vi "TI sbRIO Main (RT).vi"() -> ()   [LabVIEW 2013]
uses:
  Type Defs/Restarts Cluster.ctl
  Type Defs/Restarts Limits.ctl
  Type Defs/Controller Names.ctl
  Controls/HMI Mom Buttons.ctl
  Controls/Alarm Config.ctl
  Controls/Alarm Definition.ctl
  Controls/Alarm Profile Config.ctl
  Type Defs/App Config.ctl
  Type Defs/Actual Starts.ctl
  Type Defs/Sequence States.ctl
  Type Defs/CAN Mode.ctl
  Type Defs/Controller List.ctl
  Controls/RPi HMI Mode.ctl
  Type Defs/Pump Data Mode.ctl
  Controls/HMI Tog Buttons.ctl
  Controls/Controller Config.ctl
  SubVIs/TenHzDataArray(Global).vi
  <vilib>/FPGAPlugInAG/sbRIO-9626/niLvFpga_Open_sbRIO-9626.vi
  <vilib>/Utility/file.llb/Write To Spreadsheet File (DBL).vi
  SubVIs/Record Period (global).vi
  SubVIs/Record Samples (global).vi
  <vilib>/FPGAPlugInAG/sbRIO-9626/niLvFpga_Reset_sbRIO-9626.vi
  <vilib>/Utility/error.llb/Error Cluster From Error Code.vi
  <vilib>/rvi/errors/niLvFpgaAdjustHostInterfaceError.vi
  <vilib>/FPGAPlugInAG/sbRIO-9626/niLvFpga_Run_sbRIO-9626.vi
  <vilib>/Utility/file.llb/Write To Spreadsheet File (string).vi
  <vilib>/rvi/interface/nirviOpenFPGA/nirviOpenFPGA.xnode
  Controls/FPGA_Reference.ctl
  FPGA/bitfiles/TI sbRIO PWM (FPGA) v1.0.lvbitx
  <vilib>/rvi/interface/nirviMethod/nirviMethod.xnode
  <vilib>/rvi/interface/nirviReadWriteControl/nirviReadWriteControl.xnode
  <vilib>/Utility/config.llb/NI_LVConfig.lvlib
  NiFpgaLv.dll
  <vilib>/NI_Real-Time Target Support.lvlib
  Real-Time/Controls/RT FIFO Mode.ctl
  <vilib>/rvi/interface/nirviCloseFPGA/nirviCloseFPGA.xnode
  Type Defs/JSON_Channel.ctl
  Type Defs/JSON_Pump.ctl
  Type Defs/JSON_Tank.ctl
  <vilib>/rvi/errors/niLvFpgaMergeErrorWithErrorCode.vi
  <vilib>/FPGAPlugInAG/sbRIO-9626/niLvFpga_Abort_sbRIO-9626.vi
  <vilib>/FPGAPlugInAG/sbRIO-9626/niLvFpga_Close_sbRIO-9626.vi
panel:
  out "HMI Mom Buttons":T1
  out "TenHzPts":i32
  in  "TenHz Path":path=path "u:/TenHz/Try.csv"
  in  "Stop":bool
  in  "Alarm Tab":enum32{"Page 1", "Page 2"}(tab)
  out "Alarm Message":string
  in  "pb.Alarm OK":bool
  in  "Monitoring Tab":enum32{"Page 1", "Page 2"}(tab)
  in  "pb.E Stop":bool
  in  "Ignition Relay":T2
  in  "Power Relay":T2
  out "Voltages":dbl[](array[numeric])=[0.015201568603515625, 0.00335693359375, 0.003021240234375, 0.12260055541992188, 0.06085968017578125, 0.052234649658203125] caption="Pump\nVoltage\n(V)" format="%#.0f"
  out "Ave. Speed":dbl=7.74131899555212 format="%.1f"
  out "Temp2":dbl caption="Tank 2 Temp (C):" format="%#_2g"
  out "Temp1":dbl caption="Tank 1 Temp (C):" format="%#_2g"
  out "Pressure":dbl[](array[numeric])=[0.015201568603515625, 0.00335693359375, 0.003021240234375, 0.12260055541992188, 0.06085968017578125, 0.052234649658203125] caption="Pressure\n(kPa)" format="%#.0f"
  out "Flow":dbl[](array[numeric])=[0.0, 0.0, 0.0, 0.125, 0.0625, 0.0625] caption="Flow\n(L/H)" format="%#.0f"
  out "PumpCurrent":dbl[](array[numeric])=[0.015201568603515625, 0.00335693359375, 0.003021240234375, 0.12260055541992188, 0.06085968017578125, 0.052234649658203125] caption="Pump\nCurrent\n(RMS)" format="%#.1g"
  out "PS Actual (V):":dbl format="%.2f"
  out "ControllerCurrent":dbl[](array[numeric])=[0.015201568603515625, 0.00335693359375, 0.003021240234375, 0.12260055541992188, 0.06085968017578125, 0.052234649658203125] caption="Controller\nCurrent\n(DC)" format="%#.1g"
  out "Speed":dbl[](array[numeric]) caption="Speed\n(RPM)" format="%#_4f"
  in  "Power Supply Cmd (V):":dbl min=0.0 max=20.0 format="%#.2f"
  in  "PressureCMD":dbl caption="Pressure Cmd (kPa):" min=0.0 max=825.0 format="%#.2f"
  in  "Manual\nCMD":dbl[](array[numeric])=[0.0, 0.0, 0.0, 0.0, 0.0, 0.0] min=0.0 max=100.0 step=0.1 format="%#.2f"
  in  "pb.Zero CMDs":bool
  out "CPU Usage:":dbl=7.74131899555212 format="%.1f"
  in  "Pumps Present":T2={"Pump 1"=TRUE, "Pump 2"=TRUE, "Pump 3"=TRUE, "Pump 4"=TRUE, "Pump 5"=TRUE, "Pump 6"=TRUE}
  out "CAN CMD":dbl
  in  "Restarts Tab":enum32{"Page 1", "Page 2"}(tab)
  in  "Restarts Limits":T3={"High Limits:"=[30, 30, 30, 30, 30, 30], "Low Limits:"=[30, 30, 30, 30, 30, 30]}
  in  "pb.Rst Tot Restarts":bool
  in  "pb.Reset Restarts":bool
  in  "Inform:":string="Input email address on Email Handler program on Lab 4 PC."
  out "Restarts Cluster":T4
  out "Client?":bool
  in  "Title Tab":enum32{"Page 1", "Page 2"}(tab)
  in  "Title":string="TI Automotive sbRIO, v2.6 (Standard Tank)"
  in  "Login":bool
  in  "Set Time Tab":enum32{"Page 1", "Page 2"}(tab)
  in  "pb.Set Time OK":bool
  in  "pb.Set Time Cancel":bool
  in  "New Time":dbl format="%<%H:%M:%S>t"
  in  "Reset Tab":enum32{"Page 1", "Page 2"}(tab)
  in  "pb.Reset OK":bool
  in  "pb.Reset Cancel":bool
  in  "pb.Stop Profile":bool
  in  "Save As Tab":enum32{"Page 1", "Page 2"}(tab)
  in  "New Profile Name:":string
  in  "pb.Save As OK":bool
  in  "pb.Save As Cancel":bool
  in  "Main Tab":enum32{"Main", "Data Stream", "Alarms"}(tab)
  in  "Profile:":string[][](table)=[["1", "2.0", "0.0", "0.0", "0.0", "67.6", "67.6", "67.6"], ["2", "1.0", "0.0", "0.0", "0.0", "10.0", "10.0", "10.0"]]
  in  "Controller Type:":T5
  in  "pb.FuelChange":bool
  in  "Tank 1 Fuel Type":string
  in  "Tank 2 Fuel Type":string
  in  "Stagger Time (ms):":i32
  in  "pb.Time Reset All":bool
  in  "CA Number:":string
  in  "Profile Name:":string(combo)="test"
  in  "pb.Save As":bool
  out "Current Step:":i32=2
  out "Step Time Left:":dbl=0.21101045608520508
  out "Cycles Completed:":u32=17
  in  "pb.Cycle Reset":bool
  out "Location:":string
  in  "pb.Run Profile":bool
  out "Elapsed Time:":dbl[](array[numeric])=[7.1, 7.1, 7.1, 458133.45, 458138.85000000003, 458126.75] format="%<%H:%M:%S>t"
  in  "pb.Resets":bool[](array[boolean])=[FALSE, FALSE, FALSE, FALSE, FALSE, FALSE]
  in  "pb.Sets":bool[](array[boolean])=[FALSE, FALSE, FALSE, FALSE, FALSE, FALSE]
  in  "Serial Numbers":T6
  in  "pb.TenHzSave":bool
  in  "Record Frequency:":i32=10 min=1 max=10 step=1
  in  "pb.Reset Cogs":bool
  in  "Cog Limits:":i32[](array[numeric])=[30, 30, 30, 30, 30, 30] min=0
  out "Cog Events:":i32[](array[numeric])
  out "Graph":dbl[](graph)
  in  "RPMhyst":fxp<+,25,6>=0.20000076293945312
  in  "Alarm Config":T7
  # "Manual Control"
  # "Monitoring"
  # "Restarts Monitor"
  # "Enter a new elapsed time."
  # "Are you sure you want to reset?"
  # "Under Development"
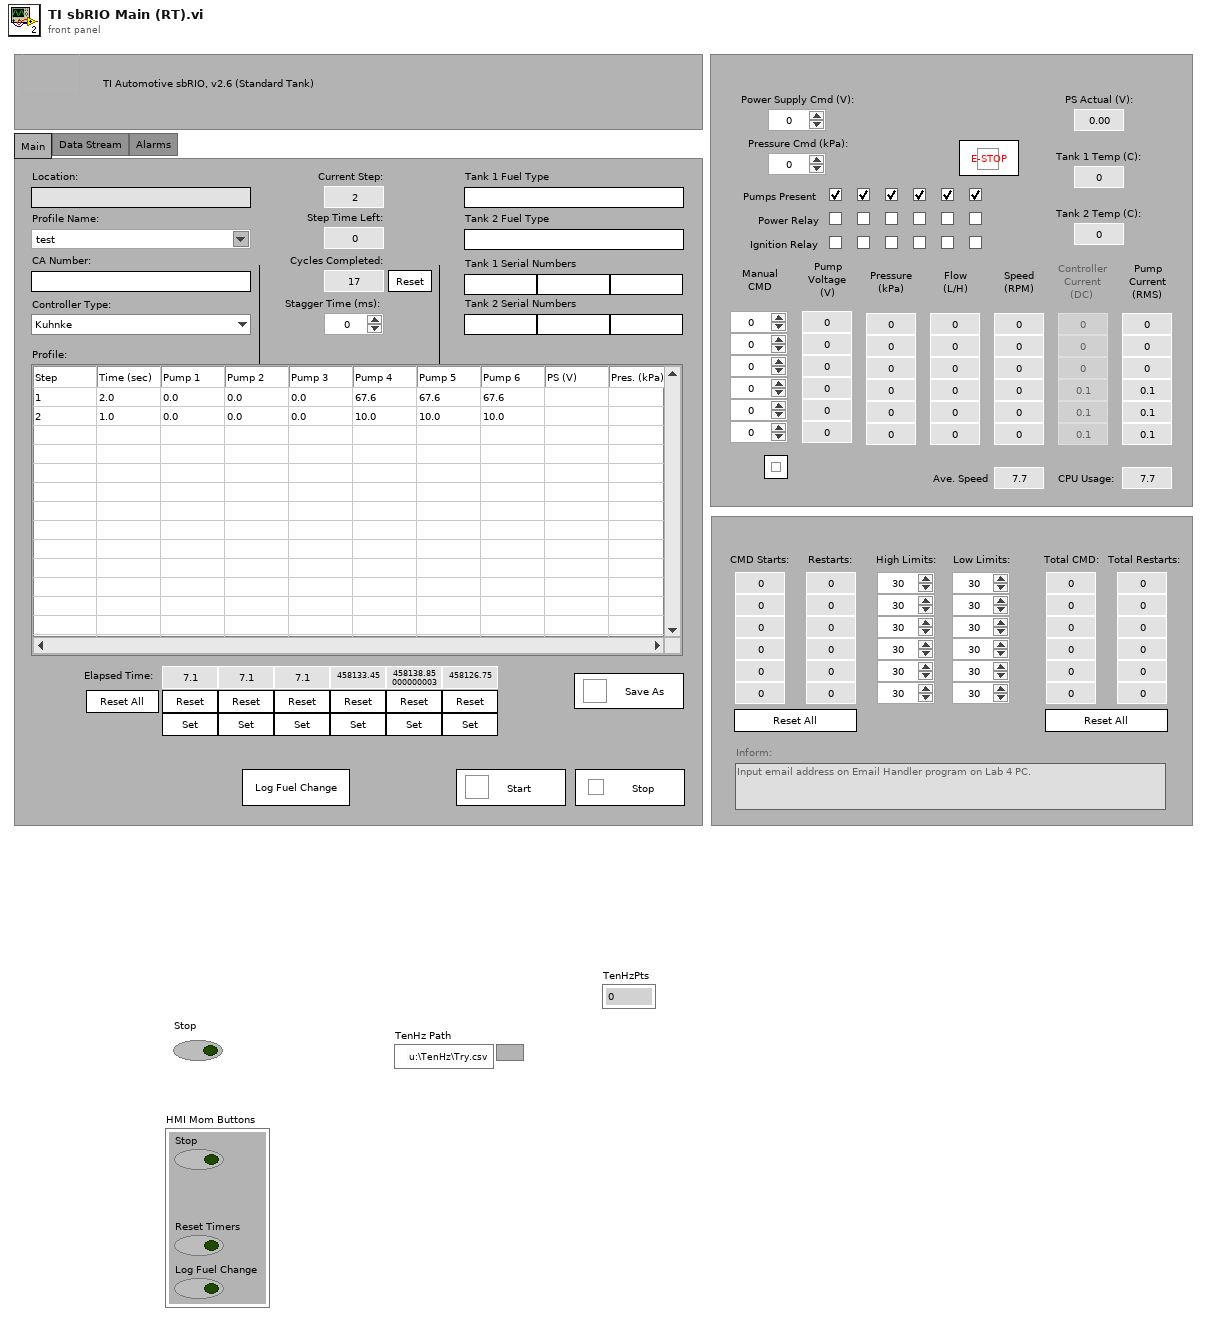
[diagram p1: front panel]
types:
  T1 = typedef "HMI Mom Buttons.ctl" = cluster{"Stop":bool, "Reset Timers":bool, "Log Fuel Change":bool}
  T2 = cluster{"Pump 1":bool, "Pump 2":bool, "Pump 3":bool, "Pump 4":bool, "Pump 5":bool, "Pump 6":bool}
  T3 = typedef "Restarts Limits.ctl" = cluster{"High Limits:":i32[], "Low Limits:":i32[]}
  T4 = typedef "Restarts Cluster.ctl" = cluster{"CMD Starts:":i32[], "Restarts:":i32[], "Total CMD:":i32[], "Total Restarts:":i32[]}
  T5 = typedef "Controller Names.ctl" = enum16{"Kuhnke", "Conti", "Hella CAN", "Helbako", "TI PWM", "PSA", "Hella DC Gas", "Hella DC Diesel", "8 Comm", "10 Comm", "8 Comm Hella", "10 Comm Hella", "8 Comm Omron", "10 Comm Omron", "8 Comm Nissan", "10 Comm Nissan"}
  T6 = cluster{"Position 1 SN":string, "Position 2 SN":string, "Position 3 SN":string, "Position 4 SN":string, "Position 5 SN":string, "Position 6 SN":string}
  T7 = typedef "Alarm Config.ctl" = cluster{"Alarms:":T8[], "Profile Sync:":T9}
  T8 = typedef "Alarm Definition.ctl" = cluster{"Description:":string, "Enabled:":bool, "Data Index:":i32, "Data Type:":string, "Low Limit:":dbl, "High Limit:":dbl, "Trip Time:":u32, "Profile Sync:":bool}
  T9 = typedef "Alarm Profile Config.ctl" = cluster{"Trip Time:":u32, "Consecutive Trips:":i32}
  T10 = typedef "RPi HMI Mode.ctl" = enum16{"Init", "Write Data", "Read from RPi", "Write to RPi"}
  T11 = typedef "Controller List.ctl" = cluster{"Controller Name":T5, "CommSeg":i32, "PWM?":bool, "Frequency":i32, "Low Command":dbl, "High Command":dbl, "Stop Command":dbl, "Command Step":dbl, "Solenoid Stop?":bool, "Controller?":bool, "Invert PWM":bool}[]
  T12 = cluster{"Controller Name":T5, "CommSeg":i32, "PWM?":bool, "Frequency":i32, "Low Command":dbl, "High Command":dbl, "Stop Command":dbl, "Command Step":dbl, "Solenoid Stop?":bool, "Controller?":bool, "Invert PWM":bool}
  T13 = typedef "CAN Mode.ctl" = enum16{"Init", "Read", "Write", "Close"}
  T14 = typedef "Sequence States.ctl" = enum16{"Main", "Init Files", "Init", "Save As", "Start Profile", "Check Step Time", "Alarm", "Run Step", "Stop Profile", "Cycle Reset", "Time Reset", "Time Reset All", "Time Set", "Tare CTs", "Save Profile", "Open Profile", "Get Profiles", "Update Screen", "Save Status", "Set Manual CMD", "Reset Restarts", "Reset Total Restarts", "Reset Cogs", "Disable Background", "Enable Background", "Get/Release Control", "Init AKLH", "Save AKLH", "Log Fuel Change", "Update Data Stream", "Init TenHz", "Read TenHz", "Remote Timer Reset", "Record Frequency Change", "Controller Change", "Get Alarms", "Init Alarms", "Save Alarms"}
  T15 = typedef "Actual Starts.ctl" = cluster{"Actual Pump Starts":i32[], "Initial Actual Starts":i32[], "Tot Act Starts":i32[], "Tot Init Act Starts":i32[]}
  T16 = typedef "App Config.ctl" = cluster{"Location":string, "Profiles Path":path, "Current Profile":string, "CA Number":string, "Cycles Completed":u32, "PWM Freq (Hz)":dbl, "Controller Type:":T5, "Inform":string, "Pumps Present":u32, "Stagger Time (ms)":i32, "Tank 1 Fuel":string, "Tank 2 Fuel":string, "Serial Numbers":cluster{"Position 1 SN":string, "Position 2 SN":string, "Poaition 3 SN":string, "Position 4 SN":string, "Position 5 SN":string, "Position 6 SN":string}, "Record TenHz":bool, "VoltCtrlRef":string, "TenHzFrequency":u32}
  T17 = cluster{"Error":errorcluster, "Profile":string[][], "App Config":T16, "Profiles":string[], "Current Step":i32, "Step Time Left":dbl, "Run Profile":bool, "Step Start Time":dbl, "Step Time":dbl, " # of Steps":i32, "Last Update":dbl, "Update Screen":bool, "Last Profile Time":dbl, "Manual CMDs":dbl[], "Client?":bool, "pb.Run Profile":bool, "pb.Resets":bool[], "pb.Sets":bool[], "Last CMDs":dbl[], "Update Profile":bool, "Elapsed Times":dbl[], "Intitial Times":dbl[], "Alarm":bool, "CT Offsets":fxp<+/-,26,7>[], "Pumps Present":cluster{"Pump 1":bool, "Pump 2":bool, "Pump 3":bool, "Pump 4":bool, "Pump 5":bool, "Pump 6":bool}, "Login":bool, "Stagger Counter":i32, "New Step":bool, "Restarts Limits":T3, "Restarts Cluster":T4, "Actual Starts":T15, "AKLH Path":path, "TenHz Path":path, "AKLH Timer":dbl, "TenHz Timer":dbl, "TenHz Active?":bool, "AKLH Last Hour":i32, "Main Tab":enum32{"Page 1", "Page 2"}, "Stop Cmd":dbl, "Tank Data":dbl[], "CogCounters":i32[], "Cog Events":i32[], "Voltage Enable":bool, "Cog Limits:":i32[], "TenHz Day":i32, "Controller":cluster{"Controller Name":T5, "CommSeg":i32, "PWM?":bool, "Frequency":i32, "Low Command":dbl, "High Command":dbl, "Stop Command":dbl, "Command Step":dbl, "Solenoid Stop?":bool, "Controller?":bool, "Invert PWM":bool}, "PS CMD":dbl, "Press CMD":dbl, "Temp CMD":dbl, "Power Relay":cluster{"Pump 1":bool, "Pump 2":bool, "Pump 3":bool, "Pump 4":bool, "Pump 5":bool, "Pump 6":bool}, "Ignition Relay":cluster{"Pump 1":bool, "Pump 2":bool, "Pump 3":bool, "Pump 4":bool, "Pump 5":bool, "Pump 6":bool}, "Controller List":T11, "Alarm Config":T7, "Alarm Config Path":path, "Trip Counters":i32[], "Previous Times":u32[], "Alarm Message":string, "Restart Alarm":bool, "Prev ON Times":u32[]}
  T18 = typedef "FPGA_Reference.ctl" = refnum<k20>
  T19 = typedef "HMI Cluster.ctl" = cluster{"Error":errorcluster, "COM Ref":refnum<visa-resource-name>, "Pump Data":T20, "Tank Data":cluster{"PS Actual (V):":dbl, "Temp1":dbl, "Temp2":dbl}, "Power Relays":cluster{"Pump 1":bool, "Pump 2":bool, "Pump 3":bool, "Pump 4":bool, "Pump 5":bool, "Pump 6":bool}, "Pump CMDs":dbl[], "HMI Header":T21, "Tank CMDs":T22, "HMI Tog Buttons":T23, "In Test":bool, "HMI Command":bool, "HMI Mom Buttons":T1, "Controller Config":T24}
  T20 = typedef "Pump Data.ctl" = cluster{"Voltages":dbl[], "PumpCurrent":dbl[], "Speed":dbl[], "ControllerCurrent":dbl[], "Pressure":dbl[], "Flow":dbl[], "Elapsed Time:":dbl[]}
  T21 = typedef "HMI Header.ctl" = cluster{"Line 1":string, "Line 2":string, "Line 3":string}
  T22 = typedef "Tank CMDs.ctl" = cluster{"PS CMD":dbl, "Press CMD":dbl, "Temp CMD":dbl}
  T23 = typedef "HMI Tog Buttons.ctl" = cluster{"Start Test":bool, "Toggle Spare 1":bool, "Toggle Spare 2":bool, "Toggle Spare 3":bool, "Toggle Spare 4":bool, "Toggle Spare 5":bool}
  T24 = typedef "Controller Config.ctl" = cluster{"Controller List":string, "Controller Type:":T5, "CMD Max":i32, "CMD Inc":i32}
  T25 = typedef "RT FIFO Mode.ctl" = enum16{"Create", "Write", "Read", "Delete"}
  T26 = typedef "Pump Data Mode.ctl" = enum16{"Read", "Write Data", "Write Cal"}
  T27 = enum8{"Enabled", "Disabled", "Disabled and Grayed Out"}
  T28 = typedef "JSON_Tank.ctl" = cluster{"number":u16, "building":string, "room":string, "ipAddress":string, "profileName":string, "caNumber":string, "ctrlType":string, "mode":string, "channels":T29[], "pumps":T30[]}
  T29 = typedef "JSON_Channel.ctl" = cluster{"name":string, "tag":string, "data":string, "type":string, "unit":string}
  T30 = typedef "JSON_Pump.ctl" = cluster{"position":u8, "enabled":bool, "command":string, "channels":T29[], "elapsedTime":string}
  T31 = cluster{"Position 1 SN":string, "Position 2 SN":string, "Poaition 3 SN":string, "Position 4 SN":string, "Position 5 SN":string, "Position 6 SN":string}
  T32 = typedef "Test Action.ctl" = enum16{"Idle", "Start", "Stop", "Pump Cmd", "Pump 1 Enable", "Pump 2 Enable", "Pump 3 Enable", "Pump 4 Enable", "Pump 5 Enable", "Pump 6 Enable", "Timer 1 Reset", "Timer 2 Reset", "Timer 3 Reset", "Timer 4 Reset", "Timer 5 Reset", "Timer 6 Reset"}
  T33 = cluster{"Boolean array[0]":bool, "Boolean array[1]":bool, "Boolean array[2]":bool, "Boolean array[3]":bool, "Boolean array[4]":bool, "Boolean array[5]":bool}
  T34 = typedef "LVDateTimeRec.ctl" = cluster{"fractional second":dbl, "second":i32, "minute":i32, "hour":i32, "day of month":i32, "month":i32, "year":i32, "day of week":i32, "day of year":i32, "DST":i32}
  T35 = typedef "NI_LVConfig.lvlib/Config Data RefNum.ctl" = refnum<k1>
  T36 = cluster{"PS Actual (V):":dbl, "Temp1":dbl, "Temp2":dbl}
  T37 = cluster{"Location":string, "Current Profile":string, "CA Number":string}
  T38 = cluster{"PS CMD":dbl, "Press CMD":dbl, "Temp CMD":dbl}
  T39 = typedef "LVRemotePanelConnectionsTypeDef.ctl" = cluster{"VI Name":string, "Remote":string, "UserName":string, "Port":i32, "Status":enum32{"Viewing", "Waiting For Control", "Controlling"}, "Create Time":timestamp, "Status Time":timestamp, "Control End Time":timestamp}[]
  T40 = typedef "NI_Real-Time Target Support.lvlib/RT CPU Load.ctl" = cluster{"Total (%)":dbl, "Time Critical (%)":dbl, "Timed Structures (%)":dbl, "High (%)":dbl, "Above Normal (%)":dbl, "Normal (%)":dbl, "Background (%)":dbl, "Idle (%)":dbl, "ISR (%)":dbl}
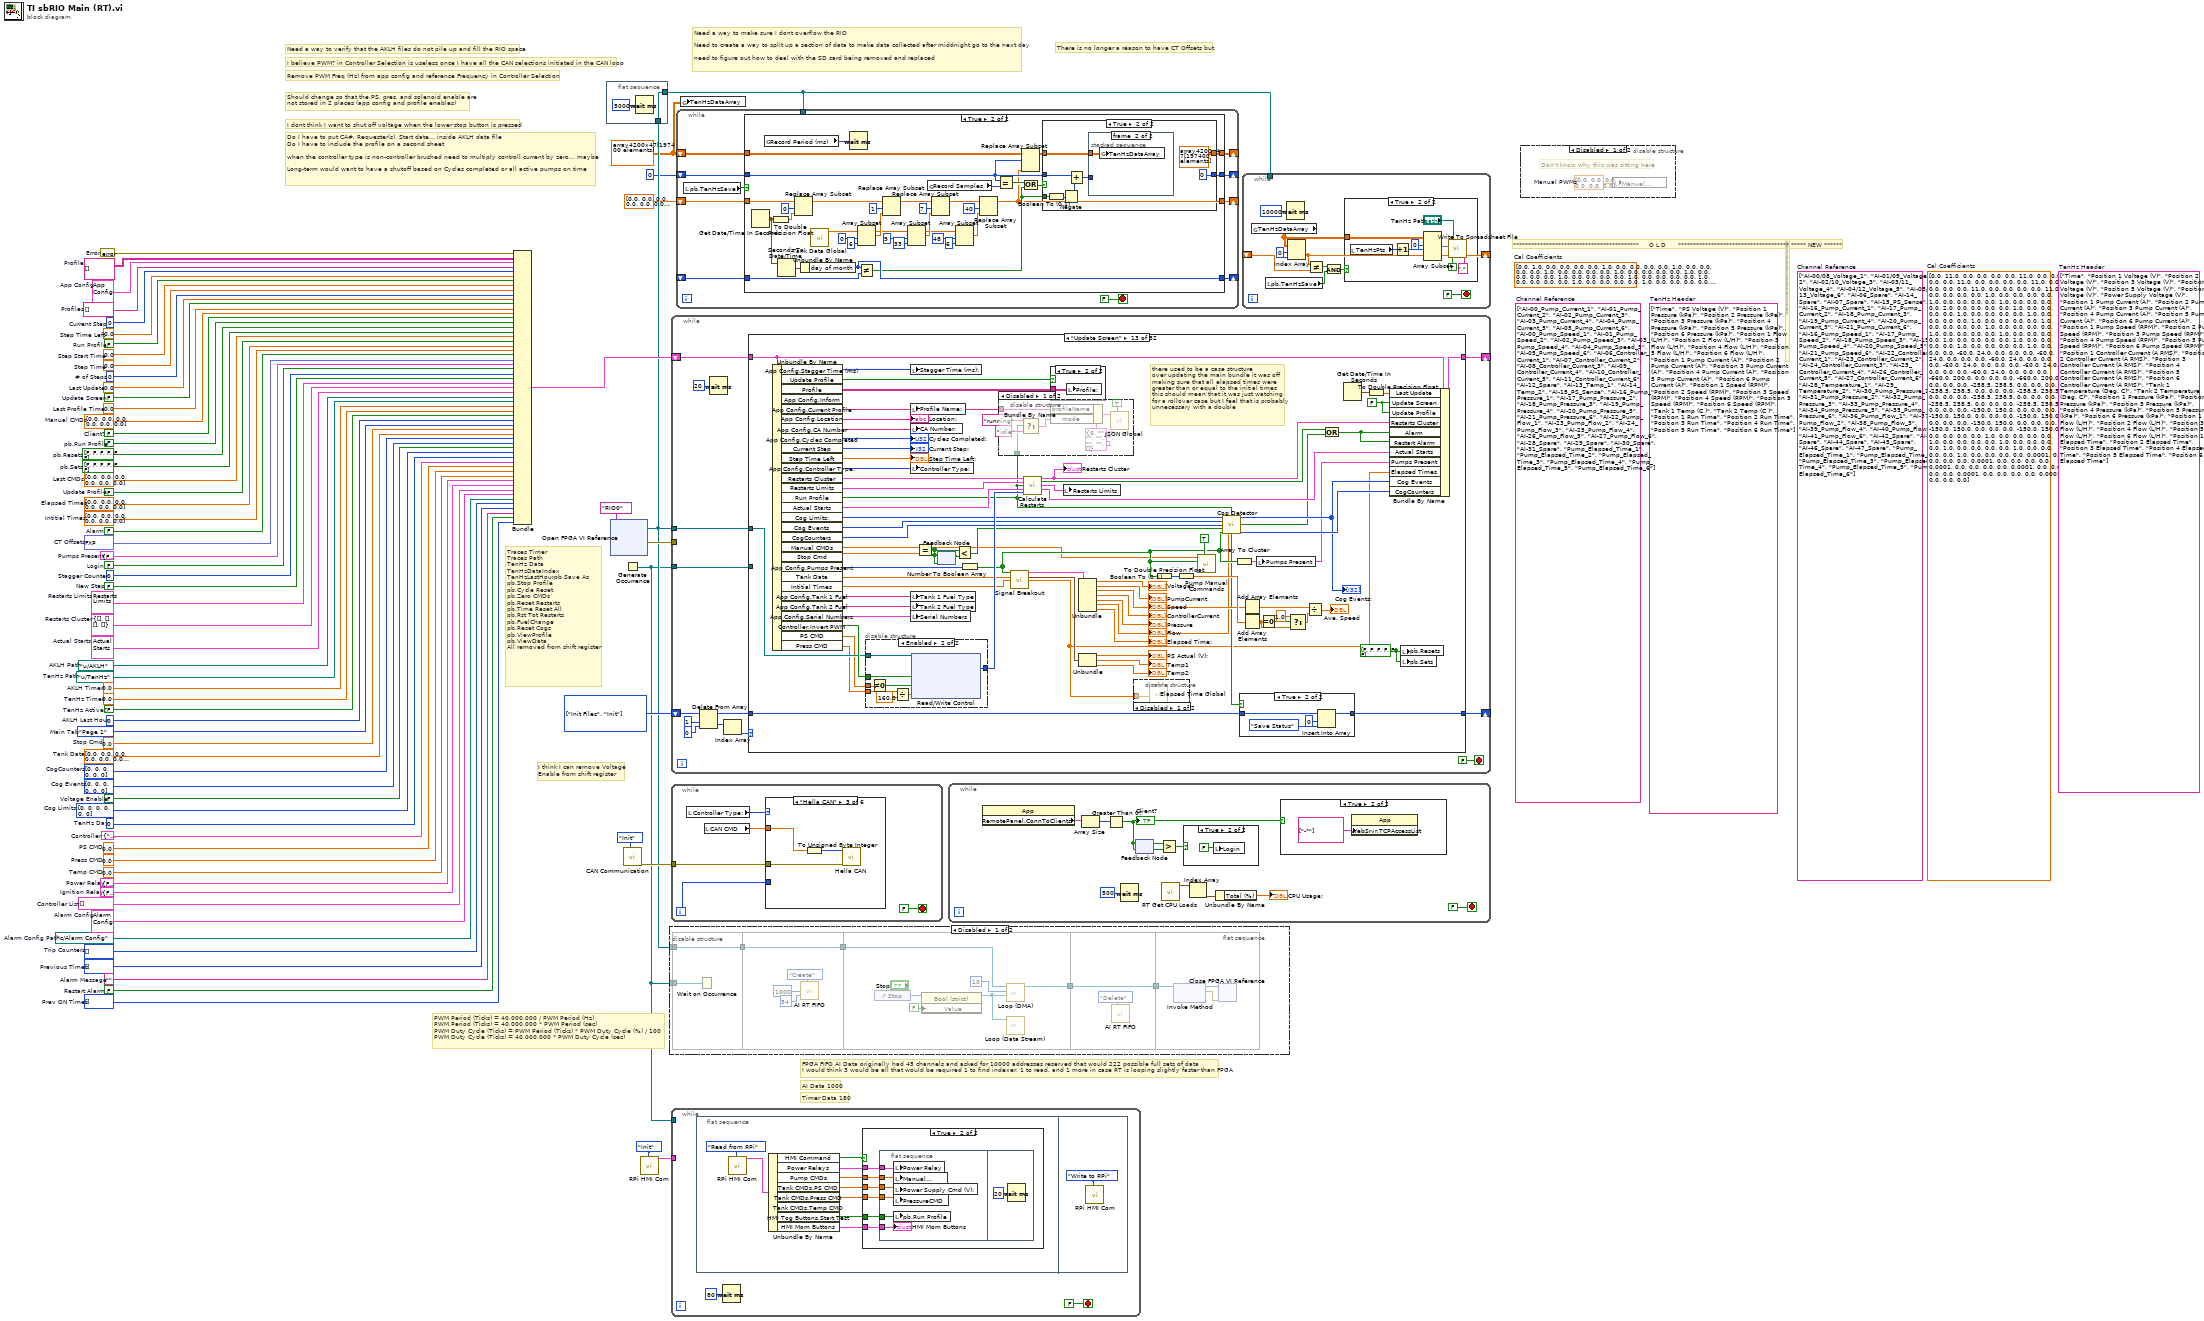
[diagram p0: block diagram]
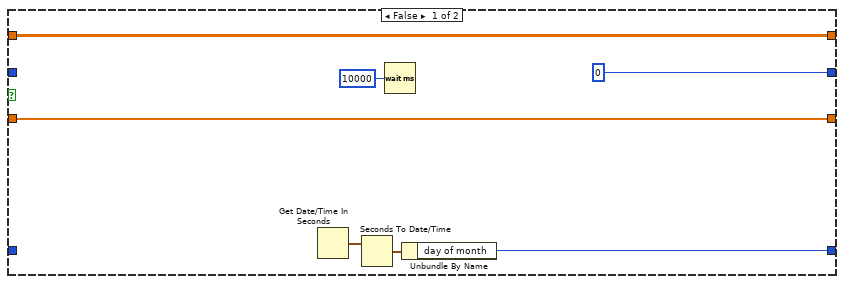
[diagram p3: hidden frame]
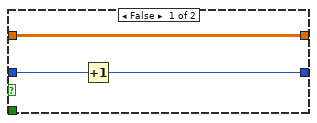
[diagram p4: hidden frame]
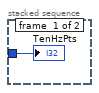
[diagram p5: hidden frame]
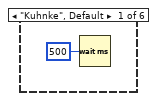
[diagram p8: hidden frame]
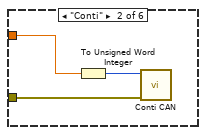
[diagram p9: hidden frame]
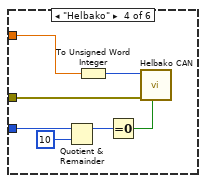
[diagram p10: hidden frame]
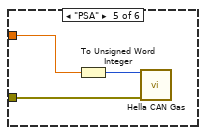
[diagram p11: hidden frame]
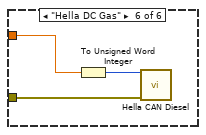
[diagram p12: hidden frame]
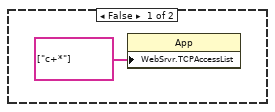
[diagram p13: hidden frame]
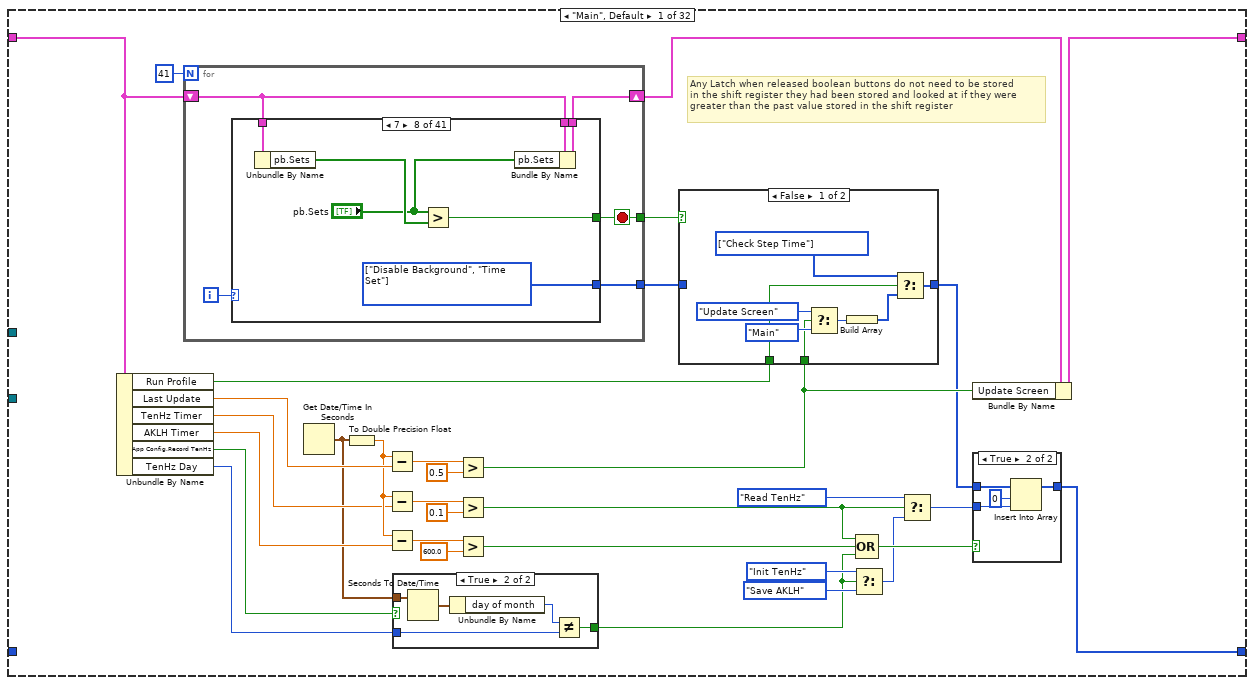
[diagram p16: hidden frame]
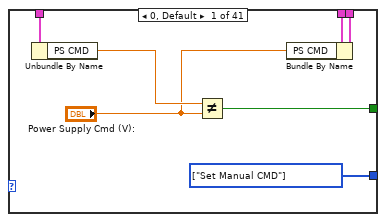
[diagram p19: hidden frame]
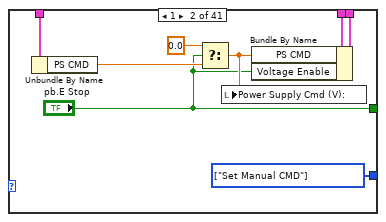
[diagram p20: hidden frame]
diagram:
  w1 = dbl[][] array4200x47[197400 elements]
  w7 = u32[] []  # Prev ON Times
  w8 = FALSE  # Restart Alarm
  w9 = ""  # Alarm Message
  w10 = u32[] []  # Previous Times
  w11 = i32[] []  # Trip Counters
  w12 = path "c:/Alarm Config"  # Alarm Config Path
  w13 = T7 {"Alarms:"=[{"Description:"="", "Enabled:"=FALSE, "Data Index:"=0, "Data Type:"="", "Low Limit:"=0.0, "High Limit:"=0.0, "Trip Time:"=0, "Profile Sync:"=FALSE}, {"Description:"="", "Enabled:"=FALSE, "Data Index:"=0, "Data Type:"="", "Low Limit:"=0.0, "High Limit:"=0.0, "Trip Time:"=0, "Profile Sync:"=FALSE}, {"Description:"="", "Enabled:"=FALSE, "Data Index:"=0, "Data Type:"="", "Low Limit:"=0.0, "High Limit:"=0.0, "Trip Time:"=0, "Profile Sync:"=FALSE}, {"Description:"="", "Enabled:"=FALSE, "Data Index:"=0, "Data Type:"="", "Low Limit:"=0.0, "High Limit:"=0.0, "Trip Time:"=0, "Profile Sync:"=FALSE}, {"Description:"="", "Enabled:"=FALSE, "Data Index:"=0, "Data Type:"="", "Low Limit:"=0.0, "High Limit:"=0.0, "Trip Time:"=0, "Profile Sync:"=FALSE}, {"Description:"="", "Enabled:"=FALSE, "Data Index:"=0, "Data Type:"="", "Low Limit:"=0.0, "High Limit:"=0.0, "Trip Time:"=0, "Profile Sync:"=FALSE}, {"Description:"="", "Enabled:"=FALSE, "Data Index:"=0, "Data Type:"="", "Low Limit:"=0.0, "High Limit:"=0.0, "Trip Time:"=0, "Profile Sync:"=FALSE}, {"Description:"="", "Enabled:"=FALSE, "Data Index:"=0, "Data Type:"="", "Low Limit:"=0.0, "High Limit:"=0.0, "Trip Time:"=0, "Profile Sync:"=FALSE}], "Profile Sync:"={"Trip Time:"=0, "Consecutive Trips:"=0}}  # Alarm Config
  w14 = T11 []  # Controller List
  w15 = T12 {"Controller Name"=enum."Kuhnke", "CommSeg"=2, "PWM?"=TRUE, "Frequency"=100, "Low Command"=10.0, "High Command"=100.0, "Stop Command"=10.0, "Command Step"=0.1, "Solenoid Stop?"=FALSE, "Controller?"=TRUE, "Invert PWM"=FALSE}  # Controller
  w17 = T2 {"Pump 1"=FALSE, "Pump 2"=FALSE, "Pump 3"=FALSE, "Pump 4"=FALSE, "Pump 5"=FALSE, "Pump 6"=FALSE}  # Ignition Relay
  w18 = T2 {"Pump 1"=FALSE, "Pump 2"=FALSE, "Pump 3"=FALSE, "Pump 4"=FALSE, "Pump 5"=FALSE, "Pump 6"=FALSE}  # Power Relay
  w19 = 0.0  # Temp CMD
  w20 = 0.0  # Press CMD
  w21 = 0.0  # PS CMD
  (unwired) string[] ["Time", "Position 1 Voltage (V)", "Position 2 Voltage (V)", "Position 3 Voltage (V)", "Position 4 Voltage (V)", "Position 5 Voltage (V)", "Position 6 Voltage (V)", "Power Supply Voltage (V)", "Position 1 Pump Current (A)", "Position 2 Pump Current (A)", "Position 3 Pump Current (A)", "Position 4 Pump Current (A)", "Position 5 Pump Current (A)", "Position 6 Pump Current (A)", "Position 1 Pump Speed (RPM)", "Position 2 Pump Speed (RPM)", "Position 3 Pump Speed (RPM)", "Position 4 Pump Speed (RPM)", "Position 5 Pump Speed (RPM)", "Position 6 Pump Speed (RPM)", "Position 1 Controller Current (A RMS)", "Position 2 Controller Current (A RMS)", "Position 3 Controller Current (A RMS)", "Position 4 Controller Current (A RMS)", "Position 5 Controller Current (A RMS)", "Position 6 Controller Current (A RMS)", "Tank 1 Temperature (Deg. C)", "Tank 2 Temperature (Deg. C)", "Position 1 Pressure (kPa)", "Position 2 Pressure (kPa)", "Position 3 Pressure (kPa)", "Position 4 Pressure (kPa)", "Position 5 Pressure (kPa)", "Position 6 Pressure (kPa)", "Position 1 Flow (L/H)", "Position 2 Flow (L/H)", "Position 3 Flow (L/H)", "Position 4 Flow (L/H)", "Position 5 Flow (L/H)", "Position 6 Flow (L/H)", "Position 1 Elapsed Time", "Position 2 Elapsed Time", "Position 3 Elapsed Time", "Position 4 Elapsed Time", "Position 5 Elapsed Time", "Position 6 Elapsed Time"]  # TenHz Header
  (unwired) dbl[][] [[0.0, 11.0, 0.0, 0.0, 0.0], [0.0, 11.0, 0.0, 0.0, 0.0], [0.0, 11.0, 0.0, 0.0, 0.0], [0.0, 11.0, 0.0, 0.0, 0.0], [0.0, 11.0, 0.0, 0.0, 0.0], [0.0, 11.0, 0.0, 0.0, 0.0], [0.0, 1.0, 0.0, 0.0, 0.0], [0.0, 1.0, 0.0, 0.0, 0.0], [0.0, 1.0, 0.0, 0.0, 0.0], [0.0, 2.0, 0.0, 0.0, 0.0], [0.0, 1.0, 0.0, 0.0, 0.0], [0.0, 1.0, 0.0, 0.0, 0.0], [0.0, 1.0, 0.0, 0.0, 0.0], [0.0, 1.0, 0.0, 0.0, 0.0], [0.0, 1.0, 0.0, 0.0, 0.0], [0.0, 1.0, 0.0, 0.0, 0.0], [0.0, 1.0, 0.0, 0.0, 0.0], [0.0, 1.0, 0.0, 0.0, 0.0], [0.0, 1.0, 0.0, 0.0, 0.0], [0.0, 1.0, 0.0, 0.0, 0.0], [0.0, 1.0, 0.0, 0.0, 0.0], [0.0, 1.0, 0.0, 0.0, 0.0], [-60.0, 24.0, 0.0, 0.0, 0.0], [-60.0, 24.0, 0.0, 0.0, 0.0], [-60.0, 24.0, 0.0, 0.0, 0.0], [-60.0, 24.0, 0.0, 0.0, 0.0], [-60.0, 24.0, 0.0, 0.0, 0.0], [-60.0, 24.0, 0.0, 0.0, 0.0], [-660.0, 200.0, 0.0, 0.0, 0.0], [-660.0, 200.0, 0.0, 0.0, 0.0], [-258.5, 258.5, 0.0, 0.0, 0.0], [-258.5, 258.5, 0.0, 0.0, 0.0], [-258.5, 258.5, 0.0, 0.0, 0.0], [-258.5, 258.5, 0.0, 0.0, 0.0], [-258.5, 258.5, 0.0, 0.0, 0.0], [-258.5, 258.5, 0.0, 0.0, 0.0], [-150.0, 150.0, 0.0, 0.0, 0.0], [-150.0, 150.0, 0.0, 0.0, 0.0], [-150.0, 150.0, 0.0, 0.0, 0.0], [-150.0, 150.0, 0.0, 0.0, 0.0], [-150.0, 150.0, 0.0, 0.0, 0.0], [-150.0, 150.0, 0.0, 0.0, 0.0], [0.0, 1.0, 0.0, 0.0, 0.0], [0.0, 1.0, 0.0, 0.0, 0.0], [0.0, 1.0, 0.0, 0.0, 0.0], [0.0, 1.0, 0.0, 0.0, 0.0], [0.0, 1.0, 0.0, 0.0, 0.0], [0.0, 1.0, 0.0, 0.0, 0.0], [0.0, 0.0001, 0.0, 0.0, 0.0], [0.0, 0.0001, 0.0, 0.0, 0.0], [0.0, 0.0001, 0.0, 0.0, 0.0], [0.0, 0.0001, 0.0, 0.0, 0.0], [0.0, 0.0001, 0.0, 0.0, 0.0], [0.0, 0.0001, 0.0, 0.0, 0.0]]  # Cal Coefficients
  (unwired) dbl[][] [[0.0, 1.0, 0.0, 0.0, 0.0], [0.0, 1.0, 0.0, 0.0, 0.0], [0.0, 1.0, 0.0, 0.0, 0.0], [0.0, 1.0, 0.0, 0.0, 0.0], [0.0, 1.0, 0.0, 0.0, 0.0], [0.0, 1.0, 0.0, 0.0, 0.0], [0.0, 1.0, 0.0, 0.0, 0.0], [0.0, 1.0, 0.0, 0.0, 0.0], [0.0, 1.0, 0.0, 0.0, 0.0], [0.0, 1.0, 0.0, 0.0, 0.0], [0.0, 1.0, 0.0, 0.0, 0.0], [0.0, 1.0, 0.0, 0.0, 0.0], [-60.0, 24.0, 0.0, 0.0, 0.0], [-60.0, 24.0, 0.0, 0.0, 0.0], [-60.0, 24.0, 0.0, 0.0, 0.0], [-60.0, 24.0, 0.0, 0.0, 0.0], [-60.0, 24.0, 0.0, 0.0, 0.0], [-60.0, 24.0, 0.0, 0.0, 0.0], [0.0, 1.0, 0.0, 0.0, 0.0], [-660.0, 200.0, 0.0, 0.0, 0.0], [-660.0, 200.0, 0.0, 0.0, 0.0], [0.0, 2.0, 0.0, 0.0, 0.0], [-258.5, 258.5, 0.0, 0.0, 0.0], [-258.5, 258.5, 0.0, 0.0, 0.0], [-258.5, 258.5, 0.0, 0.0, 0.0], [-258.5, 258.5, 0.0, 0.0, 0.0], [-258.5, 258.5, 0.0, 0.0, 0.0], [-258.5, 258.5, 0.0, 0.0, 0.0], [-150.0, 150.0, 0.0, 0.0, 0.0], [-150.0, 150.0, 0.0, 0.0, 0.0], [-150.0, 150.0, 0.0, 0.0, 0.0], [-150.0, 150.0, 0.0, 0.0, 0.0], [-150.0, 150.0, 0.0, 0.0, 0.0], [-150.0, 150.0, 0.0, 0.0, 0.0], [0.0, 1.0, 0.0, 0.0, 0.0], [0.0, 1.0, 0.0, 0.0, 0.0], [0.0, 1.0, 0.0, 0.0, 0.0], [0.0, 1.0, 0.0, 0.0, 0.0], [0.0, 0.0001, 0.0, 0.0, 0.0], [0.0, 0.0001, 0.0, 0.0, 0.0], [0.0, 0.0001, 0.0, 0.0, 0.0], [0.0, 0.0001, 0.0, 0.0, 0.0], [0.0, 0.0001, 0.0, 0.0, 0.0], [0.0, 0.0001, 0.0, 0.0, 0.0]]  # Cal Coefficients
  (unwired) string[] ["AI-00/08_Voltage_1", "AI-01/09_Voltage_2", "AI-02/10_Voltage_3", "AI-03/11_Voltage_4", "AI-04/12_Voltage_5", "AI-05/13_Voltage_6", "AI-06_Spare", "AI-14_Spare", "AI-07_Spare", "AI-15_PS_Sense", "AI-16_Pump_Current_1", "AI-17_Pump_Current_2", "AI-18_Pump_Current_3", "AI-19_Pump_Current_4", "AI-20_Pump_Current_5", "AI-21_Pump_Current_6", "AI-16_Pump_Speed_1", "AI-17_Pump_Speed_2", "AI-18_Pump_Speed_3", "AI-19_Pump_Speed_4", "AI-20_Pump_Speed_5", "AI-21_Pump_Speed_6", "AI-22_Controller_Current_1", "AI-23_Controller_Current_2", "AI-24_Controller_Current_3", "AI-25_Controller_Current_4", "AI-26_Controller_Current_5", "AI-27_Controller_Current_6", "AI-28_Temperature_1", "AI-29_Temperature_2", "AI-30_Pump_Pressure_1", "AI-31_Pump_Pressure_2", "AI-32_Pump_Pressure_3", "AI-33_Pump_Pressure_4", "AI-34_Pump_Pressure_5", "AI-35_Pump_Pressure_6", "AI-36_Pump_Flow_1", "AI-37_Pump_Flow_2", "AI-38_Pump_Flow_3", "AI-39_Pump_Flow_4", "AI-40_Pump_Flow_5", "AI-41_Pump_Flow_6", "AI-42_Spare", "AI-43_Spare", "AI-44_Spare", "AI-45_Spare", "AI-46_Spare", "AI-47_Spare", "Pump_Elapsed_Time_1", "Pump_Elapsed_Time_2", "Pump_Elapsed_Time_3", "Pump_Elapsed_Time_4", "Pump_Elapsed_Time_5", "Pump_Elapsed_Time_6"]  # Channel Reference
  (unwired) string[] ["Time", "PS Voltage (V)", "Position 1 Pressure (kPa)", "Position 2 Pressure (kPa)", "Position 3 Pressure (kPa)", "Position 4 Pressure (kPa)", "Position 5 Pressure (kPa)", "Position 6 Pressure (kPa)", "Position 1 Flow (L/H)", "Position 2 Flow (L/H)", "Position 3 Flow (L/H)", "Position 4 Flow (L/H)", "Position 5 Flow (L/H)", "Position 6 Flow (L/H)", "Position 1 Pump Current (A)", "Position 2 Pump Current (A)", "Position 3 Pump Current (A)", "Position 4 Pump Current (A)", "Position 5 Pump Current (A)", "Position 6 Pump Current (A)", "Position 1 Speed (RPM)", "Position 2 Speed (RPM)", "Position 3 Speed (RPM)", "Position 4 Speed (RPM)", "Position 5 Speed (RPM)", "Position 6 Speed (RPM)", "Tank 1 Temp (C )", "Tank 2 Temp (C )", "Position 1 Run Time", "Position 2 Run Time", "Position 3 Run Time", "Position 4 Run Time", "Position 5 Run Time", "Position 6 Run Time"]  # TenHz Header
  w27 = 0  # TenHz Day
  w28 = i32[] [0, 0, 0, 0, 0, 0]  # Cog Limits:
  w29 = FALSE  # Voltage Enable
  w30 = i32[] [0, 0, 0, 0, 0, 0]  # Cog Events
  w31 = i32[] [0, 0, 0, 0, 0, 0]  # CogCounters
  w32 = dbl[] [0.0, 0.0, 0.0, 0.0, 0.0, 0.0, 0.0, 0.0, 0.0, 0.0, 0.0, 0.0, 0.0, 0.0, 0.0, 0.0, 0.0, 0.0, 0.0, 0.0, 0.0, 0.0, 0.0, 0.0, 0.0, 0.0, 0.0, 0.0, 0.0, 0.0, 0.0, 0.0, 0.0, 0.0, 0.0, 0.0, 0.0, 0.0, 0.0, 0.0, 0.0, 0.0, 0.0, 0.0, 0.0, 0.0, 0.0, 0.0, 0.0, 0.0, 0.0, 0.0, 0.0, 0.0]  # Tank Data
  (unwired) string[] ["AI-00_Pump_Current_1", "AI-01_Pump_Current_2", "AI-02_Pump_Current_3", "AI-03_Pump_Current_4", "AI-04_Pump_Current_5", "AI-05_Pump_Current_6", "AI-00_Pump_Speed_1", "AI-01_Pump_Speed_2", "AI-02_Pump_Speed_3", "AI-03_Pump_Speed_4", "AI-04_Pump_Speed_5", "AI-05_Pump_Speed_6", "AI-06_Controller_Current_1", "AI-07_Controller_Current_2", "AI-08_Controller_Current_3", "AI-09_Controller_Current_4", "AI-10_Controller_Current_5", "AI-11_Controller_Current_6", "AI-12_Spare", "AI-13_Temp_1", "AI-14_Temp_2", "AI-15_PS_Sense", "AI-16_Pump_Pressure_1", "AI-17_Pump_Pressure_2", "AI-18_Pump_Pressure_3", "AI-19_Pump_Pressure_4", "AI-20_Pump_Pressure_5", "AI-21_Pump_Pressure_6", "AI-22_Pump_Flow_1", "AI-23_Pump_Flow_2", "AI-24_Pump_Flow_3", "AI-25_Pump_Flow_4", "AI-26_Pump_Flow_5", "AI-27_Pump_Flow_6", "AI-28_Spare", "AI-29_Spare", "AI-30_Spare", "AI-31_Spare", "Pump_Elapsed_Time_1", "Pump_Elapsed_Time_2", "Pump_Elapsed_Time_3", "Pump_Elapsed_Time_4", "Pump_Elapsed_Time_5", "Pump_Elapsed_Time_6"]  # Channel Reference
  w33 = 0.0  # Stop Cmd
  w34 = enum32{"Page 1", "Page 2"}."Page 1"  # Main Tab
  w35 = 0  # AKLH Last Hour
  w36 = FALSE  # TenHz Active?
  w37 = 0.0  # TenHz Timer
  w38 = 0.0  # AKLH Timer
  w39 = path "u:/TenHz"  # TenHz Path
  w40 = path "u:/AKLH"  # AKLH Path
  w41 = fxp<+/-,26,7>[] [0.0, 0.0, 0.0, 0.0, 0.0, 0.0]  # CT Offsets
  w42 = T14[] [enum."Init Files", enum."Init"] items=["Main", "Init Files", "Init", "Save As", "Start Profile", "Check Step Time", "Alarm", "Run Step", "Stop Profile", "Cycle Reset", "Time Reset", "Time Reset All", "Time Set", "Tare CTs", "Save Profile", "Open Profile", "Get Profiles", "Update Screen", "Save Status", "Set Manual CMD", "Reset Restarts", "Reset Total Restarts", "Reset Cogs", "Disable Background", "Enable Background", "Get/Release Control", "Init AKLH", "Save AKLH", "Log Fuel Change", "Update Data Stream", "Init TenHz", "Read TenHz", "Remote Timer Reset", "Record Frequency Change", "Controller Change", "Get Alarms", "Init Alarms", "Save Alarms"]
  w44 = T15 {"Actual Pump Starts"=[0, 0, 0, 0, 0, 0], "Initial Actual Starts"=[0, 0, 0, 0, 0, 0], "Tot Act Starts"=[0, 0, 0, 0, 0, 0], "Tot Init Act Starts"=[0, 0, 0, 0, 0, 0]}  # Actual Starts
  w45 = T4 {"CMD Starts:"=[], "Restarts:"=[], "Total CMD:"=[], "Total Restarts:"=[]}  # Restarts Cluster
  w46 = T3 {"High Limits:"=[30, 30, 30, 30, 30, 30], "Low Limits:"=[30, 30, 30, 30, 30, 30]}  # Restarts Limits
  w47 = FALSE  # New Step
  w48 = 0  # Stagger Counter
  w49 = FALSE  # Login
  w50 = T2 {"Pump 1"=FALSE, "Pump 2"=FALSE, "Pump 3"=FALSE, "Pump 4"=FALSE, "Pump 5"=FALSE, "Pump 6"=FALSE}  # Pumps Present
  w51 = FALSE  # Alarm
  w52 = dbl[] [0.0, 0.0, 0.0, 0.0, 0.0, 0.0]  # Intitial Times
  w53 = dbl[] [0.0, 0.0, 0.0, 0.0, 0.0, 0.0]  # Elapsed Times
  w54 = FALSE  # Update Profile
  w55 = dbl[] [0.0, 0.0, 0.0, 0.0, 0.0, 0.0]  # Last CMDs
  w56 = bool[] [FALSE, FALSE, FALSE, FALSE, FALSE, FALSE]  # pb.Sets
  w57 = bool[] [FALSE, FALSE, FALSE, FALSE, FALSE, FALSE]  # pb.Resets
  w58 = FALSE  # pb.Run Profile
  w59 = FALSE  # Client?
  w60 = dbl[] [0.0, 0.0, 0.0, 0.0, 0.0, 0.0]  # Manual CMDs
  w61 = 0.0  # Last Profile Time
  w62 = FALSE  # Update Screen
  w63 = 0.0  # Last Update
  w64 = 0  # # of Steps
  w65 = 0.0  # Step Time
  w66 = 0.0  # Step Start Time
  w67 = FALSE  # Run Profile
  w69 = 0  # Current Step
  w68 = 0.0  # Step Time Left
  w70 = string[] []  # Profiles
  w71 = T16 {"Location"="", "Profiles Path"=path "", "Current Profile"="", "CA Number"="", "Cycles Completed"=0, "PWM Freq (Hz)"=0.0, "Controller Type:"=enum."Kuhnke", "Inform"="", "Pumps Present"=0, "Stagger Time (ms)"=0, "Tank 1 Fuel"="", "Tank 2 Fuel"="", "Serial Numbers"={"Position 1 SN"="", "Position 2 SN"="", "Poaition 3 SN"="", "Position 4 SN"="", "Position 5 SN"="", "Position 6 SN"=""}, "Record TenHz"=FALSE, "VoltCtrlRef"="", "TenHzFrequency"=0}  # App Config
  w72 = string[][] []  # Profile
  w73 = errorcluster {"status"=FALSE, "code"=0, "source"=""}  # Error
  # "Timer Data 180"
  # "There is no longer a reason to have CT Offsets but"
  # "***** NEW ******"
  # "|\n|\n|\n|\n|\n|\n|\n|\n|\n|\n|\n|\n|\n|"
  # "******************************************     O L D      ***************************************"
  # "PWM Period (Ticks) = 40,000,000 / PWM Period (Hz)\nPWM Period (Ticks) = 40,000,000 * PWM Period (sec)\nPWM Duty Cycle (Ticks) = PWM Period (Ticks) * PWM Duty Cycle (%) / 100\nPWM Duty Cycle (Ticks) = 40,000,000 * PWM Duty Cycle (sec)"
  # "Need a way to make sure I dont overflow the RIO\n\nNeed to create a way to split up a section of data to make data collected after middnight go to the next day\n\nneed to figure out how to deal with the SD card being removed and replaced"
  # "I think I can remove Voltage\nEnable from shift register"
  # "Traces Timer\nTraces Path\nTenHz Data\nTenHzDataIndex\nTenHzLastHourpb.Save As\npb.Stop Profile\npb.Cycle Reset\npb.Zero CMDs\npb.Reset Restarts\npb.Time Reset All\npb.Rst Tot Restarts\npb.FuelChange\npb.Reset Cogs\npb.ViewProfile\npb.ViewData\nAll removed from shift register"
  # "Need a way to verify that the AKLH files do not pile up and fill the RIO space"
  # "AI Data 1000"
  # "FPGA FIFO AI Data originally had 45 channels and asked for 10000 addresses reserved that would 222 possible full sets of data\nI would think 3 would be all that would be required 1 to find indexer, 1 to read, and 1 more in case RT is looping slightly faster than FPGA"
  # "I dont think I want to shut off voltage when the lower stop button is pressed"
  # "I believe PWM? in Controller Selection is useless once I have all the CAN selections initiated in the CAN loop"
  # "Remove PWM Freq (Hz) from app config and reference Frequency in Controller Selection"
  # "Do I have to put CA#, Requester(s), Start date... inside AKLH data file\nDo I have to include the profile on a second sheet\n\nwhen the controller type is non-controller brushed need to multiply controll current by zero... maybe\n\nLong-term would want to have a shutoff based on Cycles completed or all active pumps on time"
  # "Should change so that the PS, pres, and solenoid enable are\nnot stored in 2 places (app config and profile enables)"
  n1 = Bundle("Error"=w73, "Profile"=w72, "App Config"=w71, "Profiles"=w70, "Current Step"=w69, "Step Time Left"=w68, "Run Profile"=w67, "Step Start Time"=w66, "Step Time"=w65, "# of Steps"=w64, "Last Update"=w63, "Update Screen"=w62, "Last Profile Time"=w61, "Manual CMDs"=w60, "Client?"=w59, "pb.Run Profile"=w58, "pb.Resets"=w57, "pb.Sets"=w56, "Last CMDs"=w55, "Update Profile"=w54, "Elapsed Times"=w53, "Intitial Times"=w52, "Alarm"=w51, "CT Offsets"=w41, "Pumps Present"=w50, "Login"=w49, "Stagger Counter"=w48, "New Step"=w47, "Restarts Limits"=w46, "Restarts Cluster"=w45, "Actual Starts"=w44, "AKLH Path"=w40, "TenHz Path"=w39, "AKLH Timer"=w38, "TenHz Timer"=w37, "TenHz Active?"=w36, "AKLH Last Hour"=w35, "Main Tab"=w34, "Stop Cmd"=w33, "Tank Data"=w32, "CogCounters"=w31, "Cog Events"=w30, "Voltage Enable"=w29, "Cog Limits:"=w28, "TenHz Day"=w27, "Controller"=w15, "PS CMD"=w21, "Press CMD"=w20, "Temp CMD"=w19, "Power Relay"=w18, "Ignition Relay"=w17, "Controller List"=w14, "Alarm Config"=w13, "Alarm Config Path"=w12, "Trip Counters"=w11, "Previous Times"=w10, "Alarm Message"=w9, "Restart Alarm"=w8, "Prev ON Times"=w7) -> (w43:T17)  [unwired: 1 in]
  n2 = flat-sequence {
    tunnel: [w74] -> w4
    tunnel: w22 -> [w74]
    frame #0 {
      n3 = Wait (ms)(milliseconds to wait=u32 5000) -> ()  [unwired: 1 out]
    }
  }
  n4 = xnode "Open FPGA VI Reference"("resource name"=tag "RIO0") -> ("FPGA VI Reference Out"=w22:T18, "error out"=w26:errorcluster)  [unwired: 1 in]
  n5 = call "CAN Communication.vi"("CAN Mode"=CAN_Mode."Init") -> ("Error OUT"=w24:errorcluster)  [unwired: 10 in]
  n6 = Generate Occurrence() -> (w16:refnum<k4>)
  n7 = call "RPi HMI Com.vi"("RPi HMI Mode"=RPi_HMI_Mode."Init") -> ("HMI Cluster"=w5:T19)  [unwired: 18 in]
  n8 = disable-structure shown="Disabled" {
    disable-tunnel: w22 -> [w77 _]
    disable-tunnel: w16 -> [w76 _]
    frame Disabled {
      n9 = flat-sequence {
        tunnel: w76 -> [w83]
        tunnel: [w82] -> w81
        tunnel: w77 -> [w82]
        tunnel: [w87] -> w80
        tunnel: w81 -> [w87]
        tunnel: w80 -> [w93]
        tunnel: [w92] -> w79
        tunnel: [w95] -> w78
        tunnel: w79 -> [w95]
        tunnel: w78 -> [w98]
        frame #0 {
          n10 = Wait on Occurrence(2:w83) -> ()  [unwired: 2 in, 1 out]
        }
        frame #1 {
          n11 = call "AI RT FIFO.vi"("Mode"=RT_FIFO_Mode."Create", "Buffer Size"=1000, "# of elements"=54) -> ()  [unwired: 10 in, 3 out]
        }
        frame #2 {
          n12 = control-ref of="Stop"() -> (w90:refnum<vi>)
          n13 = property class="Bool (strict)"(reference=w90, "Value"=FALSE) -> (reference out=w89:refnum<vi>)  [unwired: 1 in, 1 out]
          n14 = call "Loop (DMA).vi"("Stop"=w89, "Sample Rate"=u32 10, "FPGA Ref"=w93) -> ("FPGA Ref OUT"=w92:T18)  [unwired: 7 in, 1 out]
          n15 = call "Loop (Data Stream).vi"("Stop"=w89) -> ()  [unwired: 10 in, 1 out]
        }
        frame #3 {
          n16 = call "AI RT FIFO.vi"("Mode"=RT_FIFO_Mode."Delete") -> ()  [unwired: 12 in, 3 out]
        }
        frame #4 {
          n17 = xnode "Invoke Method"("FPGA VI Reference In"=w98) -> ("FPGA VI Reference Out"=w96:T18, "error out"=w97:errorcluster)  [unwired: 1 in]
          n18 = xnode "Close FPGA VI Reference"("FPGA VI Reference In"=w96, "error in"=w97) -> ()  [unwired: 1 out]
        }
      }
    }
    frame Enabled {
    }
  }
  n19 = while {
    tunnel: w24 -> [w102]
    i -> [w99]
    stop <- FALSE stop-if-true
    n20 = local read "Controller Type:"() -> (w100:T5)
    n21 = local read "CAN CMD"() -> (w101:dbl)
    n22 = case shown="\"Hella CAN\"" w100 {
      tunnel: w102 -> [_ w107 w110 w115 w119 w123]
      tunnel: w101 -> [_ w106 w109 w117 w120 w121]
      tunnel: w99 -> [_ _ _ w114 _ _]
      frame "Kuhnke", Default {
        n23 = Wait (ms)(milliseconds to wait=u32 500) -> ()  [unwired: 1 out]
      }
      frame "Conti" {
        n24 = To Unsigned Word Integer(number=w106) -> (unsigned 16bit integer=w105:u16)
        n25 = call "Conti CAN.vi"("Error IN"=w107, "CMD"=w105) -> ()  [unwired: 9 in, 1 out]
      }
      frame "Hella CAN" {
        n26 = To Unsigned Byte Integer(number=w109) -> (unsigned 8bit integer=w108:u8)
        n27 = call "Hella CAN.vi"("Error IN"=w110, "CMD"=w108) -> ()  [unwired: 9 in, 1 out]
      }
      frame "Helbako" {
        n28 = Quotient & Remainder(x=w114, y=10) -> (x-y*floor(x/y)=w112:i32)  [unwired: 1 out]
        n29 = To Unsigned Word Integer(number=w117) -> (unsigned 16bit integer=w116:u16)
        n30 = Equal To 0?(x=w112) -> (x = 0?=w111:bool)
        n31 = call "Helbako CAN.vi"("Split-timer"=w111, "Error IN"=w115, "CMD"=w116) -> ()  [unwired: 8 in, 1 out]
      }
      frame "PSA" {
        n32 = To Unsigned Word Integer(number=w120) -> (unsigned 16bit integer=w118:u16)
        n33 = call "Hella CAN Gas.vi"("Pressure Command (kPa)"=w118, "Error In"=w119) -> ()  [unwired: 12 in, 2 out]
      }
      frame "Hella DC Gas" {
        n34 = To Unsigned Word Integer(number=w121) -> (unsigned 16bit integer=w122:u16)
        n35 = call "Hella CAN Diesel.vi"("Command (kPa)"=w122, "Error In"=w123) -> ()  [unwired: 13 in, 1 out]
      }
    }
  }
  n36 = while {
    tunnel: w5 -> [_]
    tunnel: w16 -> [_]
    stop <- FALSE stop-if-true
    n37 = flat-sequence {
      frame #0 {
        n38 = call "RPi HMI Com.vi"("RPi HMI Mode"=RPi_HMI_Mode."Read from RPi") -> ("HMI Cluster"=w133:T19)  [unwired: 18 in]
        n39 = Unbundle By Name(w133) -> ("HMI Command"=w132:bool, "Power Relays"=w131:T2, "Pump CMDs"=w130:dbl[], "Tank CMDs.PS CMD"=w129:dbl, "Tank CMDs.Press CMD"=w128:dbl, "HMI Tog Buttons.Start Test"=w127:bool, "HMI Mom Buttons"=w126:T1)  [unwired: 1 out]
        n40 = case shown="True" w132 {
          tunnel: w131 -> [_ w140]
          tunnel: w130 -> [_ w139]
          tunnel: w129 -> [_ w138]
          tunnel: w128 -> [_ w137]
          tunnel: w127 -> [_ w136]
          tunnel: w126 -> [_ w135]
          frame False {
          }
          frame True {
            n41 = flat-sequence {
              tunnel: w140 -> [w146]
              tunnel: w139 -> [w145]
              tunnel: w138 -> [w144]
              tunnel: w137 -> [w143]
              tunnel: w136 -> [w142]
              tunnel: w135 -> [w141]
              frame #0 {
                n42 = local write "Power Relay"(w146) -> ()
                n43 = local write "Manual\nCMD"(w145) -> ()
                n44 = local write "Power Supply Cmd (V):"(w144) -> ()
                n45 = local write "PressureCMD"(w143) -> ()
                n46 = local write "pb.Run Profile"(w142) -> ()
                "HMI Mom Buttons" <- w141
              }
              frame #1 {
                n47 = Wait (ms)(milliseconds to wait=u32 20) -> ()  [unwired: 1 out]
              }
            }
          }
        }
      }
      frame #1 {
        n48 = call "RPi HMI Com.vi"("RPi HMI Mode"=RPi_HMI_Mode."Write to RPi") -> ()  [unwired: 18 in, 1 out]
      }
    }
    n49 = Wait (ms)(milliseconds to wait=u32 80) -> ()  [unwired: 1 out]
  }
  n50 = while {
    shift-right: [w158] -> _
    shift-left: w42 -> [w156]
    shift-right: [w159] -> _
    shift-left: w43 -> [w160]
    tunnel: w22 -> [w157]
    tunnel: w16 -> [w149]
    tunnel: w26 -> [_]
    stop <- FALSE stop-if-true
    n51 = Delete From Array(array=w156, length=1, index=0 ("length")) -> (deleted portion=w152:T14[], array with subset deleted=w155:T14[])
    n52 = Wait (ms)(milliseconds to wait=u32 20) -> ()  [unwired: 1 out]
    n53 = Index Array(array=w152) -> (element=w151:T14)  [unwired: 1 in]
    n54 = case shown="\"Update Screen\"" w151 {
      selector: w151 -> [_ _ _ _ _ _ _ _ _ _ _ _ _ _ _ _ _ _ w1193 _ _ _ _ _ _ _ _ _ _ _ _ _]
      tunnel: [w193 w572 w707 w798 w818 w838 w846 w862 w877 w897 w920 w968 w977 w1090 w1119 w1140 w1183 w1192 w1204 w1273 w1320 w1341 w1397 w1463 w1482 w1521 w1626 w1635 w1650 w1735 w1770 w1783] -> w159
      tunnel: w160 -> [w190 w573 w705 w799 w819 w838 w847 w863 w878 w898 w921 w969 w1047 w1079 w1120 w1140 w1183 w1192 w1194 w1274 w1319 w1338 w1397 w1463 w1483 w1522 w1627 w1635 w1651 w1720 w1770 w1784]
      tunnel: [w179 w584 w711 w794 w822 w839 w840 w851 w876 w891 w918 w958 w1045 w1084 w1121 w1162 w1182 w1188 w1195 w1289 w1309 w1339 w1401 w1461 w1485 w1514 w1614 w1634 w1649 w1734 w1769 w1788] -> w158
      tunnel: w157 -> [_ _ w709 _ _ _ _ _ _ _ _ w947 w980 w1088 _ _ _ w1191 w1198 _ w1312 w1340 w1391 _ _ _ _ _ _ w1698 _ w1785]
      tunnel: w155 -> [_ w584 _ w793 w822 w839 w841 w852 _ _ _ w958 w1044 w1086 _ w1162 w1182 w1189 _ _ _ w1339 w1401 w1461 w1485 w1515 w1615 w1634 w1649 w1734 w1769 w1788]
      tunnel: w149 -> [_ _ w689 _ _ _ _ _ _ _ _ _ _ _ _ _ _ _ _ _ _ _ _ _ _ _ _ _ _ _ _ _]
      frame "Main", Default {
        # "Any Latch when released boolean buttons do not need to be stored\nin the shift register they had been stored and looked at if they were\ngreater than the past value stored in the shift register"
        n55 = Unbundle By Name(w190) -> ("Run Profile"=w188:bool, "Last Update"=w192:dbl, "TenHz Timer"=w176:dbl, "AKLH Timer"=w175:dbl, "App Config.Record TenHz"=w167:bool, "TenHz Day"=w166:i32)
        n56 = for {
          N: 41 -> [_]
          shift-right: [w208] -> w191
          shift-left: w190 -> [w207]
          tunnel: [w206] -> w187
          tunnel: [w205] -> w189
          i -> [w209]
          stop <- w205 stop-if-true
          n57 = case shown="7" w209 {
            tunnel: w207 -> [w216 w223 w225 w233 w236 w238 w246 w253 w261 w268 w275 w283 w286 w294 w301 w308 w315 w316 w322 w323 w333 w340 w347 w349 w358 w359 w363 w366 w373 w380 w387 w395 w403 w405 w409 w501 w507 w515 w519 w528 w538]
            tunnel: [w215 w222 w225 w232 w236 w238 w245 w252 w260 w267 w274 w282 w286 w293 w300 w307 w314 w316 w322 w323 w332 w339 w346 w349 w357 w359 w363 w366 w372 w379 w386 w394 w402 w405 w410 w500 w506 w514 w518 w528 w537] -> w208
            tunnel: [w212 "pb.E Stop" "pb.Save As" w231 "pb.Stop Profile" "pb.Cycle Reset" w244 w251 w257 w264 w271 w276 "pb.Zero CMDs" w290 w297 w304 w311 "pb.Reset Restarts" w320 "pb.Time Reset All" w331 w338 w345 "pb.Rst Tot Restarts" w354 "pb.FuelChange" FALSE ("Restarts Alarm") FALSE ("Restarts Alarm") w368 w377 w382 w392 w398 "pb.Reset Cogs" w408 w498 w503 w511 w521 w524 w540] -> w205
            tunnel: w207 -> [w214 w221 _ w230 _ _ w243 w250 w259 w266 w273 w281 _ w292 w299 w306 w313 _ w321 _ w330 w337 w344 _ w356 _ _ _ w371 w378 w385 w396 w404 _ w412 w499 w508 w513 w520 _ w539]
            tunnel: [w211 w224 w226 w228 w237 w240 w241 w248 w256 w262 w269 w279 w287 w288 w296 w303 w310 w318 w319 w325 w329 w336 w343 w351 w353 w361 w362 w365 w374 w381 w388 w389 w397 w407 w414 w495 w502 w512 w522 w529 w541] -> w206
            frame 0, Default {
              w211 = T14[] [enum."Set Manual CMD"] items=["Main", "Init Files", "Init", "Save As", "Start Profile", "Check Step Time", "Alarm", "Run Step", "Stop Profile", "Cycle Reset", "Time Reset", "Time Reset All", "Time Set", "Tare CTs", "Save Profile", "Open Profile", "Get Profiles", "Update Screen", "Save Status", "Set Manual CMD", "Reset Restarts", "Reset Total Restarts", "Reset Cogs", "Disable Background", "Enable Background", "Get/Release Control", "Init AKLH", "Save AKLH", "Log Fuel Change", "Update Data Stream", "Init TenHz", "Read TenHz", "Remote Timer Reset", "Record Frequency Change", "Controller Change", "Get Alarms", "Init Alarms", "Save Alarms"]
              n58 = Unbundle By Name(w214) -> ("PS CMD"=w213:dbl)
              n59 = Not Equal?(x=w213, y="Power Supply Cmd (V):") -> (x != y?=w212:bool)
              n60 = Bundle By Name(cluster=w216, "PS CMD"="Power Supply Cmd (V):") -> (w215:T17)
            }
            frame 1 {
              w224 = T14[] [enum."Set Manual CMD"] items=["Main", "Init Files", "Init", "Save As", "Start Profile", "Check Step Time", "Alarm", "Run Step", "Stop Profile", "Cycle Reset", "Time Reset", "Time Reset All", "Time Set", "Tare CTs", "Save Profile", "Open Profile", "Get Profiles", "Update Screen", "Save Status", "Set Manual CMD", "Reset Restarts", "Reset Total Restarts", "Reset Cogs", "Disable Background", "Enable Background", "Get/Release Control", "Init AKLH", "Save AKLH", "Log Fuel Change", "Update Data Stream", "Init TenHz", "Read TenHz", "Remote Timer Reset", "Record Frequency Change", "Controller Change", "Get Alarms", "Init Alarms", "Save Alarms"]
              n61 = Unbundle By Name(w221) -> ("PS CMD"=w220:dbl)
              n62 = Select(t=0.0, s="pb.E Stop", f=w220) -> (s? t:f=w218:dbl)
              n63 = local write "Power Supply Cmd (V):"(w218) -> ()
              n64 = Bundle By Name(cluster=w223, "PS CMD"=w218, "Voltage Enable"="pb.E Stop") -> (w222:T17)
            }
            frame 2 {
              w226 = T14[] [enum."Disable Background", enum."Save As"] items=["Main", "Init Files", "Init", "Save As", "Start Profile", "Check Step Time", "Alarm", "Run Step", "Stop Profile", "Cycle Reset", "Time Reset", "Time Reset All", "Time Set", "Tare CTs", "Save Profile", "Open Profile", "Get Profiles", "Update Screen", "Save Status", "Set Manual CMD", "Reset Restarts", "Reset Total Restarts", "Reset Cogs", "Disable Background", "Enable Background", "Get/Release Control", "Init AKLH", "Save AKLH", "Log Fuel Change", "Update Data Stream", "Init TenHz", "Read TenHz", "Remote Timer Reset", "Record Frequency Change", "Controller Change", "Get Alarms", "Init Alarms", "Save Alarms"]
            }
            frame 3 {
              w228 = T14[] [enum."Start Profile"] items=["Main", "Init Files", "Init", "Save As", "Start Profile", "Check Step Time", "Alarm", "Run Step", "Stop Profile", "Cycle Reset", "Time Reset", "Time Reset All", "Time Set", "Tare CTs", "Save Profile", "Open Profile", "Get Profiles", "Update Screen", "Save Status", "Set Manual CMD", "Reset Restarts", "Reset Total Restarts", "Reset Cogs", "Disable Background", "Enable Background", "Get/Release Control", "Init AKLH", "Save AKLH", "Log Fuel Change", "Update Data Stream", "Init TenHz", "Read TenHz", "Remote Timer Reset", "Record Frequency Change", "Controller Change", "Get Alarms", "Init Alarms", "Save Alarms"]
              n65 = Unbundle By Name(w230) -> ("pb.Run Profile"=w234:bool)
              n66 = Greater?(x="pb.Run Profile", y=w234) -> (0:w231:bool)
              n67 = Bundle By Name(cluster=w233, "pb.Run Profile"="pb.Run Profile") -> (w232:T17)
            }
            frame 4 {
              w237 = T14[] [enum."Stop Profile"] items=["Main", "Init Files", "Init", "Save As", "Start Profile", "Check Step Time", "Alarm", "Run Step", "Stop Profile", "Cycle Reset", "Time Reset", "Time Reset All", "Time Set", "Tare CTs", "Save Profile", "Open Profile", "Get Profiles", "Update Screen", "Save Status", "Set Manual CMD", "Reset Restarts", "Reset Total Restarts", "Reset Cogs", "Disable Background", "Enable Background", "Get/Release Control", "Init AKLH", "Save AKLH", "Log Fuel Change", "Update Data Stream", "Init TenHz", "Read TenHz", "Remote Timer Reset", "Record Frequency Change", "Controller Change", "Get Alarms", "Init Alarms", "Save Alarms"]
            }
            frame 5 {
              w240 = T14[] [enum."Disable Background", enum."Cycle Reset"] items=["Main", "Init Files", "Init", "Save As", "Start Profile", "Check Step Time", "Alarm", "Run Step", "Stop Profile", "Cycle Reset", "Time Reset", "Time Reset All", "Time Set", "Tare CTs", "Save Profile", "Open Profile", "Get Profiles", "Update Screen", "Save Status", "Set Manual CMD", "Reset Restarts", "Reset Total Restarts", "Reset Cogs", "Disable Background", "Enable Background", "Get/Release Control", "Init AKLH", "Save AKLH", "Log Fuel Change", "Update Data Stream", "Init TenHz", "Read TenHz", "Remote Timer Reset", "Record Frequency Change", "Controller Change", "Get Alarms", "Init Alarms", "Save Alarms"]
            }
            frame 6 {
              w241 = T14[] [enum."Disable Background", enum."Time Reset"] items=["Main", "Init Files", "Init", "Save As", "Start Profile", "Check Step Time", "Alarm", "Run Step", "Stop Profile", "Cycle Reset", "Time Reset", "Time Reset All", "Time Set", "Tare CTs", "Save Profile", "Open Profile", "Get Profiles", "Update Screen", "Save Status", "Set Manual CMD", "Reset Restarts", "Reset Total Restarts", "Reset Cogs", "Disable Background", "Enable Background", "Get/Release Control", "Init AKLH", "Save AKLH", "Log Fuel Change", "Update Data Stream", "Init TenHz", "Read TenHz", "Remote Timer Reset", "Record Frequency Change", "Controller Change", "Get Alarms", "Init Alarms", "Save Alarms"]
              n68 = Unbundle By Name(w243) -> ("pb.Resets"=w247:bool[])
              n69 = Greater?(x="pb.Resets", y=w247) -> (0:w244:bool)
              n70 = Bundle By Name(cluster=w246, "pb.Resets"="pb.Resets") -> (w245:T17)
            }
            frame 7 {
              w248 = T14[] [enum."Disable Background", enum."Time Set"] items=["Main", "Init Files", "Init", "Save As", "Start Profile", "Check Step Time", "Alarm", "Run Step", "Stop Profile", "Cycle Reset", "Time Reset", "Time Reset All", "Time Set", "Tare CTs", "Save Profile", "Open Profile", "Get Profiles", "Update Screen", "Save Status", "Set Manual CMD", "Reset Restarts", "Reset Total Restarts", "Reset Cogs", "Disable Background", "Enable Background", "Get/Release Control", "Init AKLH", "Save AKLH", "Log Fuel Change", "Update Data Stream", "Init TenHz", "Read TenHz", "Remote Timer Reset", "Record Frequency Change", "Controller Change", "Get Alarms", "Init Alarms", "Save Alarms"]
              n71 = Unbundle By Name(w250) -> ("pb.Sets"=w254:bool[])
              n72 = Greater?(x="pb.Sets", y=w254) -> (0:w251:bool)
              n73 = Bundle By Name(cluster=w253, "pb.Sets"="pb.Sets") -> (w252:T17)
            }
            frame 8 {
              w256 = T14[] [enum."Save Profile"] items=["Main", "Init Files", "Init", "Save As", "Start Profile", "Check Step Time", "Alarm", "Run Step", "Stop Profile", "Cycle Reset", "Time Reset", "Time Reset All", "Time Set", "Tare CTs", "Save Profile", "Open Profile", "Get Profiles", "Update Screen", "Save Status", "Set Manual CMD", "Reset Restarts", "Reset Total Restarts", "Reset Cogs", "Disable Background", "Enable Background", "Get/Release Control", "Init AKLH", "Save AKLH", "Log Fuel Change", "Update Data Stream", "Init TenHz", "Read TenHz", "Remote Timer Reset", "Record Frequency Change", "Controller Change", "Get Alarms", "Init Alarms", "Save Alarms"]
              n74 = Unbundle By Name(w259) -> ("Profile"=w258:string[][])
              n75 = Not Equal?(x=w258, y="Profile:") -> (x != y?=w257:bool)
              n76 = Bundle By Name(cluster=w261, "Profile"="Profile:") -> (w260:T17)
            }
            frame 9 {
              w262 = T14[] [enum."Open Profile"] items=["Main", "Init Files", "Init", "Save As", "Start Profile", "Check Step Time", "Alarm", "Run Step", "Stop Profile", "Cycle Reset", "Time Reset", "Time Reset All", "Time Set", "Tare CTs", "Save Profile", "Open Profile", "Get Profiles", "Update Screen", "Save Status", "Set Manual CMD", "Reset Restarts", "Reset Total Restarts", "Reset Cogs", "Disable Background", "Enable Background", "Get/Release Control", "Init AKLH", "Save AKLH", "Log Fuel Change", "Update Data Stream", "Init TenHz", "Read TenHz", "Remote Timer Reset", "Record Frequency Change", "Controller Change", "Get Alarms", "Init Alarms", "Save Alarms"]
              n77 = Unbundle By Name(w266) -> ("App Config.Current Profile"=w265:string)
              n78 = Not Equal?(x=w265, y="Profile Name:") -> (x != y?=w264:bool)
              n79 = Bundle By Name(cluster=w268, "App Config.Current Profile"="Profile Name:") -> (w267:T17)
            }
            frame 10 {
              w269 = T14[] [enum."Set Manual CMD"] items=["Main", "Init Files", "Init", "Save As", "Start Profile", "Check Step Time", "Alarm", "Run Step", "Stop Profile", "Cycle Reset", "Time Reset", "Time Reset All", "Time Set", "Tare CTs", "Save Profile", "Open Profile", "Get Profiles", "Update Screen", "Save Status", "Set Manual CMD", "Reset Restarts", "Reset Total Restarts", "Reset Cogs", "Disable Background", "Enable Background", "Get/Release Control", "Init AKLH", "Save AKLH", "Log Fuel Change", "Update Data Stream", "Init TenHz", "Read TenHz", "Remote Timer Reset", "Record Frequency Change", "Controller Change", "Get Alarms", "Init Alarms", "Save Alarms"]
              n80 = Unbundle By Name(w273) -> ("Manual CMDs"=w272:dbl[])
              n81 = Not Equal?(x=w272, y="Manual\nCMD") -> (x != y?=w271:bool)
              n82 = Bundle By Name(cluster=w275, "Manual CMDs"="Manual\nCMD") -> (w274:T17)
            }
            frame 11 {
              w279 = T14[] [enum."Get/Release Control"] items=["Main", "Init Files", "Init", "Save As", "Start Profile", "Check Step Time", "Alarm", "Run Step", "Stop Profile", "Cycle Reset", "Time Reset", "Time Reset All", "Time Set", "Tare CTs", "Save Profile", "Open Profile", "Get Profiles", "Update Screen", "Save Status", "Set Manual CMD", "Reset Restarts", "Reset Total Restarts", "Reset Cogs", "Disable Background", "Enable Background", "Get/Release Control", "Init AKLH", "Save AKLH", "Log Fuel Change", "Update Data Stream", "Init TenHz", "Read TenHz", "Remote Timer Reset", "Record Frequency Change", "Controller Change", "Get Alarms", "Init Alarms", "Save Alarms"]
              n83 = Unbundle By Name(w281) -> ("Client?"=w277:bool, "Profiles"=w280:string[])
              n84 = local read "Client?"() -> (w278:bool)
              n85 = Greater?(x=w278, y=w277) -> (0:w276:bool)
              n86 = case shown="True" w276 {
                tunnel: w280 -> [_ w284]
                frame False {
                }
                frame True {
                  n87 = property on="Profile Name:" class="CmbBox"("Strings[]"=w284) -> ()  [unwired: 2 in, 2 out]
                }
              }
              n88 = Bundle By Name(cluster=w283, "Client?"=w278) -> (w282:T17)
            }
            frame 12 {
              w287 = T14[] [enum."Stop Profile"] items=["Main", "Init Files", "Init", "Save As", "Start Profile", "Check Step Time", "Alarm", "Run Step", "Stop Profile", "Cycle Reset", "Time Reset", "Time Reset All", "Time Set", "Tare CTs", "Save Profile", "Open Profile", "Get Profiles", "Update Screen", "Save Status", "Set Manual CMD", "Reset Restarts", "Reset Total Restarts", "Reset Cogs", "Disable Background", "Enable Background", "Get/Release Control", "Init AKLH", "Save AKLH", "Log Fuel Change", "Update Data Stream", "Init TenHz", "Read TenHz", "Remote Timer Reset", "Record Frequency Change", "Controller Change", "Get Alarms", "Init Alarms", "Save Alarms"]
            }
            frame 13 {
              w288 = T14[] [enum."Save Status"] items=["Main", "Init Files", "Init", "Save As", "Start Profile", "Check Step Time", "Alarm", "Run Step", "Stop Profile", "Cycle Reset", "Time Reset", "Time Reset All", "Time Set", "Tare CTs", "Save Profile", "Open Profile", "Get Profiles", "Update Screen", "Save Status", "Set Manual CMD", "Reset Restarts", "Reset Total Restarts", "Reset Cogs", "Disable Background", "Enable Background", "Get/Release Control", "Init AKLH", "Save AKLH", "Log Fuel Change", "Update Data Stream", "Init TenHz", "Read TenHz", "Remote Timer Reset", "Record Frequency Change", "Controller Change", "Get Alarms", "Init Alarms", "Save Alarms"]
              n89 = Unbundle By Name(w292) -> ("App Config.CA Number"=w291:string)
              n90 = Not Equal?(x=w291, y="CA Number:") -> (x != y?=w290:bool)
              n91 = Bundle By Name(cluster=w294, "App Config.CA Number"="CA Number:") -> (w293:T17)
            }
            frame 14 {
              w296 = T14[] [enum."Save Status", enum."Controller Change"] items=["Main", "Init Files", "Init", "Save As", "Start Profile", "Check Step Time", "Alarm", "Run Step", "Stop Profile", "Cycle Reset", "Time Reset", "Time Reset All", "Time Set", "Tare CTs", "Save Profile", "Open Profile", "Get Profiles", "Update Screen", "Save Status", "Set Manual CMD", "Reset Restarts", "Reset Total Restarts", "Reset Cogs", "Disable Background", "Enable Background", "Get/Release Control", "Init AKLH", "Save AKLH", "Log Fuel Change", "Update Data Stream", "Init TenHz", "Read TenHz", "Remote Timer Reset", "Record Frequency Change", "Controller Change", "Get Alarms", "Init Alarms", "Save Alarms"]
              n92 = Unbundle By Name(w299) -> ("App Config.Controller Type:"=w298:T5)
              n93 = Not Equal?(x=w298, y="Controller Type:") -> (x != y?=w297:bool)
              n94 = Bundle By Name(cluster=w301, "App Config.Controller Type:"="Controller Type:") -> (w300:T17)
            }
            frame 15 {
              w303 = T14[] [enum."Save Status"] items=["Main", "Init Files", "Init", "Save As", "Start Profile", "Check Step Time", "Alarm", "Run Step", "Stop Profile", "Cycle Reset", "Time Reset", "Time Reset All", "Time Set", "Tare CTs", "Save Profile", "Open Profile", "Get Profiles", "Update Screen", "Save Status", "Set Manual CMD", "Reset Restarts", "Reset Total Restarts", "Reset Cogs", "Disable Background", "Enable Background", "Get/Release Control", "Init AKLH", "Save AKLH", "Log Fuel Change", "Update Data Stream", "Init TenHz", "Read TenHz", "Remote Timer Reset", "Record Frequency Change", "Controller Change", "Get Alarms", "Init Alarms", "Save Alarms"]
              n95 = Unbundle By Name(w306) -> ("Restarts Limits"=w305:T3)
              n96 = Not Equal?(x=w305, y="Restarts Limits") -> (x != y?=w304:bool)
              n97 = Bundle By Name(cluster=w308, "Restarts Limits"="Restarts Limits") -> (w307:T17)
            }
            frame 16 {
              w310 = T14[] [enum."Save Status"] items=["Main", "Init Files", "Init", "Save As", "Start Profile", "Check Step Time", "Alarm", "Run Step", "Stop Profile", "Cycle Reset", "Time Reset", "Time Reset All", "Time Set", "Tare CTs", "Save Profile", "Open Profile", "Get Profiles", "Update Screen", "Save Status", "Set Manual CMD", "Reset Restarts", "Reset Total Restarts", "Reset Cogs", "Disable Background", "Enable Background", "Get/Release Control", "Init AKLH", "Save AKLH", "Log Fuel Change", "Update Data Stream", "Init TenHz", "Read TenHz", "Remote Timer Reset", "Record Frequency Change", "Controller Change", "Get Alarms", "Init Alarms", "Save Alarms"]
              n98 = Unbundle By Name(w313) -> ("App Config.Inform"=w312:string)
              n99 = Not Equal?(x=w312, y="Inform:") -> (x != y?=w311:bool)
              n100 = Bundle By Name(cluster=w315, "App Config.Inform"="Inform:") -> (w314:T17)
            }
            frame 17 {
              w318 = T14[] [enum."Disable Background", enum."Reset Restarts"] items=["Main", "Init Files", "Init", "Save As", "Start Profile", "Check Step Time", "Alarm", "Run Step", "Stop Profile", "Cycle Reset", "Time Reset", "Time Reset All", "Time Set", "Tare CTs", "Save Profile", "Open Profile", "Get Profiles", "Update Screen", "Save Status", "Set Manual CMD", "Reset Restarts", "Reset Total Restarts", "Reset Cogs", "Disable Background", "Enable Background", "Get/Release Control", "Init AKLH", "Save AKLH", "Log Fuel Change", "Update Data Stream", "Init TenHz", "Read TenHz", "Remote Timer Reset", "Record Frequency Change", "Controller Change", "Get Alarms", "Init Alarms", "Save Alarms"]
            }
            frame 18 {
              w319 = T14[] [enum."Stop Profile", enum."Disable Background", enum."Alarm"] items=["Main", "Init Files", "Init", "Save As", "Start Profile", "Check Step Time", "Alarm", "Run Step", "Stop Profile", "Cycle Reset", "Time Reset", "Time Reset All", "Time Set", "Tare CTs", "Save Profile", "Open Profile", "Get Profiles", "Update Screen", "Save Status", "Set Manual CMD", "Reset Restarts", "Reset Total Restarts", "Reset Cogs", "Disable Background", "Enable Background", "Get/Release Control", "Init AKLH", "Save AKLH", "Log Fuel Change", "Update Data Stream", "Init TenHz", "Read TenHz", "Remote Timer Reset", "Record Frequency Change", "Controller Change", "Get Alarms", "Init Alarms", "Save Alarms"]
              n101 = Unbundle By Name(w321) -> ("Alarm"=w320:bool)
            }
            frame 19 {
              w325 = T14[] [enum."Disable Background", enum."Time Reset All"] items=["Main", "Init Files", "Init", "Save As", "Start Profile", "Check Step Time", "Alarm", "Run Step", "Stop Profile", "Cycle Reset", "Time Reset", "Time Reset All", "Time Set", "Tare CTs", "Save Profile", "Open Profile", "Get Profiles", "Update Screen", "Save Status", "Set Manual CMD", "Reset Restarts", "Reset Total Restarts", "Reset Cogs", "Disable Background", "Enable Background", "Get/Release Control", "Init AKLH", "Save AKLH", "Log Fuel Change", "Update Data Stream", "Init TenHz", "Read TenHz", "Remote Timer Reset", "Record Frequency Change", "Controller Change", "Get Alarms", "Init Alarms", "Save Alarms"]
            }
            frame 20 {
              w329 = T14[] [enum."Save Status"] items=["Main", "Init Files", "Init", "Save As", "Start Profile", "Check Step Time", "Alarm", "Run Step", "Stop Profile", "Cycle Reset", "Time Reset", "Time Reset All", "Time Set", "Tare CTs", "Save Profile", "Open Profile", "Get Profiles", "Update Screen", "Save Status", "Set Manual CMD", "Reset Restarts", "Reset Total Restarts", "Reset Cogs", "Disable Background", "Enable Background", "Get/Release Control", "Init AKLH", "Save AKLH", "Log Fuel Change", "Update Data Stream", "Init TenHz", "Read TenHz", "Remote Timer Reset", "Record Frequency Change", "Controller Change", "Get Alarms", "Init Alarms", "Save Alarms"]
              n102 = Unbundle By Name(w330) -> ("App Config.Pumps Present"=w334:u32)
              n103 = Cluster To Array(cluster="Pumps Present") -> (array=w328:bool[])
              n104 = Boolean Array To Number(Boolean array=w328) -> (number=w326:u32)
              n105 = Not Equal?(x=w326, y=w334) -> (x != y?=w331:bool)
              n106 = Bundle By Name(cluster=w333, "App Config.Pumps Present"=w326) -> (w332:T17)
            }
            frame 21 {
              w336 = T14[] [enum."Get/Release Control"] items=["Main", "Init Files", "Init", "Save As", "Start Profile", "Check Step Time", "Alarm", "Run Step", "Stop Profile", "Cycle Reset", "Time Reset", "Time Reset All", "Time Set", "Tare CTs", "Save Profile", "Open Profile", "Get Profiles", "Update Screen", "Save Status", "Set Manual CMD", "Reset Restarts", "Reset Total Restarts", "Reset Cogs", "Disable Background", "Enable Background", "Get/Release Control", "Init AKLH", "Save AKLH", "Log Fuel Change", "Update Data Stream", "Init TenHz", "Read TenHz", "Remote Timer Reset", "Record Frequency Change", "Controller Change", "Get Alarms", "Init Alarms", "Save Alarms"]
              n107 = Unbundle By Name(w337) -> ("Login"=w341:bool)
              n108 = Not Equal?(x="Login", y=w341) -> (x != y?=w338:bool)
              n109 = Bundle By Name(cluster=w340, "Login"="Login") -> (w339:T17)
            }
            frame 22 {
              w343 = T14[] [enum."Save Status"] items=["Main", "Init Files", "Init", "Save As", "Start Profile", "Check Step Time", "Alarm", "Run Step", "Stop Profile", "Cycle Reset", "Time Reset", "Time Reset All", "Time Set", "Tare CTs", "Save Profile", "Open Profile", "Get Profiles", "Update Screen", "Save Status", "Set Manual CMD", "Reset Restarts", "Reset Total Restarts", "Reset Cogs", "Disable Background", "Enable Background", "Get/Release Control", "Init AKLH", "Save AKLH", "Log Fuel Change", "Update Data Stream", "Init TenHz", "Read TenHz", "Remote Timer Reset", "Record Frequency Change", "Controller Change", "Get Alarms", "Init Alarms", "Save Alarms"]
              n110 = Unbundle By Name(w344) -> ("App Config.Stagger Time (ms)"=w348:i32)
              n111 = Not Equal?(x="Stagger Time (ms):", y=w348) -> (x != y?=w345:bool)
              n112 = Bundle By Name(cluster=w347, "App Config.Stagger Time (ms)"="Stagger Time (ms):") -> (w346:T17)
            }
            frame 23 {
              w351 = T14[] [enum."Disable Background", enum."Reset Total Restarts"] items=["Main", "Init Files", "Init", "Save As", "Start Profile", "Check Step Time", "Alarm", "Run Step", "Stop Profile", "Cycle Reset", "Time Reset", "Time Reset All", "Time Set", "Tare CTs", "Save Profile", "Open Profile", "Get Profiles", "Update Screen", "Save Status", "Set Manual CMD", "Reset Restarts", "Reset Total Restarts", "Reset Cogs", "Disable Background", "Enable Background", "Get/Release Control", "Init AKLH", "Save AKLH", "Log Fuel Change", "Update Data Stream", "Init TenHz", "Read TenHz", "Remote Timer Reset", "Record Frequency Change", "Controller Change", "Get Alarms", "Init Alarms", "Save Alarms"]
            }
            frame 24 {
              w353 = T14[] [enum."Set Manual CMD"] items=["Main", "Init Files", "Init", "Save As", "Start Profile", "Check Step Time", "Alarm", "Run Step", "Stop Profile", "Cycle Reset", "Time Reset", "Time Reset All", "Time Set", "Tare CTs", "Save Profile", "Open Profile", "Get Profiles", "Update Screen", "Save Status", "Set Manual CMD", "Reset Restarts", "Reset Total Restarts", "Reset Cogs", "Disable Background", "Enable Background", "Get/Release Control", "Init AKLH", "Save AKLH", "Log Fuel Change", "Update Data Stream", "Init TenHz", "Read TenHz", "Remote Timer Reset", "Record Frequency Change", "Controller Change", "Get Alarms", "Init Alarms", "Save Alarms"]
              n113 = Unbundle By Name(w356) -> ("Press CMD"=w355:dbl)
              n114 = Not Equal?(x=w355, y="PressureCMD") -> (x != y?=w354:bool)
              n115 = Bundle By Name(cluster=w358, "Press CMD"="PressureCMD") -> (w357:T17)
            }
            frame 25 {
              w361 = T14[] [enum."Log Fuel Change"] items=["Main", "Init Files", "Init", "Save As", "Start Profile", "Check Step Time", "Alarm", "Run Step", "Stop Profile", "Cycle Reset", "Time Reset", "Time Reset All", "Time Set", "Tare CTs", "Save Profile", "Open Profile", "Get Profiles", "Update Screen", "Save Status", "Set Manual CMD", "Reset Restarts", "Reset Total Restarts", "Reset Cogs", "Disable Background", "Enable Background", "Get/Release Control", "Init AKLH", "Save AKLH", "Log Fuel Change", "Update Data Stream", "Init TenHz", "Read TenHz", "Remote Timer Reset", "Record Frequency Change", "Controller Change", "Get Alarms", "Init Alarms", "Save Alarms"]
            }
            frame 26 {
              w362 = T14[] [] items=["Main", "Init Files", "Init", "Save As", "Start Profile", "Check Step Time", "Alarm", "Run Step", "Stop Profile", "Cycle Reset", "Time Reset", "Time Reset All", "Time Set", "Tare CTs", "Save Profile", "Open Profile", "Get Profiles", "Update Screen", "Save Status", "Set Manual CMD", "Reset Restarts", "Reset Total Restarts", "Reset Cogs", "Disable Background", "Enable Background", "Get/Release Control", "Init AKLH", "Save AKLH", "Log Fuel Change", "Update Data Stream", "Init TenHz", "Read TenHz", "Remote Timer Reset", "Record Frequency Change", "Controller Change", "Get Alarms", "Init Alarms", "Save Alarms"]
            }
            frame 27 {
              w365 = T14[] [] items=["Main", "Init Files", "Init", "Save As", "Start Profile", "Check Step Time", "Alarm", "Run Step", "Stop Profile", "Cycle Reset", "Time Reset", "Time Reset All", "Time Set", "Tare CTs", "Save Profile", "Open Profile", "Get Profiles", "Update Screen", "Save Status", "Set Manual CMD", "Reset Restarts", "Reset Total Restarts", "Reset Cogs", "Disable Background", "Enable Background", "Get/Release Control", "Init AKLH", "Save AKLH", "Log Fuel Change", "Update Data Stream", "Init TenHz", "Read TenHz", "Remote Timer Reset", "Record Frequency Change", "Controller Change", "Get Alarms", "Init Alarms", "Save Alarms"]
            }
            frame 28 {
              w374 = T14[] [enum."Save Status"] items=["Main", "Init Files", "Init", "Save As", "Start Profile", "Check Step Time", "Alarm", "Run Step", "Stop Profile", "Cycle Reset", "Time Reset", "Time Reset All", "Time Set", "Tare CTs", "Save Profile", "Open Profile", "Get Profiles", "Update Screen", "Save Status", "Set Manual CMD", "Reset Restarts", "Reset Total Restarts", "Reset Cogs", "Disable Background", "Enable Background", "Get/Release Control", "Init AKLH", "Save AKLH", "Log Fuel Change", "Update Data Stream", "Init TenHz", "Read TenHz", "Remote Timer Reset", "Record Frequency Change", "Controller Change", "Get Alarms", "Init Alarms", "Save Alarms"]
              n116 = Unbundle By Name(w371) -> ("App Config.Tank 1 Fuel"=w370:string)
              n117 = Not Equal?(x=w370, y="Tank 1 Fuel Type") -> (x != y?=w368:bool)
              n118 = Bundle By Name(cluster=w373, "App Config.Tank 1 Fuel"="Tank 1 Fuel Type") -> (w372:T17)
            }
            frame 29 {
              w381 = T14[] [enum."Save Status"] items=["Main", "Init Files", "Init", "Save As", "Start Profile", "Check Step Time", "Alarm", "Run Step", "Stop Profile", "Cycle Reset", "Time Reset", "Time Reset All", "Time Set", "Tare CTs", "Save Profile", "Open Profile", "Get Profiles", "Update Screen", "Save Status", "Set Manual CMD", "Reset Restarts", "Reset Total Restarts", "Reset Cogs", "Disable Background", "Enable Background", "Get/Release Control", "Init AKLH", "Save AKLH", "Log Fuel Change", "Update Data Stream", "Init TenHz", "Read TenHz", "Remote Timer Reset", "Record Frequency Change", "Controller Change", "Get Alarms", "Init Alarms", "Save Alarms"]
              n119 = Unbundle By Name(w378) -> ("App Config.Tank 2 Fuel"=w376:string)
              n120 = Not Equal?(x=w376, y="Tank 2 Fuel Type") -> (x != y?=w377:bool)
              n121 = Bundle By Name(cluster=w380, "App Config.Tank 2 Fuel"="Tank 2 Fuel Type") -> (w379:T17)
            }
            frame 30 {
              w388 = T14[] [enum."Save Status"] items=["Main", "Init Files", "Init", "Save As", "Start Profile", "Check Step Time", "Alarm", "Run Step", "Stop Profile", "Cycle Reset", "Time Reset", "Time Reset All", "Time Set", "Tare CTs", "Save Profile", "Open Profile", "Get Profiles", "Update Screen", "Save Status", "Set Manual CMD", "Reset Restarts", "Reset Total Restarts", "Reset Cogs", "Disable Background", "Enable Background", "Get/Release Control", "Init AKLH", "Save AKLH", "Log Fuel Change", "Update Data Stream", "Init TenHz", "Read TenHz", "Remote Timer Reset", "Record Frequency Change", "Controller Change", "Get Alarms", "Init Alarms", "Save Alarms"]
              n122 = Unbundle By Name(w385) -> ("App Config.Serial Numbers"=w384:T31)
              n123 = Not Equal?(x=w384, y="Serial Numbers") -> (x != y?=w382:bool)
              n124 = Bundle By Name(cluster=w387, "App Config.Serial Numbers"="Serial Numbers") -> (w386:T17)
            }
            frame 31 {
              w389 = T14[] [enum."Save Status"] items=["Main", "Init Files", "Init", "Save As", "Start Profile", "Check Step Time", "Alarm", "Run Step", "Stop Profile", "Cycle Reset", "Time Reset", "Time Reset All", "Time Set", "Tare CTs", "Save Profile", "Open Profile", "Get Profiles", "Update Screen", "Save Status", "Set Manual CMD", "Reset Restarts", "Reset Total Restarts", "Reset Cogs", "Disable Background", "Enable Background", "Get/Release Control", "Init AKLH", "Save AKLH", "Log Fuel Change", "Update Data Stream", "Init TenHz", "Read TenHz", "Remote Timer Reset", "Record Frequency Change", "Controller Change", "Get Alarms", "Init Alarms", "Save Alarms"]
              n125 = Unbundle By Name(w396) -> ("Cog Limits:"=w391:i32[])
              n126 = Not Equal?(x="Cog Limits:", y=w391) -> (x != y?=w393:bool[])
              n127 = Or Array Elements(Boolean array=w393) -> (logical OR=w392:bool)
              n128 = Bundle By Name(cluster=w395, "Cog Limits:"="Cog Limits:") -> (w394:T17)
            }
            frame 32 {
              w397 = T14[] [enum."Save Status"] items=["Main", "Init Files", "Init", "Save As", "Start Profile", "Check Step Time", "Alarm", "Run Step", "Stop Profile", "Cycle Reset", "Time Reset", "Time Reset All", "Time Set", "Tare CTs", "Save Profile", "Open Profile", "Get Profiles", "Update Screen", "Save Status", "Set Manual CMD", "Reset Restarts", "Reset Total Restarts", "Reset Cogs", "Disable Background", "Enable Background", "Get/Release Control", "Init AKLH", "Save AKLH", "Log Fuel Change", "Update Data Stream", "Init TenHz", "Read TenHz", "Remote Timer Reset", "Record Frequency Change", "Controller Change", "Get Alarms", "Init Alarms", "Save Alarms"]
              n129 = local read "Cog Events:"() -> (w400:i32[])
              n130 = Unbundle By Name(w404) -> ("Cog Events"=w401:i32[])
              n131 = Not Equal?(x=w400, y=w401) -> (x != y?=w399:bool[])
              n132 = Bundle By Name(cluster=w403, "Cog Events"=w400) -> (w402:T17)
              n133 = Or Array Elements(Boolean array=w399) -> (logical OR=w398:bool)
            }
            frame 33 {
              w407 = T14[] [enum."Disable Background", enum."Reset Cogs"] items=["Main", "Init Files", "Init", "Save As", "Start Profile", "Check Step Time", "Alarm", "Run Step", "Stop Profile", "Cycle Reset", "Time Reset", "Time Reset All", "Time Set", "Tare CTs", "Save Profile", "Open Profile", "Get Profiles", "Update Screen", "Save Status", "Set Manual CMD", "Reset Restarts", "Reset Total Restarts", "Reset Cogs", "Disable Background", "Enable Background", "Get/Release Control", "Init AKLH", "Save AKLH", "Log Fuel Change", "Update Data Stream", "Init TenHz", "Read TenHz", "Remote Timer Reset", "Record Frequency Change", "Controller Change", "Get Alarms", "Init Alarms", "Save Alarms"]
            }
            frame 34 {
              n134 = call "Test Action Global.vi"() -> ("Data OUT"=w411:dbl, "Test Action OUT"=w413:T32)  [unwired: 10 in]
              n135 = case shown="\"Pump Cmd\"" w413 {
                selector: w413 -> [_ _ _ _ w440 w470]
                tunnel: [w415 w420 w422 w426 w433 w473] -> w414
                tunnel: w412 -> [_ _ _ _ w445 w472]
                tunnel: w411 -> [_ _ _ w431 w441 w471]
                tunnel: [w416 w421 w423 w429 w443 w469] -> w410
                tunnel: w409 -> [w416 w421 w423 w430 w444 w468]
                tunnel: [FALSE TRUE TRUE TRUE TRUE w465] -> w408
                frame "Idle", Default {
                  w415 = T14[] [] items=["Main", "Init Files", "Init", "Save As", "Start Profile", "Check Step Time", "Alarm", "Run Step", "Stop Profile", "Cycle Reset", "Time Reset", "Time Reset All", "Time Set", "Tare CTs", "Save Profile", "Open Profile", "Get Profiles", "Update Screen", "Save Status", "Set Manual CMD", "Reset Restarts", "Reset Total Restarts", "Reset Cogs", "Disable Background", "Enable Background", "Get/Release Control", "Init AKLH", "Save AKLH", "Log Fuel Change", "Update Data Stream", "Init TenHz", "Read TenHz", "Remote Timer Reset", "Record Frequency Change", "Controller Change", "Get Alarms", "Init Alarms", "Save Alarms"]
                }
                frame "Start" {
                  w420 = T14[] [enum."Start Profile"] items=["Main", "Init Files", "Init", "Save As", "Start Profile", "Check Step Time", "Alarm", "Run Step", "Stop Profile", "Cycle Reset", "Time Reset", "Time Reset All", "Time Set", "Tare CTs", "Save Profile", "Open Profile", "Get Profiles", "Update Screen", "Save Status", "Set Manual CMD", "Reset Restarts", "Reset Total Restarts", "Reset Cogs", "Disable Background", "Enable Background", "Get/Release Control", "Init AKLH", "Save AKLH", "Log Fuel Change", "Update Data Stream", "Init TenHz", "Read TenHz", "Remote Timer Reset", "Record Frequency Change", "Controller Change", "Get Alarms", "Init Alarms", "Save Alarms"]
                  n136 = local write "pb.Run Profile"(TRUE ("pb.Run Profile")) -> ()
                }
                frame "Stop" {
                  w422 = T14[] [enum."Stop Profile"] items=["Main", "Init Files", "Init", "Save As", "Start Profile", "Check Step Time", "Alarm", "Run Step", "Stop Profile", "Cycle Reset", "Time Reset", "Time Reset All", "Time Set", "Tare CTs", "Save Profile", "Open Profile", "Get Profiles", "Update Screen", "Save Status", "Set Manual CMD", "Reset Restarts", "Reset Total Restarts", "Reset Cogs", "Disable Background", "Enable Background", "Get/Release Control", "Init AKLH", "Save AKLH", "Log Fuel Change", "Update Data Stream", "Init TenHz", "Read TenHz", "Remote Timer Reset", "Record Frequency Change", "Controller Change", "Get Alarms", "Init Alarms", "Save Alarms"]
                }
                frame "Pump Cmd" {
                  w426 = T14[] [enum."Set Manual CMD"] items=["Main", "Init Files", "Init", "Save As", "Start Profile", "Check Step Time", "Alarm", "Run Step", "Stop Profile", "Cycle Reset", "Time Reset", "Time Reset All", "Time Set", "Tare CTs", "Save Profile", "Open Profile", "Get Profiles", "Update Screen", "Save Status", "Set Manual CMD", "Reset Restarts", "Reset Total Restarts", "Reset Cogs", "Disable Background", "Enable Background", "Get/Release Control", "Init AKLH", "Save AKLH", "Log Fuel Change", "Update Data Stream", "Init TenHz", "Read TenHz", "Remote Timer Reset", "Record Frequency Change", "Controller Change", "Get Alarms", "Init Alarms", "Save Alarms"]
                  n137 = Initialize Array(w431, 6 ("dimension size")) -> (w425:dbl[])
                  n138 = Bundle By Name(cluster=w430, "Manual CMDs"=w425) -> (w429:T17)
                  n139 = local write "Manual\nCMD"(w425) -> ()
                }
                frame "Pump 1 Enable".."Pump 6 Enable" {
                  w433 = T14[] [enum."Update Screen", enum."Save Status"] items=["Main", "Init Files", "Init", "Save As", "Start Profile", "Check Step Time", "Alarm", "Run Step", "Stop Profile", "Cycle Reset", "Time Reset", "Time Reset All", "Time Set", "Tare CTs", "Save Profile", "Open Profile", "Get Profiles", "Update Screen", "Save Status", "Set Manual CMD", "Reset Restarts", "Reset Total Restarts", "Reset Cogs", "Disable Background", "Enable Background", "Get/Release Control", "Init AKLH", "Save AKLH", "Log Fuel Change", "Update Data Stream", "Init TenHz", "Read TenHz", "Remote Timer Reset", "Record Frequency Change", "Controller Change", "Get Alarms", "Init Alarms", "Save Alarms"]
                  n140 = Unbundle By Name(w445) -> ("App Config.Pumps Present"=w442:u32)
                  n141 = case shown="\"Pump 1 Enable\", Default" w440 {
                    tunnel: w441 -> [w448 w451 w454 w457 w460 w463]
                    tunnel: [w447 w450 w453 w456 w459 w462] -> w439
                    tunnel: [0 ("index") 1 ("index") 2 ("index") 3 ("index") 4 ("index") 5 ("index")] -> w438
                    frame "Pump 1 Enable", Default {
                      n142 = Greater Than 0?(x=w448) -> (x > 0?=w447:bool)
                    }
                    frame "Pump 2 Enable" {
                      n143 = Greater Than 0?(x=w451) -> (x > 0?=w450:bool)
                    }
                    frame "Pump 3 Enable" {
                      n144 = Greater Than 0?(x=w454) -> (x > 0?=w453:bool)
                    }
                    frame "Pump 4 Enable" {
                      n145 = Greater Than 0?(x=w457) -> (x > 0?=w456:bool)
                    }
                    frame "Pump 5 Enable" {
                      n146 = Greater Than 0?(x=w460) -> (x > 0?=w459:bool)
                    }
                    frame "Pump 6 Enable" {
                      n147 = Greater Than 0?(x=w463) -> (x > 0?=w462:bool)
                    }
                  }
                  n148 = Number To Boolean Array(number=w442) -> (Boolean array=w437:bool[])
                  n149 = Replace Array Subset(array=w437, new element=w439, index=w438) -> (w436:bool[])
                  n150 = Array To Cluster(array=w436) -> (cluster=w435:T33)
                  n151 = local write "Pumps Present"(w435) -> ()
                  n152 = Boolean Array To Number(Boolean array=w436) -> (number=w434:u32)
                  n153 = Bundle By Name(cluster=w444, "App Config.Pumps Present"=w434) -> (w443:T17)
                }
                frame "Timer 1 Reset".."Timer 6 Reset" {
                  w473 = T14[] [enum."Remote Timer Reset"] items=["Main", "Init Files", "Init", "Save As", "Start Profile", "Check Step Time", "Alarm", "Run Step", "Stop Profile", "Cycle Reset", "Time Reset", "Time Reset All", "Time Set", "Tare CTs", "Save Profile", "Open Profile", "Get Profiles", "Update Screen", "Save Status", "Set Manual CMD", "Reset Restarts", "Reset Total Restarts", "Reset Cogs", "Disable Background", "Enable Background", "Get/Release Control", "Init AKLH", "Save AKLH", "Log Fuel Change", "Update Data Stream", "Init TenHz", "Read TenHz", "Remote Timer Reset", "Record Frequency Change", "Controller Change", "Get Alarms", "Init Alarms", "Save Alarms"]
                  n154 = Unbundle By Name(w472) -> ("pb.Resets"=w467:bool[])
                  n155 = case shown="\"Timer 1 Reset\", Default" w470 {
                    tunnel: w471 -> [w476 w479 w482 w485 w488 w491]
                    tunnel: [w475 w478 w481 w484 w487 w490] -> w465
                    tunnel: [0 ("index") 1 ("index") 2 ("index") 3 ("index") 4 ("index") 5 ("index")] -> w464
                    frame "Timer 1 Reset", Default {
                      n156 = Greater Than 0?(x=w476) -> (x > 0?=w475:bool)
                    }
                    frame "Timer 2 Reset" {
                      n157 = Greater Than 0?(x=w479) -> (x > 0?=w478:bool)
                    }
                    frame "Timer 3 Reset" {
                      n158 = Greater Than 0?(x=w482) -> (x > 0?=w481:bool)
                    }
                    frame "Timer 4 Reset" {
                      n159 = Greater Than 0?(x=w485) -> (x > 0?=w484:bool)
                    }
                    frame "Timer 5 Reset" {
                      n160 = Greater Than 0?(x=w488) -> (x > 0?=w487:bool)
                    }
                    frame "Timer 6 Reset" {
                      n161 = Greater Than 0?(x=w491) -> (x > 0?=w490:bool)
                    }
                  }
                  n162 = Replace Array Subset(array=w467, new element=w465, index=w464) -> (w466:bool[])
                  n163 = Bundle By Name(cluster=w468, "pb.Resets"=w466) -> (w469:T17)
                }
              }
            }
            frame 35 {
              w493 = T14[] [enum."Save Status", enum."Init TenHz"] items=["Main", "Init Files", "Init", "Save As", "Start Profile", "Check Step Time", "Alarm", "Run Step", "Stop Profile", "Cycle Reset", "Time Reset", "Time Reset All", "Time Set", "Tare CTs", "Save Profile", "Open Profile", "Get Profiles", "Update Screen", "Save Status", "Set Manual CMD", "Reset Restarts", "Reset Total Restarts", "Reset Cogs", "Disable Background", "Enable Background", "Get/Release Control", "Init AKLH", "Save AKLH", "Log Fuel Change", "Update Data Stream", "Init TenHz", "Read TenHz", "Remote Timer Reset", "Record Frequency Change", "Controller Change", "Get Alarms", "Init Alarms", "Save Alarms"]
              w494 = T14[] [enum."Save Status"] items=["Main", "Init Files", "Init", "Save As", "Start Profile", "Check Step Time", "Alarm", "Run Step", "Stop Profile", "Cycle Reset", "Time Reset", "Time Reset All", "Time Set", "Tare CTs", "Save Profile", "Open Profile", "Get Profiles", "Update Screen", "Save Status", "Set Manual CMD", "Reset Restarts", "Reset Total Restarts", "Reset Cogs", "Disable Background", "Enable Background", "Get/Release Control", "Init AKLH", "Save AKLH", "Log Fuel Change", "Update Data Stream", "Init TenHz", "Read TenHz", "Remote Timer Reset", "Record Frequency Change", "Controller Change", "Get Alarms", "Init Alarms", "Save Alarms"]
              n164 = Unbundle By Name(w499) -> ("TenHz Active?"=w497:bool)
              n165 = Not Equal?(x=w497, y="pb.TenHzSave") -> (x != y?=w498:bool)
              n166 = Greater?(x="pb.TenHzSave", y=w497) -> (0:w496:bool)
              n167 = Bundle By Name(cluster=w501, "TenHz Active?"="pb.TenHzSave") -> (w500:T17)
              n168 = Select(t=w493, s=w496, f=w494) -> (s? t:f=w495:T14[])
            }
            frame 36 {
              w502 = T14[] [enum."Record Frequency Change", enum."Save Status"] items=["Main", "Init Files", "Init", "Save As", "Start Profile", "Check Step Time", "Alarm", "Run Step", "Stop Profile", "Cycle Reset", "Time Reset", "Time Reset All", "Time Set", "Tare CTs", "Save Profile", "Open Profile", "Get Profiles", "Update Screen", "Save Status", "Set Manual CMD", "Reset Restarts", "Reset Total Restarts", "Reset Cogs", "Disable Background", "Enable Background", "Get/Release Control", "Init AKLH", "Save AKLH", "Log Fuel Change", "Update Data Stream", "Init TenHz", "Read TenHz", "Remote Timer Reset", "Record Frequency Change", "Controller Change", "Get Alarms", "Init Alarms", "Save Alarms"]
              n169 = Unbundle By Name(w508) -> ("App Config.TenHzFrequency"=w505:u32)
              n170 = Not Equal?(x="Record Frequency:", y=w505) -> (x != y?=w503:bool)
              n171 = Bundle By Name(cluster=w507, "App Config.TenHzFrequency"="Record Frequency:") -> (w506:T17)
            }
            frame 37 {
              w512 = T14[] [enum."Set Manual CMD", enum."Save Status"] items=["Main", "Init Files", "Init", "Save As", "Start Profile", "Check Step Time", "Alarm", "Run Step", "Stop Profile", "Cycle Reset", "Time Reset", "Time Reset All", "Time Set", "Tare CTs", "Save Profile", "Open Profile", "Get Profiles", "Update Screen", "Save Status", "Set Manual CMD", "Reset Restarts", "Reset Total Restarts", "Reset Cogs", "Disable Background", "Enable Background", "Get/Release Control", "Init AKLH", "Save AKLH", "Log Fuel Change", "Update Data Stream", "Init TenHz", "Read TenHz", "Remote Timer Reset", "Record Frequency Change", "Controller Change", "Get Alarms", "Init Alarms", "Save Alarms"]
              n172 = Unbundle By Name(w513) -> ("Power Relay"=w510:T2)
              n173 = Not Equal?(x="Power Relay", y=w510) -> (x != y?=w511:bool)
              n174 = Bundle By Name(cluster=w515, "Power Relay"="Power Relay") -> (w514:T17)
            }
            frame 38 {
              w522 = T14[] [enum."Set Manual CMD", enum."Save Status"] items=["Main", "Init Files", "Init", "Save As", "Start Profile", "Check Step Time", "Alarm", "Run Step", "Stop Profile", "Cycle Reset", "Time Reset", "Time Reset All", "Time Set", "Tare CTs", "Save Profile", "Open Profile", "Get Profiles", "Update Screen", "Save Status", "Set Manual CMD", "Reset Restarts", "Reset Total Restarts", "Reset Cogs", "Disable Background", "Enable Background", "Get/Release Control", "Init AKLH", "Save AKLH", "Log Fuel Change", "Update Data Stream", "Init TenHz", "Read TenHz", "Remote Timer Reset", "Record Frequency Change", "Controller Change", "Get Alarms", "Init Alarms", "Save Alarms"]
              n175 = Unbundle By Name(w520) -> ("Ignition Relay"=w517:T2)
              n176 = Not Equal?(x="Ignition Relay", y=w517) -> (x != y?=w521:bool)
              n177 = Bundle By Name(cluster=w519, "Ignition Relay"="Ignition Relay") -> (w518:T17)
            }
            frame 39 {
              n178 = local read "HMI Mom Buttons"() -> (w523:T1)
              n179 = flat-sequence {
                tunnel: w523 -> [_]
                frame #0 {
                  n180 = local write "HMI Mom Buttons"(T1 {"Stop"=FALSE, "Reset Timers"=FALSE, "Log Fuel Change"=FALSE} ("HMI Mom Buttons")) -> ()
                }
              }
              n181 = Cluster To Array(cluster=w523) -> (array=w527:bool[])
              n182 = Search 1D Array(1D array=w527, element=TRUE) -> (index of element=w525:i32)  [unwired: 1 in]
              n183 = case shown="0" w525 {
                tunnel: [w531 w532 w533 w534] -> w529
                frame -1, Default {
                  w531 = T14[] [] items=["Main", "Init Files", "Init", "Save As", "Start Profile", "Check Step Time", "Alarm", "Run Step", "Stop Profile", "Cycle Reset", "Time Reset", "Time Reset All", "Time Set", "Tare CTs", "Save Profile", "Open Profile", "Get Profiles", "Update Screen", "Save Status", "Set Manual CMD", "Reset Restarts", "Reset Total Restarts", "Reset Cogs", "Disable Background", "Enable Background", "Get/Release Control", "Init AKLH", "Save AKLH", "Log Fuel Change", "Update Data Stream", "Init TenHz", "Read TenHz", "Remote Timer Reset", "Record Frequency Change", "Controller Change", "Get Alarms", "Init Alarms", "Save Alarms"]
                }
                frame 0 {
                  w532 = T14[] [enum."Stop Profile"] items=["Main", "Init Files", "Init", "Save As", "Start Profile", "Check Step Time", "Alarm", "Run Step", "Stop Profile", "Cycle Reset", "Time Reset", "Time Reset All", "Time Set", "Tare CTs", "Save Profile", "Open Profile", "Get Profiles", "Update Screen", "Save Status", "Set Manual CMD", "Reset Restarts", "Reset Total Restarts", "Reset Cogs", "Disable Background", "Enable Background", "Get/Release Control", "Init AKLH", "Save AKLH", "Log Fuel Change", "Update Data Stream", "Init TenHz", "Read TenHz", "Remote Timer Reset", "Record Frequency Change", "Controller Change", "Get Alarms", "Init Alarms", "Save Alarms"]
                }
                frame 1 {
                  w533 = T14[] [enum."Remote Timer Reset"] items=["Main", "Init Files", "Init", "Save As", "Start Profile", "Check Step Time", "Alarm", "Run Step", "Stop Profile", "Cycle Reset", "Time Reset", "Time Reset All", "Time Set", "Tare CTs", "Save Profile", "Open Profile", "Get Profiles", "Update Screen", "Save Status", "Set Manual CMD", "Reset Restarts", "Reset Total Restarts", "Reset Cogs", "Disable Background", "Enable Background", "Get/Release Control", "Init AKLH", "Save AKLH", "Log Fuel Change", "Update Data Stream", "Init TenHz", "Read TenHz", "Remote Timer Reset", "Record Frequency Change", "Controller Change", "Get Alarms", "Init Alarms", "Save Alarms"]
                }
                frame 2 {
                  w534 = T14[] [enum."Log Fuel Change"] items=["Main", "Init Files", "Init", "Save As", "Start Profile", "Check Step Time", "Alarm", "Run Step", "Stop Profile", "Cycle Reset", "Time Reset", "Time Reset All", "Time Set", "Tare CTs", "Save Profile", "Open Profile", "Get Profiles", "Update Screen", "Save Status", "Set Manual CMD", "Reset Restarts", "Reset Total Restarts", "Reset Cogs", "Disable Background", "Enable Background", "Get/Release Control", "Init AKLH", "Save AKLH", "Log Fuel Change", "Update Data Stream", "Init TenHz", "Read TenHz", "Remote Timer Reset", "Record Frequency Change", "Controller Change", "Get Alarms", "Init Alarms", "Save Alarms"]
                }
              }
              n184 = Greater Or Equal To 0?(x=w525) -> (x >= 0?=w524:bool)
            }
            frame 40 {
              w541 = T14[] [enum."Save Alarms"] items=["Main", "Init Files", "Init", "Save As", "Start Profile", "Check Step Time", "Alarm", "Run Step", "Stop Profile", "Cycle Reset", "Time Reset", "Time Reset All", "Time Set", "Tare CTs", "Save Profile", "Open Profile", "Get Profiles", "Update Screen", "Save Status", "Set Manual CMD", "Reset Restarts", "Reset Total Restarts", "Reset Cogs", "Disable Background", "Enable Background", "Get/Release Control", "Init AKLH", "Save AKLH", "Log Fuel Change", "Update Data Stream", "Init TenHz", "Read TenHz", "Remote Timer Reset", "Record Frequency Change", "Controller Change", "Get Alarms", "Init Alarms", "Save Alarms"]
              n185 = Unbundle By Name(w539) -> ("Alarm Config"=w536:T7)
              n186 = Not Equal?(x="Alarm Config", y=w536) -> (x != y?=w540:bool)
              n187 = Bundle By Name(cluster=w538, "Alarm Config"="Alarm Config") -> (w537:T17)
            }
          }
        }
        n188 = Get Date/Time In Seconds() -> (seconds since 1Jan1904=w168:timestamp)
        n189 = To Double Precision Float(number=w168) -> (double precision float=w178:dbl)
        n190 = Subtract(x=w178, y=w192) -> (x-y=w182:dbl)
        n191 = Subtract(x=w178, y=w176) -> (x-y=w183:dbl)
        n192 = Subtract(x=w178, y=w175) -> (x-y=w184:dbl)
        n193 = case shown="True" w167 {
          selector: w167 -> [w194 _]
          tunnel: w168 -> [_ w198]
          tunnel: w166 -> [_ w196]
          tunnel: [w194 w195] -> w162
          frame False {
          }
          frame True {
            n194 = Seconds To Date/Time(time stamp (now)=w198) -> (date time rec=w199:T34)  [unwired: 1 in]
            n195 = Unbundle By Name(w199) -> ("day of month"=w197:i32)
            n196 = Not Equal?(x=w197, y=w196) -> (x != y?=w195:bool)
          }
        }
        n197 = Greater?(x=w182, y=0.5) -> (0:w186:bool)
        n198 = Greater?(x=w183, y=0.1) -> (0:w171:bool)
        n199 = Greater?(x=w184, y=600.0) -> (0:w170:bool)
        n200 = case shown="False" w189 {
          tunnel: w188 -> [w549 _]
          tunnel: [w543 w550] -> w180
          tunnel: w187 -> [_ w550]
          tunnel: w186 -> [w542 _]
          frame False {
            w546 = T14[] [enum."Check Step Time"] items=["Main", "Init Files", "Init", "Save As", "Start Profile", "Check Step Time", "Alarm", "Run Step", "Stop Profile", "Cycle Reset", "Time Reset", "Time Reset All", "Time Set", "Tare CTs", "Save Profile", "Open Profile", "Get Profiles", "Update Screen", "Save Status", "Set Manual CMD", "Reset Restarts", "Reset Total Restarts", "Reset Cogs", "Disable Background", "Enable Background", "Get/Release Control", "Init AKLH", "Save AKLH", "Log Fuel Change", "Update Data Stream", "Init TenHz", "Read TenHz", "Remote Timer Reset", "Record Frequency Change", "Controller Change", "Get Alarms", "Init Alarms", "Save Alarms"]
            n201 = Select(t=Sequence_States."Update Screen", s=w542, f=Sequence_States."Main") -> (s? t:f=w545:T14)
            n202 = Build Array(w545) -> (w544:T14[])
            n203 = Select(t=w546, s=w549, f=w544) -> (s? t:f=w543:T14[])
          }
          frame True {
          }
        }
        n204 = Select(t=Sequence_States."Init TenHz", s=w162, f=Sequence_States."Save AKLH") -> (s? t:f=w164:T14)
        n205 = Compound Arithmetic op=OR(w171, w170, w162) -> (w169:bool)
        n206 = Select(t=Sequence_States."Read TenHz", s=w171, f=w164) -> (s? t:f=w177:T14)
        n207 = Bundle By Name(cluster=w191, "Update Screen"=w186) -> (w193:T17)
        n208 = case shown="True" w169 {
          tunnel: w180 -> [w200 w204]
          tunnel: w177 -> [_ w203]
          tunnel: [w200 w201] -> w179
          frame False {
          }
          frame True {
            n209 = Insert Into Array(array=w204, index=0, new element=w203) -> (w201:T14[])
          }
        }
      }
      frame "Init Files" {
        # "changed tick divider to 1 as I was\nalready taking care of scaling\ntime when I do a data read that\nway data is only modified in one spot"
        n210 = Unbundle By Name(w573) -> ("App Config"=w560:T16, "AKLH Path"=w557:path, "TenHz Path"=w558:path)
        n211 = flat-sequence {
          tunnel: [errorcluster {"status"=FALSE, "code"=0, "source"=""} ("error in (no error)")] -> w554
          frame #0 {
            # "Hoping this helps avoid\nany file i/o errors."
            n212 = Wait (ms)(milliseconds to wait=u32 1000) -> ()  [unwired: 1 out]
          }
        }
        n213 = flat-sequence {
          tunnel: w565 -> [_]
          frame #0 {
            w622 = dbl[][] [[0.0, 11.0, 0.0, 0.0, 0.0], [0.0, 11.0, 0.0, 0.0, 0.0], [0.0, 11.0, 0.0, 0.0, 0.0], [0.0, 11.0, 0.0, 0.0, 0.0], [0.0, 11.0, 0.0, 0.0, 0.0], [0.0, 11.0, 0.0, 0.0, 0.0], [0.0, 1.0, 0.0, 0.0, 0.0], [0.0, 1.0, 0.0, 0.0, 0.0], [0.0, 1.0, 0.0, 0.0, 0.0], [0.0, 2.0, 0.0, 0.0, 0.0], [0.0, 1.0, 0.0, 0.0, 0.0], [0.0, 1.0, 0.0, 0.0, 0.0], [0.0, 1.0, 0.0, 0.0, 0.0], [0.0, 1.0, 0.0, 0.0, 0.0], [0.0, 1.0, 0.0, 0.0, 0.0], [0.0, 1.0, 0.0, 0.0, 0.0], [0.0, 1.0, 0.0, 0.0, 0.0], [0.0, 1.0, 0.0, 0.0, 0.0], [0.0, 1.0, 0.0, 0.0, 0.0], [0.0, 1.0, 0.0, 0.0, 0.0], [0.0, 1.0, 0.0, 0.0, 0.0], [0.0, 1.0, 0.0, 0.0, 0.0], [-60.0, 24.0, 0.0, 0.0, 0.0], [-60.0, 24.0, 0.0, 0.0, 0.0], [-60.0, 24.0, 0.0, 0.0, 0.0], [-60.0, 24.0, 0.0, 0.0, 0.0], [-60.0, 24.0, 0.0, 0.0, 0.0], [-60.0, 24.0, 0.0, 0.0, 0.0], [-660.0, 200.0, 0.0, 0.0, 0.0], [-660.0, 200.0, 0.0, 0.0, 0.0], [-258.5, 258.5, 0.0, 0.0, 0.0], [-258.5, 258.5, 0.0, 0.0, 0.0], [-258.5, 258.5, 0.0, 0.0, 0.0], [-258.5, 258.5, 0.0, 0.0, 0.0], [-258.5, 258.5, 0.0, 0.0, 0.0], [-258.5, 258.5, 0.0, 0.0, 0.0], [-150.0, 150.0, 0.0, 0.0, 0.0], [-150.0, 150.0, 0.0, 0.0, 0.0], [-150.0, 150.0, 0.0, 0.0, 0.0], [-150.0, 150.0, 0.0, 0.0, 0.0], [-150.0, 150.0, 0.0, 0.0, 0.0], [-150.0, 150.0, 0.0, 0.0, 0.0], [0.0, 1.0, 0.0, 0.0, 0.0], [0.0, 1.0, 0.0, 0.0, 0.0], [0.0, 1.0, 0.0, 0.0, 0.0], [0.0, 1.0, 0.0, 0.0, 0.0], [0.0, 1.0, 0.0, 0.0, 0.0], [0.0, 1.0, 0.0, 0.0, 0.0], [0.0, 0.0001, 0.0, 0.0, 0.0], [0.0, 0.0001, 0.0, 0.0, 0.0], [0.0, 0.0001, 0.0, 0.0, 0.0], [0.0, 0.0001, 0.0, 0.0, 0.0], [0.0, 0.0001, 0.0, 0.0, 0.0], [0.0, 0.0001, 0.0, 0.0, 0.0]]  # Cal Coefficients
            # "This is 10.30.189.0"
            n214 = String To IP() -> (0:w628:u32)  [unwired: 1 in]
            n215 = Subtract(x=w628, y=u32 169786624) -> (x-y=w627:u32)
            n216 = Number To Decimal String(number=w627) -> (decimal integer string=w626:string)  [unwired: 1 in]
            n217 = Concatenate Strings("c:\\" ("string"), w626, ".cal" ("string")) -> (w623:string)
            n218 = String To Path(string=w623) -> ()  [unwired: 1 out]
            n219 = call "Get Cal Coefficients.vi"("Path"=path "c:/160.cal") -> ("Error"=w630:bool, "Cal Coefficients"=w633:dbl[][])  [unwired: 9 in]
            n220 = case shown="False" w630 {
              tunnel: w633 -> [_ w637]
              tunnel: [w634 w636] -> w631
              tunnel: w622 -> [w634 w635]
              frame True {
              }
              frame False {
                n221 = for {
                  tunnel: w637 -> [w639] mode=indexing
                  shift-right: [w640] -> w636
                  shift-left: w635 -> [w641]
                  i -> [w638]
                  n222 = Index Array(array=w639) -> (element #1=w652:dbl, element #2=w651:dbl, element #3=w650:dbl, element #4=w646:dbl, element #5=w645:dbl)  [unwired: 5 in]
                  n223 = Equal To 0?(x=w652) -> (x = 0?=w649:bool)
                  n224 = Equal To 0?(x=w651) -> (x = 0?=w648:bool)
                  n225 = Equal To 0?(x=w650) -> (x = 0?=w647:bool)
                  n226 = Equal To 0?(x=w646) -> (x = 0?=w644:bool)
                  n227 = Equal To 0?(x=w645) -> (x = 0?=w643:bool)
                  n228 = Compound Arithmetic op=AND(w649, w648, w647, w644, w643) -> (w642:bool)
                  n229 = case shown="False" w642 {
                    tunnel: w641 -> [w656 w657]
                    tunnel: [w655 w657] -> w640
                    tunnel: w639 -> [w654 _]
                    tunnel: w638 -> [w653 _]
                    frame False {
                      n230 = Replace Array Subset(array=w656, new element=w654, index (row)=w653) -> (w655:dbl[][])  [unwired: 1 in]
                    }
                    frame True {
                    }
                  }
                }
              }
            }
            n231 = call "Tank Data Global.vi"("Pump Data Mode"=Pump_Data_Mode."Write Cal", "Cal Coefficients"=w631) -> ()  [unwired: 9 in, 1 out]
          }
        }
        n232 = Build Array(w557, w558) -> (w556:path[])
        n233 = call <vilib>:"Open Config Data.vi"("error in (no error)"=w554, "configuration file path"=path "c:/App Config.ini") -> ("error out"=w562:errorcluster, "file created?"=w559:bool, "refnum"=w563:T35)  [unwired: 7 in]
        n234 = case shown="True" w559 {
          tunnel: w563 -> [w608 w613]
          tunnel: w562 -> [w606 _]
          tunnel: w560 -> [w603 w620]
          tunnel: [w604 w618] -> w583
          tunnel: [w602 w610] -> w553
          frame False {
            # "Read App Config.ini"
            n235 = call "Read Write App Config.vi"("Error IN"=w606, "App Config IN"=w603, "Refnum in"=w608) -> ("Error OUT"=w605:errorcluster, "App Config OUT"=w604:T16, "Refnum out"=w607:T35)  [unwired: 6 in]
            n236 = call <vilib>:"Close Config Data.vi"("error in (no error)"=w605, "refnum"=w607) -> ("error out"=w609:errorcluster)  [unwired: 8 in, 1 out]
            n237 = call <vilib>:"Clear Errors.vi"("error in (no error)"=w609) -> ("error out"=w602:errorcluster)  [unwired: 6 in]
          }
          frame True {
            # "Doesn't exists, so create."
            n238 = Bundle By Name(cluster=w620, "Profiles Path"=path "c:/Profiles", "PWM Freq (Hz)"=100.0, "Pumps Present"=u32 63, "TenHzFrequency"=u32 1) -> (w618:T16)
            n239 = call "Read Write App Config.vi"("Write (F)"=TRUE, "App Config IN"=w618, "Refnum in"=w613) -> ("Error OUT"=w616:errorcluster, "Refnum out"=w617:T35)  [unwired: 6 in, 1 out]
            n240 = call <vilib>:"Close Config Data.vi"("error in (no error)"=w616, "refnum"=w617) -> ("error out"=w610:errorcluster)  [unwired: 8 in, 1 out]
          }
        }
        n241 = for {
          tunnel: w556 -> [w590] mode=indexing
          tunnel: [w589] -> w555 mode=indexing
          tunnel: w553 -> [w588]
          tunnel: [w587] -> w564
          n242 = call <vilib>:"Check if File or Folder Exists.vi"("error in (no error)"=w588, "path"=w590) -> ("error out"=w594:errorcluster, "file or folder exists?"=w593:bool, "dup path"=w595:path)  [unwired: 7 in]
          n243 = case shown="False" w593 {
            tunnel: w595 -> [w599 w601]
            tunnel: w594 -> [w597 w600]
            tunnel: [w598 w601] -> w591
            tunnel: [w596 w600] -> w587
            frame False {
              n244 = Create Folder(path (use dialog)=w599, error in=w597) -> (created path=w598:path, error out=w596:errorcluster)  [unwired: 1 in, 1 out]
            }
            frame True {
            }
          }
          n245 = Build Path(base path=w591, name or relative path="StartingPoint.csv") -> (appended path=w589:path)
        }
        n246 = Index Array(array=w555) -> (element #1=w574:path, element #2=w568:path)  [unwired: 2 in]
        n247 = call "Get Restarts Data.vi"("error in"=w564, "Path"=path "c:/Restarts" ("file (use dialog)")) -> ("Cogging Data"=w571:cluster{"CogEvents":i32[], "CogLimits":i32[]}, "Restarts Limits"=w578:T3, "Actual Starts"=w579:T15, "Restarts Cluster"=w580:T4, "error out"=w567:errorcluster)  [unwired: 5 in]
        n248 = call "Get Elapsed Times.vi"("error in"=w567, "Path"=path "c:/ElapsedTimes" ("file (use dialog)")) -> ("error out"=w566:errorcluster, "Elapsed Times"=w576:dbl[])  [unwired: 8 in]
        n249 = call "Get CT Offsets.vi"("error in"=w566, "Path"=path "c:/CT Offsets" ("file (use dialog)")) -> ("error out"=w565:errorcluster, "CT Offsets"=w581:fxp<+,24,6>[])  [unwired: 8 in]
        n250 = call "Elapsed Time Global.vi"("Write (F)"=TRUE, "Tick Divider"=1.0, "Initial Times IN"=w576) -> ()  [unwired: 8 in, 1 out]
        n251 = Unbundle(w571) -> ("CogEvents"=w569:i32[], "CogLimits"=w570:i32[])
        n252 = Bundle By Name(cluster=w573, "AKLH Path"=w574, "TenHz Path"=w568, "App Config"=w583, "Restarts Cluster"=w580, "Actual Starts"=w579, "Restarts Limits"=w578, "Intitial Times"=w576, "CT Offsets"=w581, "Cog Events"=w569, "Cog Limits:"=w570) -> (w572:T17)
        n253 = local write "Cog Events:"(w569) -> ()
        n254 = local write "Cog Limits:"(w570) -> ()
      }
      frame "Init" {
        w679 = T11 [{"Controller Name"=enum."Kuhnke", "CommSeg"=2, "PWM?"=TRUE, "Frequency"=100, "Low Command"=10.0, "High Command"=100.0, "Stop Command"=10.0, "Command Step"=0.1, "Solenoid Stop?"=FALSE, "Controller?"=FALSE, "Invert PWM"=TRUE}, {"Controller Name"=enum."Conti", "CommSeg"=2, "PWM?"=FALSE, "Frequency"=100, "Low Command"=0.0, "High Command"=800.0, "Stop Command"=0.0, "Command Step"=1.0, "Solenoid Stop?"=FALSE, "Controller?"=FALSE, "Invert PWM"=FALSE}, {"Controller Name"=enum."Helbako", "CommSeg"=2, "PWM?"=FALSE, "Frequency"=100, "Low Command"=0.0, "High Command"=100.0, "Stop Command"=0.0, "Command Step"=0.1, "Solenoid Stop?"=FALSE, "Controller?"=FALSE, "Invert PWM"=FALSE}, {"Controller Name"=enum."TI PWM", "CommSeg"=2, "PWM?"=TRUE, "Frequency"=100, "Low Command"=0.0, "High Command"=100.0, "Stop Command"=0.0, "Command Step"=0.1, "Solenoid Stop?"=FALSE, "Controller?"=FALSE, "Invert PWM"=FALSE}, {"Controller Name"=enum."PSA", "CommSeg"=2, "PWM?"=TRUE, "Frequency"=100, "Low Command"=5.0, "High Command"=95.0, "Stop Command"=5.0, "Command Step"=0.1, "Solenoid Stop?"=FALSE, "Controller?"=FALSE, "Invert PWM"=FALSE}, {"Controller Name"=enum."PSA", "CommSeg"=2, "PWM?"=FALSE, "Frequency"=100, "Low Command"=0.0, "High Command"=800.0, "Stop Command"=0.0, "Command Step"=1.0, "Solenoid Stop?"=TRUE, "Controller?"=FALSE, "Invert PWM"=FALSE}, {"Controller Name"=enum."Hella DC Gas", "CommSeg"=2, "PWM?"=FALSE, "Frequency"=100, "Low Command"=370.0, "High Command"=461.0, "Stop Command"=370.0, "Command Step"=1.0, "Solenoid Stop?"=TRUE, "Controller?"=FALSE, "Invert PWM"=FALSE}, {"Controller Name"=enum."8 Comm", "CommSeg"=8, "PWM?"=FALSE, "Frequency"=100, "Low Command"=0.0, "High Command"=1.0, "Stop Command"=0.0, "Command Step"=1.0, "Solenoid Stop?"=FALSE, "Controller?"=FALSE, "Invert PWM"=FALSE}, {"Controller Name"=enum."10 Comm", "CommSeg"=10, "PWM?"=FALSE, "Frequency"=100, "Low Command"=0.0, "High Command"=1.0, "Stop Command"=0.0, "Command Step"=1.0, "Solenoid Stop?"=FALSE, "Controller?"=FALSE, "Invert PWM"=FALSE}, {"Controller Name"=enum."8 Comm Hella", "CommSeg"=8, "PWM?"=TRUE, "Frequency"=150, "Low Command"=0.0, "High Command"=50.0, "Stop Command"=80.0, "Command Step"=0.1, "Solenoid Stop?"=FALSE, "Controller?"=FALSE, "Invert PWM"=FALSE}, {"Controller Name"=enum."10 Comm Hella", "CommSeg"=10, "PWM?"=TRUE, "Frequency"=150, "Low Command"=0.0, "High Command"=50.0, "Stop Command"=80.0, "Command Step"=0.1, "Solenoid Stop?"=FALSE, "Controller?"=FALSE, "Invert PWM"=FALSE}, {"Controller Name"=enum."8 Comm Omron", "CommSeg"=8, "PWM?"=TRUE, "Frequency"=150, "Low Command"=5.0, "High Command"=50.0, "Stop Command"=75.0, "Command Step"=0.1, "Solenoid Stop?"=FALSE, "Controller?"=FALSE, "Invert PWM"=FALSE}, {"Controller Name"=enum."10 Comm Omron", "CommSeg"=10, "PWM?"=TRUE, "Frequency"=150, "Low Command"=5.0, "High Command"=50.0, "Stop Command"=75.0, "Command Step"=0.1, "Solenoid Stop?"=FALSE, "Controller?"=FALSE, "Invert PWM"=FALSE}, {"Controller Name"=enum."8 Comm Nissan", "CommSeg"=8, "PWM?"=TRUE, "Frequency"=10, "Low Command"=50.0, "High Command"=90.0, "Stop Command"=50.0, "Command Step"=0.1, "Solenoid Stop?"=TRUE, "Controller?"=FALSE, "Invert PWM"=FALSE}, {"Controller Name"=enum."10 Comm Nissan", "CommSeg"=10, "PWM?"=TRUE, "Frequency"=10, "Low Command"=50.0, "High Command"=90.0, "Stop Command"=50.0, "Command Step"=0.1, "Solenoid Stop?"=TRUE, "Controller?"=FALSE, "Invert PWM"=FALSE}]  # Controller List
        w710 = T14[] [enum."Init AKLH", enum."Init TenHz", enum."Get Profiles", enum."Enable Background", enum."Get/Release Control", enum."Record Frequency Change", enum."Get Alarms"] items=["Main", "Init Files", "Init", "Save As", "Start Profile", "Check Step Time", "Alarm", "Run Step", "Stop Profile", "Cycle Reset", "Time Reset", "Time Reset All", "Time Set", "Tare CTs", "Save Profile", "Open Profile", "Get Profiles", "Update Screen", "Save Status", "Set Manual CMD", "Reset Restarts", "Reset Total Restarts", "Reset Cogs", "Disable Background", "Enable Background", "Get/Release Control", "Init AKLH", "Save AKLH", "Log Fuel Change", "Update Data Stream", "Init TenHz", "Read TenHz", "Remote Timer Reset", "Record Frequency Change", "Controller Change", "Get Alarms", "Init Alarms", "Save Alarms"]
        w712 = T14[] [enum."Init AKLH", enum."Get Profiles", enum."Enable Background", enum."Get/Release Control", enum."Record Frequency Change", enum."Get Alarms"] items=["Main", "Init Files", "Init", "Save As", "Start Profile", "Check Step Time", "Alarm", "Run Step", "Stop Profile", "Cycle Reset", "Time Reset", "Time Reset All", "Time Set", "Tare CTs", "Save Profile", "Open Profile", "Get Profiles", "Update Screen", "Save Status", "Set Manual CMD", "Reset Restarts", "Reset Total Restarts", "Reset Cogs", "Disable Background", "Enable Background", "Get/Release Control", "Init AKLH", "Save AKLH", "Log Fuel Change", "Update Data Stream", "Init TenHz", "Read TenHz", "Remote Timer Reset", "Record Frequency Change", "Controller Change", "Get Alarms", "Init Alarms", "Save Alarms"]
        w713 = 40000000.0  # 40 MHz
        n255 = Unbundle By Name(w705) -> ("App Config.TenHzFrequency"=w700:u32, "App Config.Profiles Path"=w704:path, "App Config.Record TenHz"=w691:bool, "App Config.Controller Type:"=w714:T5)
        n256 = local write "pb.Run Profile"(FALSE ("pb.Run Profile")) -> ()
        n257 = local write "Main Tab"(enum32{"Main", "Data Stream", "Alarms"}."Main" ("Main Tab")) -> ()
        n258 = Index Array(array=w679, index=w714) -> (element=w698:T12)
        n259 = local write "Record Frequency:"(w700) -> ()
        n260 = local write "pb.TenHzSave"(w691) -> ()
        n261 = Unbundle By Name(w698) -> ("High Command"=w703:dbl, "Low Command"=w702:dbl, "Command Step"=w701:dbl, "Stop Command"=w706:dbl, "CommSeg"=w694:i32, "Frequency"=w697:i32, "Invert PWM"=w680:bool, "Controller Name"=w671:T5)
        n262 = xnode "Invoke Method"("FPGA VI Reference In"=w709) -> ("FPGA VI Reference Out"=w708:T18)  [unwired: 1 in, 1 out]
        n263 = property on="Manual CMD" class="DigNum (strict)"("Maximum"=w703, "Minimum"=w702, "Increment"=w701) -> ()  [unwired: 2 in, 2 out]
        n264 = Divide(x=w694, y=2) -> (x/y=w693:dbl)
        n265 = To Fixed-Point(fixed-point type=fxp<+,32,16> 0.0 ("CommFactor"), number=w693) -> (fixed-point=w692:fxp<+,32,16>)
        n266 = Divide(x=w713, y=w697) -> (x/y=w670:dbl)
        n267 = Divide(x=w670, y=100.0) -> (x/y=w668:dbl)
        n268 = case shown="\"Kuhnke\"" w671 {
          tunnel: w668 -> [_ w732 w741 w746 w751]
          tunnel: [0 w731 w740 w745 w750] -> w667
          tunnel: [9 w730 9 w744 w749] -> w665
          tunnel: [4 w730 4 w744 w749] -> w664
          tunnel: [0 w730 0 w744 w749] -> w663
          tunnel: [230 w730 230 w744 w749] -> w662
          tunnel: [2147483647 w730 2147483647 w744 w749] -> w661
          tunnel: [0.0 w728 w733 w743 w747] -> w659
          frame Default {
          }
          frame "Kuhnke" {
            w730 = 0
            w728 = 10.0 ("y")
            n269 = Multiply(x=w732, y=w728) -> (x*y=w729:dbl)
            n270 = To Long Integer(number=w729) -> (32bit integer=w731:i32)
          }
          frame "PSA" {
            w733 = 5.0 ("y")
            n271 = Multiply(x=w741, y=w733) -> (x*y=w734:dbl)
            n272 = To Long Integer(number=w734) -> (32bit integer=w740:i32)
          }
          frame "8 Comm Hella", "10 Comm Hella" {
            w744 = 0
            w743 = 80.0 ("y")
            n273 = Multiply(x=w746, y=w743) -> (x*y=w742:dbl)
            n274 = To Long Integer(number=w742) -> (32bit integer=w745:i32)
          }
          frame "8 Comm Omron", "10 Comm Omron" {
            w749 = 0
            w747 = 75.0 ("y")
            n275 = Multiply(x=w751, y=w747) -> (x*y=w748:dbl)
            n276 = To Long Integer(number=w748) -> (32bit integer=w750:i32)
          }
        }
        n277 = To Unsigned Long Integer(number=w670) -> (unsigned 32bit integer=w720:u32)
        n278 = disable-structure shown="Enabled" {
          disable-tunnel: w720 -> [w767 w782]
          disable-tunnel: u32 100 ("Loop Timer (uSec)") -> [w766 w781]
          disable-tunnel: w708 -> [w765 w785]
          disable-tunnel: u32 4000000 ("x") -> [w764 _]
          disable-tunnel: w692 -> [w763 _]
          disable-tunnel: [w762 w784] -> w686
          disable-tunnel: [w761 w783] -> w685
          disable-tunnel: fxp<+/-,16,9> -121.7265625 ("PumpCurrentB") -> [w760 _]
          disable-tunnel: fxp<+/-,16,9> 74.5546875 ("PumpCurrentM") -> [w759 _]
          disable-tunnel: w680 -> [w758 _]
          disable-tunnel: fxp<+/-,24,6> 1.5 ("Threshold") -> [_ w780]
          disable-tunnel: 33 ("Period Delta") -> [_ w779]
          disable-tunnel: 500 ("Consec Samples") -> [_ w778]
          disable-tunnel: fxp<+,16,5> 24.0 ("Current Scale") -> [_ w777]
          disable-tunnel: fxp<+,23,5> 1.0 ("Speed Hysteresis") -> [_ w776]
          disable-tunnel: fxp<+/-,18,7> -60.0 ("Current Offset") -> [_ w775]
          disable-tunnel: w667 -> [_ w774]
          disable-tunnel: FALSE ("PS Control") -> [_ w773]
          disable-tunnel: w665 -> [_ w772]
          disable-tunnel: w664 -> [_ w771]
          disable-tunnel: w663 -> [_ w770]
          disable-tunnel: w662 -> [_ w769]
          disable-tunnel: w661 -> [_ w768]
          frame Disabled {
            n279 = xnode "Read/Write Control"("FPGA VI Reference In"=w765, "PWM Period (Ticks)"=w767, "Loop Timer (uSec)"=w766, "AI Divisor"=w764, "CommFactor"=w763, "InvertPWM?"=w758, "PumpCurrentB"=w760, "PumpCurrentM"=w759) -> ("FPGA VI Reference Out"=w762:T18, "error out"=w761:errorcluster)  [unwired: 1 in]
          }
          frame Enabled {
            n280 = xnode "Read/Write Control"("FPGA VI Reference In"=w785, "PWM Period (Ticks)"=w782, "Loop Timer (uSec)"=w781, "Threshold"=w780, "Kuhnke Window"=w779, "Consec Samples"=w778, "Current Scale"=w777, "Current Offset"=w775, "Speed Hysteresis"=w776, "Arm Level"=w772, "Disarm Level"=w771, "Spike Window"=w770, "Min Window"=w769, "Max Window"=w768, "Duty (Ticks) 1"=w774, "Duty (Ticks) 2"=w774, "Duty (Ticks) 3"=w774, "Duty (Ticks) 4"=w774, "Duty (Ticks) 5"=w774, "Duty (Ticks) 6"=w774, "PS Control"=w773) -> ("FPGA VI Reference Out"=w784:T18, "error out"=w783:errorcluster)  [unwired: 1 in]
          }
        }
        n281 = call <vilib>:"Check if File or Folder Exists.vi"("path"=w704) -> ("file or folder exists?"=w719:bool, "dup path"=w718:path)  [unwired: 8 in, 1 out]
        n282 = disable-structure shown="Enabled" {
          disable-tunnel: w686 -> [w755 w757]
          disable-tunnel: w685 -> [w754 w756]
          disable-tunnel: [w753 w757] -> w684
          disable-tunnel: [w752 w756] -> w683
          frame Disabled {
            n283 = call "Init FPGA.vi"("error in (no error)"=w754, "FPGA Ref"=w755) -> ("error out"=w752:errorcluster, "FPGA Ref OUT"=w753:T18)  [unwired: 8 in]
          }
          frame Enabled {
          }
        }
        n284 = Initialize Array(w659, 6 ("dimension size")) -> (w658:dbl[])
        n285 = case shown="False" w719 {
          tunnel: w718 -> [w791 _]
          frame False {
            n286 = Create Folder(path (use dialog)=w791) -> ()  [unwired: 2 in, 3 out]
          }
          frame True {
          }
        }
        n287 = xnode "Invoke Method"("FPGA VI Reference In"=w684, "error in"=w683, "Wait Until Done (F)"=FALSE) -> ("FPGA VI Reference Out"=w690:T18, "error out"=w688:errorcluster)
        n288 = Bundle By Name(cluster=w705, "Controller List"=w679, "Stop Cmd"=w706, "Manual CMDs"=w658, "Last CMDs"=w658) -> (w707:T17)
        n289 = local write "Manual\nCMD"(w658) -> ()
        n290 = flat-sequence {
          tunnel: w690 -> [w786]
          tunnel: w689 -> [w787]
          tunnel: w688 -> [w788]
          tunnel: [w787] -> w687
          frame #0 {
            n291 = disable-structure shown="Disabled" {
              disable-tunnel: w788 -> [w790 _]
              disable-tunnel: w786 -> [w789 _]
              frame Disabled {
                n292 = call "Init ADCs.vi"("Error IN"=w790, "FPGA Ref"=w789) -> ()  [unwired: 7 in, 3 out]
              }
              frame Enabled {
              }
            }
          }
        }
        n293 = Set Occurrence(w687) -> ()
        n294 = Select(t=w710, s=w691, f=w712) -> (s? t:f=w711:T14[])
      }
      frame "Get Alarms" {
        n295 = Unbundle By Name(w799) -> ("Alarm Config"=w800:T7, "Alarm Config Path"=w797:path)
        n296 = call <vilib>:"Check if File or Folder Exists.vi"("path"=w797) -> ("file or folder exists?"=w802:bool, "dup path"=w801:path)  [unwired: 8 in, 1 out]
        n297 = case shown="False" w802 {
          tunnel: w801 -> [w807 w812]
          tunnel: w800 -> [_ w810]
          tunnel: [w804 w808] -> w792
          frame False {
            w804 = T7 {"Alarms:"=[{"Description:"="", "Enabled:"=FALSE, "Data Index:"=0, "Data Type:"="", "Low Limit:"=0.0, "High Limit:"=0.0, "Trip Time:"=0, "Profile Sync:"=FALSE}, {"Description:"="", "Enabled:"=FALSE, "Data Index:"=0, "Data Type:"="", "Low Limit:"=0.0, "High Limit:"=0.0, "Trip Time:"=0, "Profile Sync:"=FALSE}, {"Description:"="", "Enabled:"=FALSE, "Data Index:"=0, "Data Type:"="", "Low Limit:"=0.0, "High Limit:"=0.0, "Trip Time:"=0, "Profile Sync:"=FALSE}, {"Description:"="", "Enabled:"=FALSE, "Data Index:"=0, "Data Type:"="", "Low Limit:"=0.0, "High Limit:"=0.0, "Trip Time:"=0, "Profile Sync:"=FALSE}, {"Description:"="", "Enabled:"=FALSE, "Data Index:"=0, "Data Type:"="", "Low Limit:"=0.0, "High Limit:"=0.0, "Trip Time:"=0, "Profile Sync:"=FALSE}, {"Description:"="", "Enabled:"=FALSE, "Data Index:"=0, "Data Type:"="", "Low Limit:"=0.0, "High Limit:"=0.0, "Trip Time:"=0, "Profile Sync:"=FALSE}, {"Description:"="", "Enabled:"=FALSE, "Data Index:"=0, "Data Type:"="", "Low Limit:"=0.0, "High Limit:"=0.0, "Trip Time:"=0, "Profile Sync:"=FALSE}, {"Description:"="", "Enabled:"=FALSE, "Data Index:"=0, "Data Type:"="", "Low Limit:"=0.0, "High Limit:"=0.0, "Trip Time:"=0, "Profile Sync:"=FALSE}], "Profile Sync:"={"Trip Time:"=0, "Consecutive Trips:"=0}} ("Alarm Config")
            n298 = Flatten To JSON(anything=w804) -> (JSON string=w803:string)  [unwired: 2 in, 1 out]
            n299 = Write to Text File(file (use dialog)=w807, text=w803) -> (refnum out=w806:refnum<file>, error out=w805:errorcluster)  [unwired: 2 in, 1 out]
            n300 = Close File(refnum=w806, error in=w805) -> ()  [unwired: 2 out]
          }
          frame True {
            n301 = Read from Text File(file (use dialog)=w812) -> (refnum out=w809:refnum<file>, text=w811:string)  [unwired: 3 in, 2 out]
            n302 = Close File(refnum=w809) -> ()  [unwired: 1 in, 2 out]
            n303 = Unflatten From JSON(JSON string=w811, type and defaults=w810) -> (value=w808:T7)  [unwired: 5 in, 1 out]
          }
        }
        n304 = Bundle By Name(cluster=w799, "Alarm Config"=w792) -> (w798:T17)
        n305 = local write "Alarm Config"(w792) -> ()
        n306 = Insert Into Array(array=w793, index=0, new element=Sequence_States."Init Alarms") -> (w794:T14[])
      }
      frame "Init Alarms" {
        # "Initialize alarm arrays."
        n307 = Unbundle By Name(w819) -> ("Alarm Config.Alarms:"=w821:T8[])
        n308 = for {
          tunnel: w821 -> [w828] mode=indexing
          shift-right: [w824] -> w815
          shift-left: 0 -> [w823]
          n309 = Unbundle By Name(w828) -> ("Data Type:"=w827:string, "Enabled:"=w826:bool)
          n310 = case shown="\"Pump\", Default" w827 {
            tunnel: [6 1] -> w825
            frame "Pump", Default {
            }
            frame "Tank" {
            }
          }
          n311 = case shown="True" w826 {
            tunnel: w825 -> [_ w832]
            tunnel: [w829 w831] -> w824
            tunnel: w823 -> [w829 w830]
            frame False {
            }
            frame True {
              n312 = Add(x=w832, y=w830) -> (x+y=w831:i32)
            }
          }
        }
        n313 = Tick Count (ms)() -> (millisecond timer value=w816:u32)
        n314 = Initialize Array(0, w815) -> (w814:i32[])
        n315 = Initialize Array(w816, w815) -> (w813:u32[])
        n316 = Bundle By Name(cluster=w819, "Trip Counters"=w814, "Previous Times"=w813, "Prev ON Times"=w813) -> (w818:T17)
      }
      frame "Save Alarms" {
        n317 = Unbundle By Name(w838) -> ("Alarm Config Path"=w836:path, "Alarm Config"=w837:T7)
        n318 = Flatten To JSON(anything=w837) -> (JSON string=w835:string)  [unwired: 2 in, 1 out]
        n319 = Write to Text File(file (use dialog)=w836, text=w835) -> ()  [unwired: 2 in, 3 out]
      }
      frame "Get Profiles" {
        n320 = Unbundle By Name(w847) -> ("App Config.Profiles Path"=w848:path)
        n321 = List Folder(path=w848) -> (filenames=w845:string[], error out=w844:errorcluster)  [unwired: 3 in, 2 out]
        n322 = call <vilib>:"Clear Errors.vi"("error in (no error)"=w844) -> ()  [unwired: 6 in, 1 out]
        n323 = property on="Profile Name:" class="CmbBox"("Strings[]"=w845) -> ()  [unwired: 2 in, 2 out]
        n324 = Bundle By Name(cluster=w847, "Profiles"=w845) -> (w846:T17)
        n325 = Insert Into Array(array=w841, index=0, new element=Sequence_States."Open Profile") -> (w840:T14[])
      }
      frame "Open Profile" {
        w850 = T14[] [enum."Update Screen", enum."Save Status"] items=["Main", "Init Files", "Init", "Save As", "Start Profile", "Check Step Time", "Alarm", "Run Step", "Stop Profile", "Cycle Reset", "Time Reset", "Time Reset All", "Time Set", "Tare CTs", "Save Profile", "Open Profile", "Get Profiles", "Update Screen", "Save Status", "Set Manual CMD", "Reset Restarts", "Reset Total Restarts", "Reset Cogs", "Disable Background", "Enable Background", "Get/Release Control", "Init AKLH", "Save AKLH", "Log Fuel Change", "Update Data Stream", "Init TenHz", "Read TenHz", "Remote Timer Reset", "Record Frequency Change", "Controller Change", "Get Alarms", "Init Alarms", "Save Alarms"]
        n326 = Unbundle By Name(w863) -> ("App Config.Profiles Path"=w865:path, "App Config.Current Profile"=w864:string)
        n327 = Build Path(base path=w865, name or relative path=w864) -> (appended path=w860:path)
        n328 = Read from Text File(file (use dialog)=w860) -> (refnum out=w858:refnum<file>, text=w859:string, error out=w857:errorcluster)  [unwired: 3 in, 1 out]
        n329 = Close File(refnum=w858, error in=w857) -> (error out=w856:errorcluster)  [unwired: 1 out]
        n330 = case shown="No Error" w856 {
          tunnel: w859 -> [w867 _]
          tunnel: [w868 string[][] []] -> w849
          frame No Error {
            n331 = Spreadsheet String To Array(delimiter (Tab)=",", format string="%s", spreadsheet string=w867, array type (2D Dbl)=string[][] []) -> (array=w868:string[][])
          }
          frame Error {
          }
        }
        n332 = Array Size(array=w849) -> (size(s)=w861:i32[])
        n333 = Index Array(array=w861) -> (element=w854:i32)  [unwired: 1 in]
        n334 = Bundle By Name(cluster=w863, "Profile"=w849, "# of Steps"=w854, "Update Profile"=TRUE) -> (w862:T17)
        n335 = Insert Into Array(array=w852, index=0, new element=w850) -> (w851:T14[])
      }
      frame "Save Profile" {
        n336 = Unbundle By Name(w878) -> ("App Config.Profiles Path"=w882:path, "App Config.Current Profile"=w880:string, "Profile"=w881:string[][])
        n337 = Empty String/Path?(string/path=w880) -> (empty?=w879:bool)
        n338 = case shown="False" w879 {
          tunnel: w882 -> [w887 _]
          tunnel: w880 -> [w886 _]
          tunnel: w881 -> [w885 _]
          tunnel: [w884 string[][] [] ("Profile OUT")] -> w874
          tunnel: [w883 w888] -> w876
          frame False {
            w883 = T14[] [enum."Update Screen"] items=["Main", "Init Files", "Init", "Save As", "Start Profile", "Check Step Time", "Alarm", "Run Step", "Stop Profile", "Cycle Reset", "Time Reset", "Time Reset All", "Time Set", "Tare CTs", "Save Profile", "Open Profile", "Get Profiles", "Update Screen", "Save Status", "Set Manual CMD", "Reset Restarts", "Reset Total Restarts", "Reset Cogs", "Disable Background", "Enable Background", "Get/Release Control", "Init AKLH", "Save AKLH", "Log Fuel Change", "Update Data Stream", "Init TenHz", "Read TenHz", "Remote Timer Reset", "Record Frequency Change", "Controller Change", "Get Alarms", "Init Alarms", "Save Alarms"]
            n339 = call "Save Profile.vi"("Profile"=w885, "Current Profile"=w886, "Profiles Path"=w887) -> ("Profile OUT"=w884:string[][])  [unwired: 8 in]
          }
          frame True {
            w888 = T14[] [enum."Main"] items=["Main", "Init Files", "Init", "Save As", "Start Profile", "Check Step Time", "Alarm", "Run Step", "Stop Profile", "Cycle Reset", "Time Reset", "Time Reset All", "Time Set", "Tare CTs", "Save Profile", "Open Profile", "Get Profiles", "Update Screen", "Save Status", "Set Manual CMD", "Reset Restarts", "Reset Total Restarts", "Reset Cogs", "Disable Background", "Enable Background", "Get/Release Control", "Init AKLH", "Save AKLH", "Log Fuel Change", "Update Data Stream", "Init TenHz", "Read TenHz", "Remote Timer Reset", "Record Frequency Change", "Controller Change", "Get Alarms", "Init Alarms", "Save Alarms"]
          }
        }
        n340 = Array Size(array=w874) -> (size(s)=w875:i32[])
        n341 = Index Array(array=w875) -> (element=w873:i32)  [unwired: 1 in]
        n342 = Bundle By Name(cluster=w878, "Profile"=w874, "# of Steps"=w873, "Update Profile"=TRUE) -> (w877:T17)
      }
      frame "Start Profile" {
        w891 = T14[] [enum."Init Alarms", enum."Check Step Time"] items=["Main", "Init Files", "Init", "Save As", "Start Profile", "Check Step Time", "Alarm", "Run Step", "Stop Profile", "Cycle Reset", "Time Reset", "Time Reset All", "Time Set", "Tare CTs", "Save Profile", "Open Profile", "Get Profiles", "Update Screen", "Save Status", "Set Manual CMD", "Reset Restarts", "Reset Total Restarts", "Reset Cogs", "Disable Background", "Enable Background", "Get/Release Control", "Init AKLH", "Save AKLH", "Log Fuel Change", "Update Data Stream", "Init TenHz", "Read TenHz", "Remote Timer Reset", "Record Frequency Change", "Controller Change", "Get Alarms", "Init Alarms", "Save Alarms"]
        w890 = 0 ("Current Step")
        n343 = property on="Main Tab" class="TabCtl (strict)"("DisabledEnum"=T27."Disabled" ("Disabled")) -> ()  [unwired: 2 in, 2 out]
        n344 = Get Date/Time In Seconds() -> (seconds since 1Jan1904=w895:timestamp)
        n345 = To Double Precision Float(number=w895) -> (double precision float=w894:dbl)
        n346 = Bundle By Name(cluster=w898, "Run Profile"=TRUE, "Step Start Time"=w894, "Last Profile Time"=w894, "Step Time"=0.0, "Current Step"=w890, "Stagger Counter"=w890) -> (w897:T17)
      }
      frame "Check Step Time" {
        # "Time elapsed since\nstart of step."
        n347 = Unbundle By Name(w921) -> ("Step Start Time"=w924:dbl, "Step Time"=w922:dbl, "Current Step"=w917:i32, "App Config.Stagger Time (ms)"=w900:i32, "Stagger Counter"=w906:i32, "Update Screen"=w915:bool)
        n348 = Get Date/Time In Seconds() -> (seconds since 1Jan1904=w923:timestamp)
        n349 = Increment(x=w906) -> (x+1=w901:i32)
        n350 = To Double Precision Float(number=w923) -> (double precision float=w914:dbl)
        n351 = Multiply(x=w900, y=w901) -> (x*y=w912:i32)
        n352 = Subtract(x=w914, y=w924) -> (x-y=w911:dbl)
        n353 = To Double Precision Float(number=w912) -> (double precision float=w905:dbl)
        n354 = Divide(x=w905, y=1000.0) -> (x/y=w903:dbl)
        n355 = Not Equal To 0?(x=w900) -> (x != 0?=w899:bool)
        n356 = Greater Or Equal?(x=w911, y=w903) -> (x >= y?=w910:bool)
        n357 = Less Or Equal?(x=w906, y=4) -> (x <= y?=w908:bool)
        n358 = Subtract(x=w922, y=w911) -> (x-y=w919:dbl)
        n359 = Compound Arithmetic op=AND(w910, w908, w899) -> (w907:bool)
        n360 = Less Or Equal To 0?(x=w919) -> (x <= 0?=w902:bool)
        n361 = case shown="False" w902 {
          tunnel: [w929 w940] -> w918
          tunnel: w917 -> [w930 w942]
          tunnel: [w930 w941] -> w916
          tunnel: w915 -> [w928 _]
          tunnel: [w925 0 ("Stagger Counter")] -> w913
          tunnel: w907 -> [w927 _]
          tunnel: w906 -> [w926 _]
          frame False {
            # "There's time left.  Update screen."
            n362 = case shown="True" w927 {
              tunnel: [w935 w938] -> w929
              tunnel: w928 -> [w934 _]
              tunnel: w926 -> [w931 w937]
              tunnel: [w931 w936] -> w925
              frame False {
                w932 = T14[] [enum."Main"] items=["Main", "Init Files", "Init", "Save As", "Start Profile", "Check Step Time", "Alarm", "Run Step", "Stop Profile", "Cycle Reset", "Time Reset", "Time Reset All", "Time Set", "Tare CTs", "Save Profile", "Open Profile", "Get Profiles", "Update Screen", "Save Status", "Set Manual CMD", "Reset Restarts", "Reset Total Restarts", "Reset Cogs", "Disable Background", "Enable Background", "Get/Release Control", "Init AKLH", "Save AKLH", "Log Fuel Change", "Update Data Stream", "Init TenHz", "Read TenHz", "Remote Timer Reset", "Record Frequency Change", "Controller Change", "Get Alarms", "Init Alarms", "Save Alarms"]
                w933 = T14[] [enum."Update Screen"] items=["Main", "Init Files", "Init", "Save As", "Start Profile", "Check Step Time", "Alarm", "Run Step", "Stop Profile", "Cycle Reset", "Time Reset", "Time Reset All", "Time Set", "Tare CTs", "Save Profile", "Open Profile", "Get Profiles", "Update Screen", "Save Status", "Set Manual CMD", "Reset Restarts", "Reset Total Restarts", "Reset Cogs", "Disable Background", "Enable Background", "Get/Release Control", "Init AKLH", "Save AKLH", "Log Fuel Change", "Update Data Stream", "Init TenHz", "Read TenHz", "Remote Timer Reset", "Record Frequency Change", "Controller Change", "Get Alarms", "Init Alarms", "Save Alarms"]
                n363 = Select(t=w933, s=w934, f=w932) -> (s? t:f=w935:T14[])
              }
              frame True {
                w938 = T14[] [enum."Run Step"] items=["Main", "Init Files", "Init", "Save As", "Start Profile", "Check Step Time", "Alarm", "Run Step", "Stop Profile", "Cycle Reset", "Time Reset", "Time Reset All", "Time Set", "Tare CTs", "Save Profile", "Open Profile", "Get Profiles", "Update Screen", "Save Status", "Set Manual CMD", "Reset Restarts", "Reset Total Restarts", "Reset Cogs", "Disable Background", "Enable Background", "Get/Release Control", "Init AKLH", "Save AKLH", "Log Fuel Change", "Update Data Stream", "Init TenHz", "Read TenHz", "Remote Timer Reset", "Record Frequency Change", "Controller Change", "Get Alarms", "Init Alarms", "Save Alarms"]
                n364 = Increment(x=w937) -> (x+1=w936:i32)
              }
            }
          }
          frame True {
            w940 = T14[] [enum."Run Step"] items=["Main", "Init Files", "Init", "Save As", "Start Profile", "Check Step Time", "Alarm", "Run Step", "Stop Profile", "Cycle Reset", "Time Reset", "Time Reset All", "Time Set", "Tare CTs", "Save Profile", "Open Profile", "Get Profiles", "Update Screen", "Save Status", "Set Manual CMD", "Reset Restarts", "Reset Total Restarts", "Reset Cogs", "Disable Background", "Enable Background", "Get/Release Control", "Init AKLH", "Save AKLH", "Log Fuel Change", "Update Data Stream", "Init TenHz", "Read TenHz", "Remote Timer Reset", "Record Frequency Change", "Controller Change", "Get Alarms", "Init Alarms", "Save Alarms"]
            # "No time left.  Go to next step."
            n365 = Increment(x=w942) -> (x+1=w941:i32)
          }
        }
        n366 = Bundle By Name(cluster=w921, "Last Profile Time"=w914, "Step Time Left"=w919, "New Step"=w902, "Current Step"=w916, "Stagger Counter"=w913) -> (w920:T17)
      }
      frame "Run Step" {
        n367 = Unbundle By Name(w969) -> ("App Config.VoltCtrlRef"=w946:string, "Profile"=w971:string[][], "Current Step"=w965:i32, "# of Steps"=w966:i32, "App Config.Stagger Time (ms)"=w950:i32, "App Config.Cycles Completed"=w963:u32, "App Config.PWM Freq (Hz)"=w970:dbl, "App Config.Controller Type:"=w956:T5, "Restarts Cluster"=w961:T4, "Stagger Counter"=w953:i32, "Last CMDs"=w960:dbl[], "App Config.Pumps Present"=w957:u32, "New Step"=w952:bool, "Step Start Time"=w951:dbl)
        n368 = control-ref of="CAN CMD"() -> (w955:refnum<vi>)
        n369 = call "Run Step.vi"("CAN Cmd Ref"=w955, "FPGA Ref"=w947, "Stagger Time (ms)"=w950, "Cycles Completed in"=w963, "PWM Freq (Hz)"=w970, "Controller Type:"=w956, "# of Steps"=w966, "Restarts Cluster"=w961, "VoltCtrlRef"=w946, "Stagger Counter"=w953, "Current Step in"=w965, "Last CMDs"=w960, "Profile"=w971, "Pumps Present"=w957) -> ("PS Cmd"=w948:dbl, "Ignition Relays"=w943:T2, "Manual CMDs"=w945:dbl[], "Current Step out"=w964:i32, "Press Cmd"=w949:dbl, "Cycles Completed out"=w962:u32, "Step Time"=w967:dbl, "Power Relays"=w944:T2, "Restarts Cluster OUT"=w959:T4)  [unwired: 5 in]
        n370 = local write "Power Supply Cmd (V):"(w948) -> ()
        n371 = local write "PressureCMD"(w949) -> ()
        n372 = local write "Manual\nCMD"(w945) -> ()
        n373 = case shown="True" w952 {
          tunnel: [w972 w973] -> w954
          tunnel: w951 -> [w972 _]
          tunnel: w945 -> [_ _]
          frame False {
          }
          frame True {
            n374 = Get Date/Time In Seconds() -> (seconds since 1Jan1904=w974:timestamp)
            n375 = To Double Precision Float(number=w974) -> (double precision float=w973:dbl)
          }
        }
        n376 = local write "Power Relay"(w944) -> ()
        n377 = local write "Ignition Relay"(w943) -> ()
        n378 = Bundle By Name(cluster=w969, "PS CMD"=w948, "Press CMD"=w949, "Current Step"=w964, "App Config.Cycles Completed"=w962, "Step Time"=w967, "Restarts Cluster"=w959, "Last CMDs"=w945, "Step Start Time"=w954, "Power Relay"=w944, "Ignition Relay"=w943) -> (w968:T17)
      }
      frame "Update Screen" {
        w1005 = FALSE ("Update Screen")
        w1046 = bool[] [FALSE, FALSE, FALSE, FALSE, FALSE, FALSE] ("pb.Resets")
        # "there used to be a case structure\nover updating the main bundle it was off\nmaking sure that all elapsed times were\ngreater than or equal to the initial times\nthis should mean that it was just watching\nfor a rollover case but I feel that is probably\nunnecessary with a double"
        n379 = Unbundle By Name(w1047) -> ("App Config.Stagger Time (ms)"=w1017:i32, "Update Profile"=w1018:bool, "Profile"=w1019:string[][], "App Config.Current Profile"=w985:string, "App Config.Location"=→"Location:":string, "App Config.CA Number"=w984:string, "App Config.Cycles Completed"=→"Cycles Completed:":u32, "Current Step"=→"Current Step:":i32, "Step Time Left"=→"Step Time Left:":dbl, "App Config.Controller Type:"=w1020:T5, "Restarts Cluster"=w1041:T4, "Restarts Limits"=w1040:T3, "Run Profile"=w982:bool, "Actual Starts"=w1039:T15, "Cog Limits:"=w1015:i32[], "Cog Events"=w1014:i32[], "CogCounters"=w1010:i32[], "Manual CMDs"=w983:dbl[], "Stop Cmd"=w1013:dbl, "App Config.Pumps Present"=w1012:u32, "Tank Data"=w1000:dbl[], "Intitial Times"=w999:dbl[], "App Config.Tank 1 Fuel"=w1004:string, "App Config.Tank 2 Fuel"=w1003:string, "App Config.Serial Numbers"=w1002:T31, "Controller.Invert PWM"=w981:bool, "PS CMD"=w978:dbl, "Press CMD"=w979:dbl)  [unwired: 1 out]
        n380 = disable-structure shown="Enabled" {
          disable-tunnel: w980 -> [w1049 w1057]
          disable-tunnel: [w1048 w1056] -> w1024
          disable-tunnel: w981 -> [_ w1055]
          disable-tunnel: w979 -> [_ w1052]
          disable-tunnel: w978 -> [_ w1053]
          frame Disabled {
            n381 = xnode "Read/Write Control"("FPGA VI Reference In"=w1049) -> ("Detected Starts"=w1048)  [unwired: 1 in, 2 out]
          }
          frame Enabled {
            n382 = Not Equal To 0?(x=w1053) -> (x != 0?=w1054:bool)
            n383 = Divide(x=w1052, y=160.0) -> (x/y=w1051:dbl)
            n384 = xnode "Read/Write Control"("FPGA VI Reference In"=w1057, "InvertPWM"=w1055, "PS Control"=w1054, "AO0"=w1051) -> ("Actual Pump Starts"=w1056:u32[])  [unwired: 1 in, 2 out]
          }
        }
        n385 = local write "Stagger Time (ms):"(w1017) -> ()
        n386 = local write "Profile Name:"(w985) -> ()
        n387 = local write "CA Number:"(w984) -> ()
        n388 = local write "Controller Type:"(w1020) -> ()
        n389 = local write "Tank 1 Fuel Type"(w1004) -> ()
        n390 = local write "Tank 2 Fuel Type"(w1003) -> ()
        n391 = local write "Serial Numbers"(w1002) -> ()
        n392 = Equal?(x=w983, y=w1013) -> (x = y?=w1029:bool[])
        n393 = feedback-in #1(w1029) -> ()
        n394 = feedback #1(w1029) -> (w1030:bool[])
        n395 = Less?(x=w1029, y=w1030) -> (x < y?=w1009:bool[])
        n396 = Number To Boolean Array(number=w1012) -> (Boolean array=w1001:bool[])
        n397 = disable-structure shown="Disabled" {
          disable-tunnel: w985 -> [w1060 _]
          disable-tunnel: w982 -> [w1059 _]
          frame Disabled {
            n398 = Select(t="running", s=w1059, f="idle") -> (s? t:f=w1063:string)
            n399 = Bundle By Name(cluster=T28 {"number"=0, "building"="", "room"="", "ipAddress"="", "profileName"="", "caNumber"="", "ctrlType"="", "mode"="", "channels"=[], "pumps"=[]} ("tank"), "profileName"=w1060, "mode"=w1063) -> (w1064:T28)
            n400 = call "JSON Global.vi"("Write (F)"=TRUE, "JSON In"=w1064) -> ()  [unwired: 9 in, 1 out]
          }
          frame Enabled {
          }
        }
        n401 = call "Signal Breakout.vi"("Pumps Enabled"=w1001, "Tank Data"=w1000, "Intitial Times"=w999) -> ("Pump Data"=w988:T20, "Tank Data"=w987:T36, "Elapsed Time:"=w975:dbl[])  [unwired: 10 in]
        n402 = call "Calculate Restarts.vi"("Restarts Cluster"=w1041, "Restarts Limits"=w1040, "Run Profile"=w982, "Actual Starts"=w1039, "Actual Pump Starts (FPGA)"=w1024) -> ("Restarts Cluster OUT"=w1016:T4, "Restarts Alarm"=w1026:bool, "Restarts Limits OUT"=w1043:T3, "Actual Starts OUT"=w1042:T15)  [unwired: 7 in]
        "Restarts Cluster" <- w1016
        n403 = case shown="True" w1018 {
          tunnel: w1019 -> [_ w1072]
          frame False {
          }
          frame True {
            n404 = local write "Profile:"(w1072) -> ()
          }
        }
        n405 = local write "Restarts Limits"(w1043) -> ()
        n406 = Unbundle(w988) -> ("Voltages"=→"Voltages":dbl[], "PumpCurrent"=→"PumpCurrent":dbl[], "Speed"=w996:dbl[], "ControllerCurrent"=→"ControllerCurrent":dbl[], "Pressure"=→"Pressure":dbl[], "Flow"=w993:dbl[], "Elapsed Time:"=→"Elapsed Time:":dbl[])
        "Speed" <- w996
        "Flow" <- w993
        n407 = Unbundle(w987) -> ("PS Actual (V):"=→"PS Actual (V):":dbl, "Temp1"=→"Temp1":dbl, "Temp2"=→"Temp2":dbl)
        n408 = disable-structure shown="Disabled" {
          disable-tunnel: w975 -> [w1058 _]
          frame Disabled {
            n409 = call "Elapsed Time Global.vi"("Ticks IN"=w1058) -> ()  [unwired: 10 in, 1 out]
          }
          frame Enabled {
          }
        }
        n410 = Boolean To (0,1)(Boolean=w1001) -> (0, 1=w1031:i16[])
        n411 = To Double Precision Float(number=w1031) -> (double precision float=w1011:dbl[])
        n412 = call "Pump Manual Commands.vi"("Write (F)"=TRUE, "Pumps Enabled IN"=w1001, "Manual CMDs IN"=w983) -> ()  [unwired: 7 in, 2 out]
        n413 = call "Cog Detector.vi"("Cog Limits:"=w1015, "Cogs IN"=w1014, "Counters IN"=w1010, "Started"=w1009, "Pump Present"=w1001, "Flow"=w993, "Run Profile"=w982) -> ("Cogs OUT"=w1027:i32[], "Cog Alarm"=w1025:bool, "Counters OUT"=w1028:i32[])  [unwired: 6 in]
        "Cog Events:" <- w1027
        n414 = Array To Cluster(array=w1001) -> (cluster=w1008:T33)
        n415 = case shown="True" w982 {
          tunnel: [w1067 w1069] -> w1045
          tunnel: w1044 -> [w1067 w1068]
          frame False {
          }
          frame True {
            n416 = Insert Into Array(array=w1068, index=0, new element=Sequence_States."Save Status") -> (w1069:T14[])
          }
        }
        n417 = Add Array Elements(numeric array=w996) -> (sum=w1037:dbl)
        n418 = Add Array Elements(numeric array=w1011) -> (sum=w1035:dbl)
        n419 = local write "Pumps Present"(w1008) -> ()
        n420 = Equal To 0?(x=w1035) -> (x = 0?=w1036:bool)
        n421 = Select(t=1.0, s=w1036, f=w1035) -> (s? t:f=w1033:dbl)
        n422 = Divide(x=w1037, y=w1033) -> (x/y=→"Ave. Speed":dbl)
        n423 = Or(x=w1026, y=w1025) -> (x .or. y?=w976:bool)
        n424 = Get Date/Time In Seconds() -> (seconds since 1Jan1904=w1007:timestamp)
        n425 = To Double Precision Float(number=w1007) -> (double precision float=w1006:dbl)
        n426 = Bundle By Name(cluster=w1047, "Last Update"=w1006, "Update Screen"=w1005, "Update Profile"=w1005, "Restarts Cluster"=w1016, "Alarm"=w976, "Restart Alarm"=w976, "Actual Starts"=w1042, "Pumps Present"=w1008, "Elapsed Times"=w975, "Cog Events"=w1027, "CogCounters"=w1028) -> (w977:T17)
        n427 = local write "pb.Resets"(w1046) -> ()
        n428 = local write "pb.Sets"(w1046) -> ()
      }
      frame "Stop Profile" {
        w1082 = T2 {"Pump 1"=FALSE, "Pump 2"=FALSE, "Pump 3"=FALSE, "Pump 4"=FALSE, "Pump 5"=FALSE, "Pump 6"=FALSE} ("Power Relay")
        w1083 = FALSE ("Run Profile")
        n429 = Unbundle By Name(w1079) -> ("App Config.Controller Type:"=w1077:T5, "App Config.PWM Freq (Hz)"=w1078:dbl)
        n430 = Divide(x=400000.0 ("y"), y=w1078) -> (x/y=w1081:dbl)
        n431 = case shown="\"Kuhnke\"" w1077 {
          tunnel: w1081 -> [_ w1096 w1100 w1104 w1108]
          tunnel: [0 w1095 w1099 w1103 w1107] -> w1073
          tunnel: [0.0 w1093 w1097 w1101 w1105] -> w1076
          frame Default {
          }
          frame "Kuhnke" {
            w1093 = 10.0 ("y")
            n432 = Multiply(x=w1096, y=w1093) -> (x*y=w1094:dbl)
            n433 = To Long Integer(number=w1094) -> (32bit integer=w1095:i32)
          }
          frame "PSA" {
            w1097 = 5.0 ("y")
            n434 = Multiply(x=w1100, y=w1097) -> (x*y=w1098:dbl)
            n435 = To Long Integer(number=w1098) -> (32bit integer=w1099:i32)
          }
          frame "8 Comm Hella", "10 Comm Hella" {
            w1101 = 80.0 ("y")
            n436 = Multiply(x=w1104, y=w1101) -> (x*y=w1102:dbl)
            n437 = To Long Integer(number=w1102) -> (32bit integer=w1103:i32)
          }
          frame "8 Comm Omron", "10 Comm Omron" {
            w1105 = 75.0 ("y")
            n438 = Multiply(x=w1108, y=w1105) -> (x*y=w1106:dbl)
            n439 = To Long Integer(number=w1106) -> (32bit integer=w1107:i32)
          }
        }
        n440 = Initialize Array(w1076, 6 ("dimension size")) -> (w1074:dbl[])
        n441 = disable-structure shown="Enabled" {
          disable-tunnel: w1088 -> [w1111 w1115]
          disable-tunnel: w1073 -> [_ w1114]
          frame Disabled {
            w1109 = fxp<+/-,20,5> 0.0 ("AO0")
            w1110 = 0 ("Duty (Ticks) 1")
            # "This was disabled before I started"
            # "Solenoid"
            n442 = xnode "Read/Write Control"("FPGA VI Reference In"=w1111, "Duty (Ticks) 1"=w1110, "Duty (Ticks) 2"=w1110, "Duty (Ticks) 3"=w1110, "Duty (Ticks) 4"=w1110, "Duty (Ticks) 5"=w1110, "Duty (Ticks) 6"=w1110, "AO0"=w1109, "AO1"=w1109) -> ()  [unwired: 1 in, 2 out]
          }
          frame Enabled {
            n443 = xnode "Read/Write Control"("FPGA VI Reference In"=w1115, "Duty (Ticks) 1"=w1114, "Duty (Ticks) 2"=w1114, "Duty (Ticks) 3"=w1114, "Duty (Ticks) 4"=w1114, "Duty (Ticks) 5"=w1114, "Duty (Ticks) 6"=w1114, "AO0"=fxp<+/-,20,5> 0.0, "PS Control"=FALSE) -> ()  [unwired: 1 in, 2 out]
          }
        }
        n444 = local write "pb.Run Profile"(w1083) -> ()
        n445 = Bundle By Name(cluster=w1079, "Run Profile"=w1083, "Manual CMDs"=w1074, "Last CMDs"=w1074, "Power Relay"=w1082, "Ignition Relay"=w1082) -> (w1090:T17)
        n446 = local write "Power Relay"(w1082) -> ()
        n447 = local write "Ignition Relay"(w1082) -> ()
        n448 = local write "Manual\nCMD"(w1074) -> ()
        n449 = property on="Main Tab" class="TabCtl (strict)"("DisabledEnum"=T27."Enabled" ("Disabled")) -> ()  [unwired: 2 in, 2 out]
        n450 = Insert Into Array(array=w1086, index=0, new element=Sequence_States."Set Manual CMD") -> (w1084:T14[])
      }
      frame "Save As" {
        n451 = property on="Save As Tab" class="TabCtl (strict)"("Visible"=TRUE) -> (error out=w1116:errorcluster)  [unwired: 2 in, 1 out]
        n452 = while {
          tunnel: ["pb.Save As OK"] -> w1123
          tunnel: w1116 -> [_]
          stop <- w1125 stop-if-true
          n453 = Wait (ms)(milliseconds to wait=u32 10) -> ()  [unwired: 1 out]
          n454 = Or(x="pb.Save As OK", y="pb.Save As Cancel") -> (x .or. y?=w1125:bool)
        }
        n455 = Unbundle By Name(w1120) -> ("App Config.Profiles Path"=w1122:path, "Profile"=w1118:string[][])
        n456 = case shown="True" w1123 {
          tunnel: w1122 -> [_ w1133]
          tunnel: [w1128 w1130] -> w1121
          tunnel: w1120 -> [w1129 w1135]
          tunnel: [w1129 w1134] -> w1119
          tunnel: w1118 -> [_ w1132]
          frame False {
            w1128 = T14[] [enum."Enable Background"] items=["Main", "Init Files", "Init", "Save As", "Start Profile", "Check Step Time", "Alarm", "Run Step", "Stop Profile", "Cycle Reset", "Time Reset", "Time Reset All", "Time Set", "Tare CTs", "Save Profile", "Open Profile", "Get Profiles", "Update Screen", "Save Status", "Set Manual CMD", "Reset Restarts", "Reset Total Restarts", "Reset Cogs", "Disable Background", "Enable Background", "Get/Release Control", "Init AKLH", "Save AKLH", "Log Fuel Change", "Update Data Stream", "Init TenHz", "Read TenHz", "Remote Timer Reset", "Record Frequency Change", "Controller Change", "Get Alarms", "Init Alarms", "Save Alarms"]
          }
          frame True {
            w1130 = T14[] [enum."Enable Background", enum."Get Profiles"] items=["Main", "Init Files", "Init", "Save As", "Start Profile", "Check Step Time", "Alarm", "Run Step", "Stop Profile", "Cycle Reset", "Time Reset", "Time Reset All", "Time Set", "Tare CTs", "Save Profile", "Open Profile", "Get Profiles", "Update Screen", "Save Status", "Set Manual CMD", "Reset Restarts", "Reset Total Restarts", "Reset Cogs", "Disable Background", "Enable Background", "Get/Release Control", "Init AKLH", "Save AKLH", "Log Fuel Change", "Update Data Stream", "Init TenHz", "Read TenHz", "Remote Timer Reset", "Record Frequency Change", "Controller Change", "Get Alarms", "Init Alarms", "Save Alarms"]
            n457 = call "Save Profile.vi"("Profile"=w1132, "Current Profile"="New Profile Name:", "Profiles Path"=w1133) -> ()  [unwired: 8 in, 1 out]
            n458 = Bundle By Name(cluster=w1135, "App Config.Current Profile"="New Profile Name:") -> (w1134:T17)
          }
        }
      }
      frame "Save Status" {
        # "Was getting stuck in a loop where I had not set my frequency so had to\nmake sure I was not recording on startup, probably could remove this now"
        n459 = Unbundle By Name(w1140) -> ("App Config"=w1143:T16, "Restarts Cluster.CMD Starts:"=w1151:i32[], "Actual Starts.Actual Pump Starts"=w1150:i32[], "Restarts Limits.High Limits:"=w1149:i32[], "Restarts Limits.Low Limits:"=w1148:i32[], "Restarts Cluster.Total CMD:"=w1147:i32[], "Actual Starts.Tot Act Starts"=w1146:i32[], "Elapsed Times"=w1139:dbl[], "CT Offsets"=w1159:fxp<+/-,26,7>[], "Cog Events"=w1145:i32[], "Cog Limits:"=w1144:i32[])
        n460 = Bundle By Name(cluster=w1143, "Record TenHz"=FALSE) -> (w1142:T16)
        n461 = call <vilib>:"Open Config Data.vi"("create file if necessary (T)"=TRUE, "configuration file path"=path "c:/App Config.ini") -> ("error out"=w1171:errorcluster, "refnum"=w1175:T35)  [unwired: 7 in, 1 out]
        n462 = Build Array(w1151, w1150, w1149, w1148, w1147, w1146, w1145, w1144) -> (w1169:i32[][])
        n463 = To Double Precision Float(number=w1159) -> (double precision float=w1158:dbl[])
        n464 = call "Read Write App Config.vi"("Write (F)"=TRUE, "Error IN"=w1171, "App Config IN"=w1142, "Refnum in"=w1175) -> ("Error OUT"=w1173:errorcluster, "Refnum out"=w1174:T35)  [unwired: 5 in, 1 out]
        n465 = Array To Spreadsheet String(delimiter (Tab)=",", array=w1169, 3:"%d" ("format string")) -> (spreadsheet string=w1166:string)
        n466 = Array To Spreadsheet String(delimiter (Tab)=",", array=w1139, 3:"%.2f" ("format string")) -> ()  [unwired: 1 out]
        n467 = Array To Spreadsheet String(delimiter (Tab)=",", array=w1158, 3:"%.2f" ("format string")) -> (spreadsheet string=w1156:string)
        n468 = call <vilib>:"Close Config Data.vi"("error in (no error)"=w1173, "refnum"=w1174) -> ()  [unwired: 8 in, 2 out]
        n469 = Write to Text File(file (use dialog)=path "c:/Restarts", text=w1166) -> (refnum out=w1155:refnum<file>, error out=w1154:errorcluster)  [unwired: 2 in, 1 out]
        n470 = Write to Text File(file (use dialog)=path "c:/CT Offsets", text=w1156) -> (refnum out=w1153:refnum<file>, error out=w1152:errorcluster)  [unwired: 2 in, 1 out]
        n471 = Array Size(array=w1139) -> (size(s)=w1138:i32)
        n472 = Close File(refnum=w1155, error in=w1154) -> ()  [unwired: 2 out]
        n473 = Close File(refnum=w1153, error in=w1152) -> ()  [unwired: 2 out]
        n474 = Equal?(x=w1138, y=6) -> (x = y?=w1136:bool)
        n475 = case shown="True" w1136 {
          tunnel: w1139 -> [_ w1177]
          frame False {
          }
          frame True {
            n476 = Write to Binary File(file (use dialog)=path "c:/ElapsedTimes", data=w1177) -> (refnum out=w1179:refnum<file>, error out=w1178:errorcluster)  [unwired: 4 in, 1 out]
            n477 = Close File(refnum=w1179, error in=w1178) -> ()  [unwired: 2 out]
          }
        }
      }
      frame "Disable Background" {
        w1181 = T27."Disabled and Grayed Out" ("Disabled")
        n478 = property on="Main Tab" class="TabCtl (strict)"("DisabledEnum"=w1181) -> ()  [unwired: 2 in, 2 out]
        n479 = property on="pb.Stop Profile" class="Bool"("DisabledEnum"=w1181) -> ()  [unwired: 2 in, 2 out]
        n480 = property on="Restarts Tab" class="TabCtl (strict)"("DisabledEnum"=w1181) -> ()  [unwired: 2 in, 2 out]
        n481 = property on="Monitoring Tab" class="TabCtl (strict)"("DisabledEnum"=w1181) -> ()  [unwired: 2 in, 2 out]
        n482 = property on="Title Tab" class="TabCtl (strict)"("DisabledEnum"=w1181) -> ()  [unwired: 2 in, 2 out]
        n483 = property on="CPU Usage:" class="DigNum (strict)"("DisabledEnum"=w1181) -> ()  [unwired: 2 in, 2 out]
      }
      frame "Enable Background" {
        w1184 = FALSE ("Visible")
        w1185 = T27."Enabled" ("Disabled")
        n484 = xnode "Read/Write Control"("FPGA VI Reference In"=w1191, "Timer Resets"=bool[] [FALSE, FALSE, FALSE, FALSE, FALSE, FALSE] ("array")) -> ()  [unwired: 1 in, 2 out]
        n485 = property on="Save As Tab" class="TabCtl (strict)"("Visible"=w1184) -> ()  [unwired: 2 in, 2 out]
        n486 = property on="Reset Tab" class="TabCtl (strict)"("Visible"=w1184) -> ()  [unwired: 2 in, 2 out]
        n487 = property on="Set Time Tab" class="TabCtl (strict)"("Visible"=w1184) -> ()  [unwired: 2 in, 2 out]
        n488 = property on="Alarm Tab" class="TabCtl (strict)"("Visible"=w1184) -> ()  [unwired: 2 in, 2 out]
        n489 = property on="Main Tab" class="TabCtl (strict)"("DisabledEnum"=w1185) -> ()  [unwired: 2 in, 2 out]
        n490 = property on="pb.Stop Profile" class="Bool"("DisabledEnum"=w1185) -> ()  [unwired: 2 in, 2 out]
        n491 = property on="Restarts Tab" class="TabCtl (strict)"("DisabledEnum"=w1185) -> ()  [unwired: 2 in, 2 out]
        n492 = property on="Monitoring Tab" class="TabCtl (strict)"("DisabledEnum"=w1185) -> ()  [unwired: 2 in, 2 out]
        n493 = property on="Title Tab" class="TabCtl (strict)"("DisabledEnum"=w1185) -> ()  [unwired: 2 in, 2 out]
        n494 = property on="CPU Usage:" class="DigNum (strict)"("DisabledEnum"=w1185) -> ()  [unwired: 2 in, 2 out]
        n495 = property on="Alarm Tab" class="TabCtl (strict)"("DisabledEnum"=w1185) -> ()  [unwired: 2 in, 2 out]
        n496 = Insert Into Array(array=w1189, index=0, new element=Sequence_States."Update Screen") -> (w1188:T14[])
      }
      frame "Cycle Reset".."Time Reset All", "Reset Restarts".."Reset Cogs" {
        w1195 = T14[] [enum."Enable Background"] items=["Main", "Init Files", "Init", "Save As", "Start Profile", "Check Step Time", "Alarm", "Run Step", "Stop Profile", "Cycle Reset", "Time Reset", "Time Reset All", "Time Set", "Tare CTs", "Save Profile", "Open Profile", "Get Profiles", "Update Screen", "Save Status", "Set Manual CMD", "Reset Restarts", "Reset Total Restarts", "Reset Cogs", "Disable Background", "Enable Background", "Get/Release Control", "Init AKLH", "Save AKLH", "Log Fuel Change", "Update Data Stream", "Init TenHz", "Read TenHz", "Remote Timer Reset", "Record Frequency Change", "Controller Change", "Get Alarms", "Init Alarms", "Save Alarms"]
        n497 = property on="Reset Tab" class="TabCtl (strict)"("Visible"=TRUE) -> (error out=w1196:errorcluster)  [unwired: 2 in, 1 out]
        n498 = while {
          tunnel: ["pb.Reset OK"] -> w1203
          tunnel: w1196 -> [_]
          stop <- w1206 stop-if-true
          n499 = Wait (ms)(milliseconds to wait=u32 10) -> ()  [unwired: 1 out]
          n500 = Or(x="pb.Reset Cancel", y="pb.Reset OK") -> (x .or. y?=w1206:bool)
        }
        n501 = Unbundle By Name(w1194) -> ("pb.Resets"=w1202:bool[], "Intitial Times"=w1199:dbl[])
        n502 = Search 1D Array(1D array=w1202, element=TRUE) -> (index of element=w1200:i32)  [unwired: 1 in]
        n503 = case shown="True" w1203 {
          tunnel: [w1209 w1216] -> w1204
          tunnel: w1194 -> [w1209 w1215]
          tunnel: w1200 -> [_ w1214]
          tunnel: w1199 -> [_ w1213]
          tunnel: w1198 -> [_ w1212]
          tunnel: w1194 -> [_ w1211]
          tunnel: w1193 -> [_ w1210]
          frame False {
          }
          frame True {
            n504 = case shown="\"Reset Restarts\"" w1210 {
              tunnel: w1215 -> [w1219 w1231 w1238 w1247 w1262 w1271]
              tunnel: [w1218 w1230 w1237 w1246 w1261 w1270] -> w1216
              tunnel: w1214 -> [_ w1226 _ _ _ _]
              tunnel: w1213 -> [_ w1229 _ _ _ _]
              tunnel: w1212 -> [_ w1224 w1236 w1245 w1260 _]
              tunnel: w1211 -> [_ _ _ w1243 w1258 _]
              frame "Cycle Reset", Default {
                n505 = Bundle By Name(cluster=w1219, "App Config.Cycles Completed"=u32 0) -> (w1218:T17)
              }
              frame "Time Reset" {
                n506 = Replace Array Subset(array=w1229, new element=0.0 ("new element/subarray"), index=w1226) -> (w1220:dbl[])
                n507 = Replace Array Subset(array=bool[] [FALSE, FALSE, FALSE, FALSE, FALSE, FALSE], new element=TRUE ("new element/subarray"), index=w1226) -> (w1227:bool[])
                n508 = xnode "Read/Write Control"("FPGA VI Reference In"=w1224, "Timer Resets"=w1227) -> ()  [unwired: 1 in, 2 out]
                n509 = Bundle By Name(cluster=w1231, "Intitial Times"=w1220) -> (w1230:T17)
                n510 = call "Elapsed Time Global.vi"("Write (F)"=TRUE, "Tick Divider"=1.0, "Initial Times IN"=w1220) -> ()  [unwired: 8 in, 1 out]
              }
              frame "Time Reset All" {
                w1232 = dbl[] [0.0, 0.0, 0.0, 0.0, 0.0, 0.0] ("Intitial Times")
                n511 = xnode "Read/Write Control"("FPGA VI Reference In"=w1236, "Timer Resets"=bool[] [TRUE, TRUE, TRUE, TRUE, TRUE, TRUE] ("array")) -> ()  [unwired: 1 in, 2 out]
                n512 = Bundle By Name(cluster=w1238, "Intitial Times"=w1232) -> (w1237:T17)
                n513 = call "Elapsed Time Global.vi"("Write (F)"=TRUE, "Tick Divider"=1.0, "Initial Times IN"=w1232) -> ()  [unwired: 8 in, 1 out]
              }
              frame "Reset Restarts" {
                w1244 = i32[] [0, 0, 0, 0, 0, 0] ("CMD Starts")
                n514 = disable-structure shown="Enabled" {
                  disable-tunnel: w1245 -> [w1250 w1253]
                  disable-tunnel: TRUE ("Reset") -> [w1249 w1251]
                  disable-tunnel: [w1248 w1252] -> w1239
                  frame Disabled {
                    n515 = xnode "Read/Write Control"("FPGA VI Reference In"=w1250, "Reset Starts"=w1249) -> ("Detected Starts"=w1248)  [unwired: 1 in, 2 out]
                  }
                  frame Enabled {
                    n516 = xnode "Read/Write Control"("FPGA VI Reference In"=w1253, "Reset"=w1251) -> ("Actual Pump Starts"=w1252:u32[])  [unwired: 1 in, 2 out]
                  }
                }
                n517 = Unbundle By Name(w1243) -> ("Actual Starts.Tot Init Act Starts"=w1240:i32[])
                n518 = Add(x=w1240, y=w1239) -> (x+y=w1242:u32[])
                n519 = Bundle By Name(cluster=w1247, "Restarts Cluster.CMD Starts:"=w1244, "Actual Starts.Actual Pump Starts"=w1244, "Actual Starts.Initial Actual Starts"=w1244, "Actual Starts.Tot Init Act Starts"=w1242) -> (w1246:T17)
              }
              frame "Reset Total Restarts" {
                w1259 = i32[] [0, 0, 0, 0, 0, 0] ("CMD Starts")
                n520 = Unbundle By Name(w1258) -> ("Actual Starts.Initial Actual Starts"=w1254:i32[])
                n521 = disable-structure shown="Enabled" {
                  disable-tunnel: w1260 -> [w1265 w1268]
                  disable-tunnel: TRUE ("Reset") -> [w1264 w1267]
                  disable-tunnel: [w1263 w1266] -> w1255
                  frame Disabled {
                    n522 = xnode "Read/Write Control"("FPGA VI Reference In"=w1265, "Reset Starts"=w1264) -> ("Detected Starts"=w1263)  [unwired: 1 in, 2 out]
                  }
                  frame Enabled {
                    n523 = xnode "Read/Write Control"("FPGA VI Reference In"=w1268, "Reset"=w1267) -> ("Actual Pump Starts"=w1266:u32[])  [unwired: 1 in, 2 out]
                  }
                }
                n524 = Add(x=w1254, y=w1255) -> (x+y=w1257:u32[])
                n525 = Bundle By Name(cluster=w1262, "Restarts Cluster.Total CMD:"=w1259, "Actual Starts.Tot Act Starts"=w1259, "Actual Starts.Tot Init Act Starts"=w1259, "Actual Starts.Initial Actual Starts"=w1257) -> (w1261:T17)
              }
              frame "Reset Cogs" {
                n526 = Bundle By Name(cluster=w1271, "Cog Events"=i32[] [0, 0, 0, 0, 0, 0]) -> (w1270:T17)
              }
            }
          }
        }
      }
      frame "Alarm" {
        w1289 = T14[] [enum."Enable Background"] items=["Main", "Init Files", "Init", "Save As", "Start Profile", "Check Step Time", "Alarm", "Run Step", "Stop Profile", "Cycle Reset", "Time Reset", "Time Reset All", "Time Set", "Tare CTs", "Save Profile", "Open Profile", "Get Profiles", "Update Screen", "Save Status", "Set Manual CMD", "Reset Restarts", "Reset Total Restarts", "Reset Cogs", "Disable Background", "Enable Background", "Get/Release Control", "Init AKLH", "Save AKLH", "Log Fuel Change", "Update Data Stream", "Init TenHz", "Read TenHz", "Remote Timer Reset", "Record Frequency Change", "Controller Change", "Get Alarms", "Init Alarms", "Save Alarms"]
        n527 = Unbundle By Name(w1274) -> ("Alarm Message"=w1285:string, "Restart Alarm"=w1284:bool, "App Config.Location"=w1277:string, "Restarts Cluster.CMD Starts:"=w1278:i32[], "Restarts Cluster.Restarts:"=w1279:i32[], "Restarts Limits.High Limits:"=w1280:i32[], "Restarts Limits.Low Limits:"=w1281:i32[], "Cog Events"=w1282:i32[], "Cog Limits:"=w1283:i32[], "App Config.Inform"=w1286:string)
        n528 = case shown="True" w1284 {
          tunnel: w1277 -> [w1292 w1303]
          tunnel: w1278 -> [_ w1302]
          tunnel: w1279 -> [_ w1301]
          tunnel: w1280 -> [_ w1300]
          tunnel: w1281 -> [_ w1299]
          tunnel: w1282 -> [_ w1298]
          tunnel: w1283 -> [_ w1297]
          tunnel: [w1293 "A pump event has occured.  Either a pump has had too many restarts, is cogging, or a fuse/breaker is tripped.  The test has been terminated.  Reset the restarts monitor in order to start the test again.  You may want to log the restarts before you reset!" ("Alarm Message")] -> w1276
          tunnel: w1285 -> [w1293 _]
          tunnel: [w1290 w1295] -> w1287
          tunnel: [w1293 w1294] -> w1288
          frame False {
            n529 = Concatenate Strings(w1292, " ALARM!" ("string")) -> (w1290:string)
          }
          frame True {
            n530 = call "Restart Alarm Message.vi"("Location"=w1303, "CMD Starts:"=w1302, "Restarts:"=w1301, "High Limits:"=w1300, "Low Limits:"=w1299, "Cog Events"=w1298, "Cog Limits:"=w1297) -> ("Subject:"=w1295:string, "Message:"=w1294:string)  [unwired: 11 in]
          }
        }
        n531 = call "Email to Handler.vi"("Email Handler IP"="34", "Message:"=w1288, "Subject:"=w1287, "To:"=w1286) -> ()  [unwired: 8 in]
        n532 = while {
          tunnel: w1276 -> [w1304]
          stop <- "pb.Alarm OK" stop-if-true
          n533 = flat-sequence {
            tunnel: w1304 -> [w1307]
            frame #0 {
              "Alarm Message" <- w1307
            }
            frame #1 {
              n534 = property on="Alarm Tab" class="TabCtl (strict)"("Visible"=TRUE) -> ()  [unwired: 2 in, 2 out]
            }
          }
          n535 = Wait (ms)(milliseconds to wait=u32 20) -> ()  [unwired: 1 out]
        }
        n536 = Bundle By Name(cluster=w1274, "Restart Alarm"=FALSE) -> (w1273:T17)
      }
      frame "Time Set" {
        w1309 = T14[] [enum."Enable Background", enum."Save Status"] items=["Main", "Init Files", "Init", "Save As", "Start Profile", "Check Step Time", "Alarm", "Run Step", "Stop Profile", "Cycle Reset", "Time Reset", "Time Reset All", "Time Set", "Tare CTs", "Save Profile", "Open Profile", "Get Profiles", "Update Screen", "Save Status", "Set Manual CMD", "Reset Restarts", "Reset Total Restarts", "Reset Cogs", "Disable Background", "Enable Background", "Get/Release Control", "Init AKLH", "Save AKLH", "Log Fuel Change", "Update Data Stream", "Init TenHz", "Read TenHz", "Remote Timer Reset", "Record Frequency Change", "Controller Change", "Get Alarms", "Init Alarms", "Save Alarms"]
        n537 = Unbundle By Name(w1319) -> ("pb.Sets"=w1318:bool[], "Intitial Times"=w1313:dbl[], "Elapsed Times"=w1316:dbl[])
        n538 = Search 1D Array(1D array=w1318, element=TRUE) -> (index of element=w1315:i32)  [unwired: 1 in]
        n539 = Index Array(array=w1316, index=w1315) -> (element=w1314:dbl)
        n540 = local write "New Time"(w1314) -> ()
        n541 = property on="Set Time Tab" class="TabCtl (strict)"("Visible"=TRUE) -> (error out=w1310:errorcluster)  [unwired: 2 in, 1 out]
        n542 = while {
          tunnel: ["pb.Set Time OK"] -> w1321
          tunnel: w1314 -> [_]
          tunnel: w1310 -> [_]
          stop <- w1324 stop-if-true
          n543 = Wait (ms)(milliseconds to wait=u32 10) -> ()  [unwired: 1 out]
          n544 = Or(x="pb.Set Time Cancel", y="pb.Set Time OK") -> (x .or. y?=w1324:bool)
        }
        n545 = case shown="True" w1321 {
          tunnel: w1319 -> [w1326 w1332]
          tunnel: [w1326 w1331] -> w1320
          tunnel: w1315 -> [_ w1328]
          tunnel: w1313 -> [_ w1330]
          tunnel: w1312 -> [_ w1329]
          frame False {
          }
          frame True {
            n546 = xnode "Read/Write Control"("FPGA VI Reference In"=w1329) -> ("FPGA VI Reference Out"=w1335:T18, "Timer Resets"=w1336:bool[])  [unwired: 1 in, 1 out]
            n547 = Replace Array Subset(array=w1330, new element="New Time", index=w1328) -> (w1337:dbl[])
            n548 = Replace Array Subset(array=w1336, new element=TRUE ("new element/subarray"), index=w1328) -> (w1334:bool[])
            n549 = Bundle By Name(cluster=w1332, "Intitial Times"=w1337) -> (w1331:T17)
            n550 = xnode "Read/Write Control"("FPGA VI Reference In"=w1335, "Timer Resets"=w1334) -> ()  [unwired: 1 in, 2 out]
          }
        }
      }
      frame "Remote Timer Reset" {
        n551 = disable-structure shown="Enabled" {
          disable-tunnel: w1338 -> [w1358 _]
          disable-tunnel: [w1348 w1368] -> w1341
          disable-tunnel: w1340 -> [w1347 w1367]
          disable-tunnel: w1338 -> [w1342 w1363]
          frame Disabled {
            # "Reset individual timer."
            n552 = Unbundle By Name(w1358) -> ("Intitial Times"=w1354:dbl[], "pb.Resets"=w1356:bool[])
            n553 = Search 1D Array(1D array=w1356, element=TRUE) -> (index of element=w1350:i32)  [unwired: 1 in]
            n554 = Replace Array Subset(array=bool[] [FALSE, FALSE, FALSE, FALSE, FALSE, FALSE] ("pb.Resets"), new element=TRUE ("new element/subarray"), index=w1350) -> (w1346:bool[])
            n555 = Replace Array Subset(array=w1354, new element=0.0 ("new element/subarray"), index=w1350) -> (w1352:dbl[])
            n556 = xnode "Read/Write Control"("FPGA VI Reference In"=w1347, "Timer Resets"=w1346) -> ("FPGA VI Reference Out"=w1344:T18)  [unwired: 1 in, 1 out]
            n557 = Bundle By Name(cluster=w1342, "pb.Resets"=bool[] [FALSE, FALSE, FALSE, FALSE, FALSE, FALSE], "Intitial Times"=w1352) -> (w1348:T17)
            n558 = flat-sequence {
              tunnel: w1344 -> [w1359]
              tunnel: [w1359] -> w1343
              frame #0 {
                n559 = Wait (ms)(milliseconds to wait=u32 20) -> ()  [unwired: 1 out]
              }
            }
            n560 = xnode "Read/Write Control"("FPGA VI Reference In"=w1343, "Timer Resets"=bool[] [FALSE, FALSE, FALSE, FALSE, FALSE, FALSE] ("pb.Resets")) -> ()  [unwired: 1 in, 2 out]
          }
          frame Enabled {
            n561 = xnode "Read/Write Control"("FPGA VI Reference In"=w1367, "Timer Resets"=bool[] [TRUE, TRUE, TRUE, TRUE, TRUE, TRUE] ("pb.Resets")) -> ("FPGA VI Reference Out"=w1365:T18)  [unwired: 1 in, 1 out]
            n562 = Bundle By Name(cluster=w1363, "Intitial Times"=dbl[] [0.0, 0.0, 0.0, 0.0, 0.0, 0.0]) -> (w1368:T17)
            n563 = flat-sequence {
              tunnel: w1365 -> [w1369]
              tunnel: [w1369] -> w1364
              frame #0 {
                n564 = Wait (ms)(milliseconds to wait=u32 20) -> ()  [unwired: 1 out]
              }
            }
            n565 = xnode "Read/Write Control"("FPGA VI Reference In"=w1364, "Timer Resets"=bool[] [FALSE, FALSE, FALSE, FALSE, FALSE, FALSE] ("pb.Resets")) -> ()  [unwired: 1 in, 2 out]
          }
        }
      }
      frame "Set Manual CMD" {
        w1398 = fxp<+/-,20,5> 0.0 ("AO0")
        n566 = Unbundle By Name(w1397) -> ("App Config.Controller Type:"=w1403:T5, "App Config.PWM Freq (Hz)"=w1404:dbl, "Manual CMDs"=w1402:dbl[], "PS CMD"=w1388:dbl, "Press CMD"=w1392:dbl, "Voltage Enable"=w1390:bool, "App Config.VoltCtrlRef"=w1375:string, "Power Relay"=w1373:T2, "Ignition Relay"=w1372:T2)
        n567 = Unbundle(w1373) -> ("Pump 1"=w1387:bool, "Pump 2"=w1386:bool, "Pump 3"=w1385:bool, "Pump 4"=w1384:bool, "Pump 5"=w1383:bool, "Pump 6"=w1382:bool)
        n568 = Unbundle(w1372) -> ("Pump 1"=w1381:bool, "Pump 2"=w1380:bool, "Pump 3"=w1379:bool, "Pump 4"=w1378:bool, "Pump 5"=w1377:bool, "Pump 6"=w1376:bool)
        n569 = Not(x=w1390) -> (.not. x?=w1374:bool)
        n570 = Divide(x=w1388, y=10.0) -> (x/y=w1396:dbl)
        n571 = Divide(x=w1392, y=165.0) -> (x/y=w1393:dbl)
        n572 = To Fixed-Point(fixed-point type=w1398, number=w1396) -> (fixed-point=w1399:fxp<+/-,20,5>)
        n573 = To Fixed-Point(fixed-point type=w1398, number=w1393) -> (fixed-point=w1400:fxp<+/-,20,5>)
        n574 = disable-structure shown="Enabled" {
          disable-tunnel: w1400 -> [w1421 w1425]
          disable-tunnel: w1399 -> [w1420 w1423]
          disable-tunnel: w1391 -> [w1419 w1426]
          disable-tunnel: [w1418 w1424] -> w1389
          disable-tunnel: w1387 -> [w1417 _]
          disable-tunnel: w1386 -> [w1416 _]
          disable-tunnel: w1385 -> [w1415 _]
          disable-tunnel: w1384 -> [w1414 _]
          disable-tunnel: w1383 -> [w1413 _]
          disable-tunnel: w1382 -> [w1412 _]
          disable-tunnel: w1381 -> [w1411 _]
          disable-tunnel: w1380 -> [w1410 _]
          disable-tunnel: w1379 -> [w1409 _]
          disable-tunnel: w1378 -> [w1408 _]
          disable-tunnel: w1377 -> [w1407 _]
          disable-tunnel: w1376 -> [w1406 _]
          disable-tunnel: w1374 -> [w1405 _]
          frame Disabled {
            n575 = xnode "Read/Write Control"("FPGA VI Reference In"=w1419, "AO3"=w1420, "AO0"=w1421, "DIO6"=w1417, "DIO7"=w1416, "DIO8"=w1415, "DIO9"=w1414, "DIO10"=w1413, "DIO11"=w1412, "DIO12"=w1411, "DIO13"=w1410, "DIO14"=w1409, "DIO15"=w1408, "DIO16"=w1407, "DIO17"=w1406, "DIO18"=w1405) -> ("error out"=w1418:errorcluster)  [unwired: 1 in, 1 out]
          }
          frame Enabled {
            n576 = Not Equal To 0?(x=w1423) -> (x != 0?=w1422:bool)
            n577 = xnode "Read/Write Control"("FPGA VI Reference In"=w1426, "PS Control"=w1422, "AO0"=w1425) -> ("error out"=w1424:errorcluster)  [unwired: 1 in, 1 out]
          }
        }
        n578 = case shown="\"Kuhnke\", \"PSA\", Default" w1403 {
          selector: w1403 -> [w1437 _]
          tunnel: w1391 -> [w1451 _]
          tunnel: w1404 -> [w1435 _]
          tunnel: w1402 -> [w1450 w1458]
          frame "Kuhnke", "PSA", Default {
            n579 = disable-structure shown="Enabled" {
              disable-tunnel: w1437 -> [w1453 _]
              disable-tunnel: [w1452 w1456] -> w1436
              disable-tunnel: w1435 -> [_ w1456]
              frame Disabled {
                n580 = case shown="\"Kuhnke\", Default" w1453 {
                  tunnel: [100.0 ("y") 150.0 ("y")] -> w1452
                  frame "Kuhnke", Default {
                  }
                  frame "PSA" {
                  }
                }
              }
              frame Enabled {
              }
            }
            n581 = Divide(x=40000000.0 ("40 MHz"), y=w1436) -> (x/y=w1442:dbl)
            n582 = Multiply(x=w1442, y=w1450) -> (x*y=w1438:dbl[])
            n583 = Divide(x=w1438, y=100.0 ("%")) -> (x/y=w1440:dbl[])
            n584 = To Long Integer(number=w1440) -> (32bit integer=w1449:i32[])
            n585 = Index Array(array=w1449) -> (element #1=w1448:i32, element #2=w1447:i32, element #3=w1446:i32, element #4=w1445:i32, element #5=w1444:i32, element #6=w1443:i32)  [unwired: 6 in]
            n586 = xnode "Read/Write Control"("FPGA VI Reference In"=w1451, "Duty (Ticks) 1"=w1448, "Duty (Ticks) 2"=w1447, "Duty (Ticks) 3"=w1446, "Duty (Ticks) 4"=w1445, "Duty (Ticks) 5"=w1444, "Duty (Ticks) 6"=w1443) -> ()  [unwired: 1 in, 2 out]
          }
          frame "Conti", "Hella CAN" {
            n587 = Index Array(array=w1458) -> (element=→"CAN CMD":dbl)  [unwired: 1 in]
          }
        }
        n588 = Empty String/Path?(string/path=w1375) -> (empty?=w1371:bool)
        n589 = case shown="False" w1371 {
          tunnel: w1389 -> [_ w1430]
          tunnel: w1388 -> [_ w1428]
          tunnel: w1375 -> [_ w1427]
          frame True {
          }
          frame False {
            n590 = shared-variable-open(w1427, w1430, 0.0) -> (w1434:refnum<k21>, w1431:errorcluster)  [unwired: 1 in]
            n591 = shared-variable-write(w1434, w1431, w1428) -> (w1433:refnum<k21>, w1432:errorcluster)
            n592 = Close Variable Connection(8:w1432, 11:w1433) -> ()  [unwired: 1 out]
          }
        }
      }
      frame "Get/Release Control" {
        n593 = Unbundle By Name(w1463) -> ("Login"=w1460:bool)
        n594 = case shown="True" w1460 {
          tunnel: [T27."Disabled" ("Disabled") T27."Enabled" ("Disabled")] -> w1462
          frame False {
          }
          frame True {
          }
        }
        n595 = local write "Main Tab"(enum32{"Main", "Data Stream", "Alarms"}."Main" ("Main Tab")) -> ()
        n596 = property on="Main Tab" class="TabCtl (strict)"("DisabledEnum"=w1462) -> ()  [unwired: 2 in, 2 out]
        n597 = property on="pb.Stop Profile" class="Bool"("DisabledEnum"=w1462) -> ()  [unwired: 2 in, 2 out]
        n598 = property on="Restarts Tab" class="TabCtl (strict)"("DisabledEnum"=w1462) -> ()  [unwired: 2 in, 2 out]
        n599 = property on="Monitoring Tab" class="TabCtl (strict)"("DisabledEnum"=w1462) -> ()  [unwired: 2 in, 2 out]
      }
      frame "Init AKLH" {
        w1476 = " " ("string")
        n600 = Unbundle By Name(w1483) -> ("AKLH Path"=w1481:path, "App Config.Location"=w1478:string, "App Config.CA Number"=w1477:string)
        n601 = Get Date/Time In Seconds() -> (seconds since 1Jan1904=w1467:timestamp)
        n602 = call "Timestamp2DayofYear.vi"("time stamp"=w1467) -> ("time string"=w1475:string)  [unwired: 14 in]
        n603 = Concatenate Strings("Continuous Monitoring " ("string"), w1478, w1476, w1477, w1476, w1475) -> (w1470:string)
        n604 = Strip Path(path=w1481) -> (stripped path=w1480:path)  [unwired: 1 out]
        n605 = Concatenate Strings(w1470, ".csv" ("string")) -> (w1471:string)
        n606 = Build Path(base path=w1480, name or relative path=w1471) -> (appended path=w1474:path)
        n607 = for {
          N: 10 -> [_]
          shift-right: [w1497] -> w1468
          shift-left: w1474 -> [w1499]
          tunnel: w1470 -> [w1494]
          tunnel: [w1492] -> w1469
          i -> [w1496]
          stop <- w1492 continue-if-true
          n608 = call <vilib>:"Check if File or Folder Exists.vi"("path"=w1499) -> ("file or folder exists?"=w1492:bool, "dup path"=w1498:path)  [unwired: 8 in, 1 out]
          n609 = Add(x=2, y=w1496) -> (x+y=w1493:i32)
          n610 = case shown="True" w1492 {
            tunnel: w1498 -> [w1505 w1507]
            tunnel: [w1500 w1507] -> w1497
            tunnel: w1494 -> [w1503 _]
            tunnel: w1493 -> [w1502 _]
            frame True {
              n611 = Strip Path(path=w1505) -> (stripped path=w1506:path)  [unwired: 1 out]
              n612 = Format Into String(format string="%s_%d.csv", w1503, w1502) -> (resulting string=w1501:string)  [unwired: 2 in, 1 out]
              n613 = Build Path(base path=w1506, name or relative path=w1501) -> (appended path=w1500:path)
            }
            frame False {
            }
          }
        }
        n614 = To Double Precision Float(number=w1467) -> (double precision float=w1466:dbl)
        n615 = case shown="False" w1469 {
          tunnel: [w1486 w1491] -> w1484
          tunnel: w1468 -> [w1486 w1488]
          frame True {
          }
          frame False {
            w1487 = string[] ["Time", "Cycles Completed", "Current Step", "PS Voltage (V)", "Tank 1 Temp (C)", "Tank 1 Fuel Type", "Position 1 Serial Number", "Position 1 Elapsed On Time", "Position 1 Controller Current (Adc)", "Position 1 Pump Current (Arms)", "Position 1 Pressure (kPa)", "Position 1 Flow (L/H)", "Position 1 Speed (RPM)", "Position 2 Serial Number", "Position 2 Elapsed On Time", "Position 2 Controller Current (Adc)", "Position 2 Pump Current (Arms)", "Position 2 Pressure (kPa)", "Position 2 Flow (L/H)", "Position 2 Speed (RPM)", "Position 3 Serial Number", "Position 3 Elapsed On Time", "Position 3 Controller Current (Adc)", "Position 3 Pump Current (Arms)", "Position 3 Pressure (kPa)", "Position 3 Flow (L/H)", "Position 3 Speed (RPM)", "Tank 2 Temp (C)", "Tank 2 Fuel Type", "Position 4 Serial Number", "Position 4 Elapsed On Time", "Position 4 Controller Current (Adc)", "Position 4 Pump Current (Arms)", "Position 4 Pressure (kPa)", "Position 4 Flow (L/H)", "Position 4 Speed (RPM)", "Position 5 Serial Number", "Position 5 Elapsed On Time", "Position 5 Controller Current (Adc)", "Position 5 Pump Current (Arms)", "Position 5 Pressure (kPa)", "Position 5 Flow (L/H)", "Position 5 Speed (RPM)", "Position 6 Serial Number", "Position 6 Elapsed On Time", "Position 6 Controller Current (Adc)", "Position 6 Pump Current (Arms)", "Position 6 Pressure (kPa)", "Position 6 Flow (L/H)", "Position 6 Speed (RPM)"]  # AKLH Header
            n616 = call-poly <vilib>:"Write To Spreadsheet File.vi"("delimiter (\\t)"="," ("delimiter (\\t)"), "append to file? (new file:F)"=TRUE, "1D data"=w1487, "file path (dialog if empty)"=w1488) -> ("new file path (Not A Path if cancelled)"=w1491:path)  [unwired: 4 in]
          }
        }
        n617 = Bundle By Name(cluster=w1483, "AKLH Path"=w1484, "AKLH Timer"=w1466) -> (w1482:T17)
      }
      frame "Save AKLH" {
        n618 = Unbundle By Name(w1522) -> ("AKLH Timer"=w1511:dbl, "AKLH Path"=w1524:path, "App Config.Cycles Completed"=w1520:u32, "Current Step"=w1519:i32, "AKLH Last Hour"=w1513:i32)
        n619 = Get Date/Time In Seconds() -> (seconds since 1Jan1904=w1508:timestamp)
        n620 = Seconds To Date/Time(time stamp (now)=w1508) -> (date time rec=w1518:T34)  [unwired: 1 in]
        n621 = Unbundle By Name(w1518) -> ("hour"=w1509:i32)
        n622 = Format Date/Time String(time format string (%c)="%H:%M", seconds (now)=w1508) -> (date/time string=w1517:string)  [unwired: 1 in]
        n623 = Less Or Equal?(x=w1513, y=w1509) -> (x <= y?=w1512:bool)
        n624 = case shown="True" w1512 {
          tunnel: w1524 -> [w1530 w1573]
          tunnel: w1520 -> [_ w1555]
          tunnel: w1519 -> [_ w1554]
          tunnel: w1517 -> [_ w1539]
          tunnel: [w1530 w1538] -> w1516
          tunnel: w1515 -> [w1528 w1537]
          tunnel: [w1527 w1537] -> w1514
          tunnel: w1511 -> [w1525 _]
          tunnel: [w1525 w1531] -> w1510
          frame False {
            w1526 = T14[] [enum."Init AKLH", enum."Save AKLH"] items=["Main", "Init Files", "Init", "Save As", "Start Profile", "Check Step Time", "Alarm", "Run Step", "Stop Profile", "Cycle Reset", "Time Reset", "Time Reset All", "Time Set", "Tare CTs", "Save Profile", "Open Profile", "Get Profiles", "Update Screen", "Save Status", "Set Manual CMD", "Reset Restarts", "Reset Total Restarts", "Reset Cogs", "Disable Background", "Enable Background", "Get/Release Control", "Init AKLH", "Save AKLH", "Log Fuel Change", "Update Data Stream", "Init TenHz", "Read TenHz", "Remote Timer Reset", "Record Frequency Change", "Controller Change", "Get Alarms", "Init Alarms", "Save Alarms"]
            # "This case only happens when the previous read was before midnight and this reading is after midnight\n\nSo just want to get the file corrected to the proper date before saving this data set"
            n625 = Insert Into Array(array=w1528, index=0, new element=w1526) -> (w1527:T14[])
          }
          frame True {
            w1540 = "%d.1"
            # "Should possibly take the data from\nthe shift register and parse it out\nlike is done in the update screen case"
            n626 = local read "ControllerCurrent"() -> (w1569:dbl[])
            n627 = local read "Elapsed Time:"() -> (w1570:dbl[])
            n628 = local read "PumpCurrent"() -> (w1568:dbl[])
            n629 = local read "Pressure"() -> (w1567:dbl[])
            n630 = local read "Speed"() -> (w1565:dbl[])
            n631 = local read "Flow"() -> (w1566:dbl[])
            n632 = local read "Serial Numbers"() -> (w1536:T6)
            n633 = local read "PS Actual (V):"() -> (w1553:dbl)
            n634 = for {
              tunnel: w1570 -> [w1611] mode=indexing
              tunnel: w1569 -> [w1610] mode=indexing
              tunnel: w1568 -> [w1609] mode=indexing
              tunnel: w1567 -> [w1608] mode=indexing
              tunnel: w1566 -> [w1607] mode=indexing
              tunnel: w1565 -> [w1600] mode=indexing
              tunnel: [w1599] -> w1559 mode=indexing
              tunnel: [w1605] -> w1560 mode=indexing
              tunnel: [w1604] -> w1561 mode=indexing
              tunnel: [w1603] -> w1562 mode=indexing
              tunnel: [w1602] -> w1563 mode=indexing
              tunnel: [w1601] -> w1564 mode=indexing
              w1606 = "%d.2"
              n635 = Format Into String(format string="%<%H:%M:%S>t", w1611) -> (resulting string=w1601:string)  [unwired: 2 in, 1 out]
              n636 = Format Into String(format string=w1606, w1610) -> (resulting string=w1602:string)  [unwired: 2 in, 1 out]
              n637 = Format Into String(format string=w1606, w1609) -> (resulting string=w1603:string)  [unwired: 2 in, 1 out]
              n638 = Format Into String(format string=w1606, w1608) -> (resulting string=w1604:string)  [unwired: 2 in, 1 out]
              n639 = Format Into String(format string=w1606, w1607) -> (resulting string=w1605:string)  [unwired: 2 in, 1 out]
              n640 = Number To Decimal String(number=w1600) -> (decimal integer string=w1599:string)  [unwired: 1 in]
            }
            n641 = local read "Tank 1 Fuel Type"() -> (w1533:string)
            n642 = local read "Tank 2 Fuel Type"() -> (w1534:string)
            n643 = local read "Temp1"() -> (w1550:dbl)
            n644 = local read "Temp2"() -> (w1557:dbl)
            n645 = Number To Decimal String(number=w1555) -> (decimal integer string=w1542:string)  [unwired: 1 in]
            n646 = Number To Decimal String(number=w1554) -> (decimal integer string=w1543:string)  [unwired: 1 in]
            n647 = Format Into String(format string="%d.2", w1553) -> (resulting string=w1552:string)  [unwired: 2 in, 1 out]
            n648 = Format Into String(format string=w1540, w1550) -> (resulting string=w1551:string)  [unwired: 2 in, 1 out]
            n649 = Format Into String(format string=w1540, w1557) -> (resulting string=w1556:string)  [unwired: 2 in, 1 out]
            n650 = Cluster To Array(cluster=w1536) -> (array=w1535:string[])
            n651 = Build Array(w1556, w1534) -> (w1545:string[])
            n652 = Interleave 1D Arrays(w1535, w1564, w1563, w1562, w1561, w1560, w1559) -> (w1547:string[])
            n653 = Build Array(w1539, w1542, w1543, w1552, w1551, w1533) -> (w1549:string[])
            n654 = Insert Into Array(array=w1547, index=21, new element=w1545) -> (w1546:string[])
            n655 = disable-structure shown="Disabled" {
              frame Disabled {
                w1575 = 0 ("index")
                w1576 = i16 2 ("precision (6)")
                w1585 = i16 1 ("precision (6)")
                w1598 = 6 ("length")
                n656 = Array Subset(index=0, length=w1598) -> (array=w1593:dbl[], w1591:void[])
                n657 = Index Array(array=w1593, index=21) -> (element=w1592)
                n658 = Array Subset(array=w1593, index=22, length=w1598) -> (w1590:void[])
                n659 = Array Subset(array=w1593, index=28, length=w1598) -> (w1589:void[])
                n660 = Array Subset(array=w1593, index=w1598, length=w1598) -> (w1588:void[])
                n661 = Number To Fractional String(number=w1591, precision (6)=w1576) -> (F-format string=w1584:string[])  [unwired: 2 in]
                n662 = Number To Fractional String(number=w1590, precision (6)=w1585) -> (F-format string=w1583:string[])  [unwired: 2 in]
                n663 = Number To Fractional String(number=w1589, precision (6)=w1585) -> (F-format string=w1582:string[])  [unwired: 2 in]
                n664 = Number To Fractional String(number=w1588, width (-)=i16 4) -> (F-format string=w1581:string[])  [unwired: 2 in]
                n665 = Format Date/Time String(time format string (%c)="%H:%M:%S%2u") -> (seconds (now)=w1574:timestamp, date/time string=w1577:string)  [unwired: 1 in]
                n666 = Number To Fractional String(number=w1592, precision (6)=w1576) -> (F-format string=w1579:string)  [unwired: 2 in]
                n667 = Interleave 1D Arrays(w1584, w1583, w1582, w1581) -> (w1580:string[])
                n668 = Insert Into Array(array=w1580, index=w1575, new element=w1579) -> (w1578:string[])
                n669 = Insert Into Array(array=w1578, index=w1575, new element=w1577) -> ()  [unwired: 1 out]
              }
              frame Enabled {
              }
            }
            n670 = Insert Into Array(array=w1546, index=0, new element=w1549) -> (w1541:string[])
            n671 = Get Date/Time In Seconds() -> (seconds since 1Jan1904=w1532:timestamp)
            n672 = To Double Precision Float(number=w1532) -> (double precision float=w1531:dbl)
            n673 = call-poly <vilib>:"Write To Spreadsheet File.vi"("delimiter (\\t)"="," ("delimiter (\\t)"), "append to file? (new file:F)"=TRUE, "1D data"=w1541, "file path (dialog if empty)"=w1573) -> ("new file path (Not A Path if cancelled)"=w1538:path)  [unwired: 4 in]
          }
        }
        n674 = Bundle By Name(cluster=w1522, "AKLH Timer"=w1510, "AKLH Path"=w1516, "AKLH Last Hour"=w1509) -> (w1521:T17)
      }
      frame "Log Fuel Change" {
        n675 = Get Date/Time In Seconds() -> (seconds since 1Jan1904=w1620:timestamp)
        n676 = Format Date/Time String(time format string (%c)="%H:%M", seconds (now)=w1620) -> (date/time string=w1619:string)  [unwired: 1 in]
        n677 = Unbundle By Name(w1627) -> ("AKLH Path"=w1625:path)
        n678 = Replace Array Subset(array=string[] ["", "Fuel", "Changed"], new element=w1619, index=0) -> (w1616:string[])
        n679 = call-poly <vilib>:"Write To Spreadsheet File.vi"("delimiter (\\t)"="," ("delimiter (\\t)"), "append to file? (new file:F)"=TRUE, "1D data"=w1616, "file path (dialog if empty)"=w1625) -> ("new file path (Not A Path if cancelled)"=w1624:path)  [unwired: 4 in]
        n680 = Bundle By Name(cluster=w1627, "AKLH Path"=w1624) -> (w1626:T17)
        n681 = case shown="True" FALSE {
          tunnel: w1615 -> [w1628 w1632]
          tunnel: [w1628 w1631] -> w1614
          frame False {
          }
          frame True {
            w1629 = T14[] [enum."Remote Timer Reset"] items=["Main", "Init Files", "Init", "Save As", "Start Profile", "Check Step Time", "Alarm", "Run Step", "Stop Profile", "Cycle Reset", "Time Reset", "Time Reset All", "Time Set", "Tare CTs", "Save Profile", "Open Profile", "Get Profiles", "Update Screen", "Save Status", "Set Manual CMD", "Reset Restarts", "Reset Total Restarts", "Reset Cogs", "Disable Background", "Enable Background", "Get/Release Control", "Init AKLH", "Save AKLH", "Log Fuel Change", "Update Data Stream", "Init TenHz", "Read TenHz", "Remote Timer Reset", "Record Frequency Change", "Controller Change", "Get Alarms", "Init Alarms", "Save Alarms"]
            # "If tenhz is active I should have a way to insert\na line for fuel change... at the correct location"
            n682 = Insert Into Array(array=w1632, index=0, new element=w1629) -> (w1631:T14[])
          }
        }
      }
      frame "Update Data Stream" {
        # "...probably scrapping the idea of traces"
        # "UNACCESSIBLE"
        "Graph" <- dbl[] [] ("Waveform Graph 2")
      }
      frame "Init TenHz" {
        w1636 = string[] ["Time", "Position 1 Voltage (V)", "Position 2 Voltage (V)", "Position 3 Voltage (V)", "Position 4 Voltage (V)", "Position 5 Voltage (V)", "Position 6 Voltage (V)", "Power Supply Voltage (V)", "Position 1 Pump Current (A)", "Position 2 Pump Current (A)", "Position 3 Pump Current (A)", "Position 4 Pump Current (A)", "Position 5 Pump Current (A)", "Position 6 Pump Current (A)", "Position 1 Pump Speed (RPM)", "Position 2 Pump Speed (RPM)", "Position 3 Pump Speed (RPM)", "Position 4 Pump Speed (RPM)", "Position 5 Pump Speed (RPM)", "Position 6 Pump Speed (RPM)", "Position 1 Controller Current (A RMS)", "Position 2 Controller Current (A RMS)", "Position 3 Controller Current (A RMS)", "Position 4 Controller Current (A RMS)", "Position 5 Controller Current (A RMS)", "Position 6 Controller Current (A RMS)", "Tank 1 Temperature (Deg. C)", "Tank 2 Temperature (Deg. C)", "Position 1 Pressure (kPa)", "Position 2 Pressure (kPa)", "Position 3 Pressure (kPa)", "Position 4 Pressure (kPa)", "Position 5 Pressure (kPa)", "Position 6 Pressure (kPa)", "Position 1 Flow (L/H)", "Position 2 Flow (L/H)", "Position 3 Flow (L/H)", "Position 4 Flow (L/H)", "Position 5 Flow (L/H)", "Position 6 Flow (L/H)", "Position 1 Elapsed Time", "Position 2 Elapsed Time", "Position 3 Elapsed Time", "Position 4 Elapsed Time", "Position 5 Elapsed Time", "Position 6 Elapsed Time"]  # TenHz Header
        n683 = Unbundle By Name(w1651) -> ("TenHz Path"=w1661:path, "App Config.Location"=w1658:string, "App Config.CA Number"=w1657:string, "App Config.TenHzFrequency"=w1638:u32)
        n684 = Get Date/Time In Seconds() -> (seconds since 1Jan1904=w1655:timestamp)
        n685 = case shown="10, Default" w1638 {
          tunnel: ["One" "Two" "Three" "Four" "Five" "Six" "Seven" "Eight" "Nine" "Ten"] -> w1637
          frame 1 {
          }
          frame 2 {
          }
          frame 3 {
          }
          frame 4 {
          }
          frame 5 {
          }
          frame 6 {
          }
          frame 7 {
          }
          frame 8 {
          }
          frame 9 {
          }
          frame 10, Default {
          }
        }
        n686 = call "Timestamp2DayofYear.vi"("time stamp"=w1655) -> ("time string"=w1654:string)  [unwired: 14 in]
        n687 = Concatenate Strings(w1637, " Hertz Data " ("string"), w1658, " CA" ("string"), w1657, " " ("string"), w1654) -> (w1648:string)
        n688 = Strip Path(path=w1661) -> (stripped path=w1660:path)  [unwired: 1 out]
        n689 = Concatenate Strings(w1648, ".csv" ("string")) -> (w1652:string)
        n690 = Build Path(base path=w1660, name or relative path=w1652) -> (appended path=w1647:path)
        n691 = while {
          tunnel: w1648 -> [w1679]
          shift-right: [w1673] -> w1646
          shift-left: w1647 -> [w1672]
          i -> [w1678]
          stop <- w1674 continue-if-true
          n692 = call <vilib>:"Check if File or Folder Exists.vi"("path"=w1672) -> ("file or folder exists?"=w1676:bool, "dup path"=w1680:path)  [unwired: 8 in, 1 out]
          n693 = Add(x=2, y=w1678) -> (x+y=w1682:i32)
          n694 = Not Equal?(x=w1678, y=8) -> (x != y?=w1675:bool)
          n695 = case shown="True" w1676 {
            tunnel: w1680 -> [w1688 w1690]
            tunnel: [w1683 w1690] -> w1673
            tunnel: w1679 -> [w1686 _]
            tunnel: w1682 -> [w1685 _]
            frame True {
              n696 = Strip Path(path=w1688) -> (stripped path=w1689:path)  [unwired: 1 out]
              n697 = Format Into String(format string="%s_%d.csv", w1686, w1685) -> (resulting string=w1684:string)  [unwired: 2 in, 1 out]
              n698 = Build Path(base path=w1689, name or relative path=w1684) -> (appended path=w1683:path)
            }
            frame False {
            }
          }
          n699 = And(x=w1676, y=w1675) -> (x .and. y?=w1674:bool)
        }
        n700 = Get Date/Time In Seconds() -> (seconds since 1Jan1904=w1642:timestamp)
        n701 = Seconds To Date/Time(time stamp (now)=w1642) -> (date time rec=w1643:T34)  [unwired: 1 in]
        n702 = Unbundle By Name(w1643) -> ("day of month"=w1641:i32)
        n703 = call-poly <vilib>:"Write To Spreadsheet File.vi"("delimiter (\\t)"="," ("delimiter (\\t)"), "append to file? (new file:F)"=TRUE, "1D data"=w1636, "file path (dialog if empty)"=w1646) -> ("new file path (Not A Path if cancelled)"=w1640:path)  [unwired: 4 in]
        n704 = Bundle By Name(cluster=w1651, "TenHz Day"=w1641, "TenHz Path"=w1640) -> (w1650:T17)
        n705 = local write "TenHz Path"(w1640) -> ()
      }
      frame "Read TenHz" {
        (unwired) string[] ["AI-00/08_Voltage_1", "AI-01/09_Voltage_2", "AI-02/10_Voltage_3", "AI-03/11_Voltage_4", "AI-04/12_Voltage_5", "AI-05/13_Voltage_6", "AI-06_Spare", "AI-14_Spare", "AI-07_Spare", "AI-15_PS_Sense", "AI-16_Pump_Current_1", "AI-17_Pump_Current_2", "AI-18_Pump_Current_3", "AI-19_Pump_Current_4", "AI-20_Pump_Current_5", "AI-21_Pump_Current_6", "AI-16_Pump_Speed_1", "AI-17_Pump_Speed_2", "AI-18_Pump_Speed_3", "AI-19_Pump_Speed_4", "AI-20_Pump_Speed_5", "AI-21_Pump_Speed_6", "AI-22_Controller_Current_1", "AI-23_Controller_Current_2", "AI-24_Controller_Current_3", "AI-25_Controller_Current_4", "AI-26_Controller_Current_5", "AI-27_Controller_Current_6", "AI-28_Temperature_1", "AI-29_Temperature_2", "AI-30_Pump_Pressure_1", "AI-31_Pump_Pressure_2", "AI-32_Pump_Pressure_3", "AI-33_Pump_Pressure_4", "AI-34_Pump_Pressure_5", "AI-35_Pump_Pressure_6", "AI-36_Pump_Flow_1", "AI-37_Pump_Flow_2", "AI-38_Pump_Flow_3", "AI-39_Pump_Flow_4", "AI-40_Pump_Flow_5", "AI-41_Pump_Flow_6", "AI-42_Spare", "AI-43_Spare", "AI-44_Spare", "AI-45_Spare", "AI-46_Spare", "AI-47_Spare", "Pump_Elapsed_Time_1", "Pump_Elapsed_Time_2", "Pump_Elapsed_Time_3", "Pump_Elapsed_Time_4", "Pump_Elapsed_Time_5", "Pump_Elapsed_Time_6"]  # Channel Reference
        n706 = Unbundle By Name(w1720) -> ("Tank Data"=w1695:dbl[], "Controller List"=w1707:T11, "Trip Counters"=w1704:i32[], "Previous Times"=w1703:u32[], "Prev ON Times"=w1697:u32[], "Alarm Config"=w1708:T7, "App Config.Pumps Present"=w1710:u32, "Intitial Times"=w1731:dbl[], "Power Relay"=w1727:T2, "Manual CMDs"=w1711:dbl[], "App Config.Location"=w1726:string, "App Config.Current Profile"=w1725:string, "App Config.CA Number"=w1724:string, "PS CMD"=w1723:dbl, "Press CMD"=w1722:dbl, "Temp CMD"=w1721:dbl, "Run Profile"=w1712:bool, "App Config.Controller Type:"=w1706:T5)
        n707 = disable-structure shown="Enabled" {
          disable-tunnel: [w1737 w1742] -> w1709
          disable-tunnel: w1698 -> [_ w1743]
          disable-tunnel: w1695 -> [_ w1738]
          frame Disabled {
            n708 = call "Tank Data Global.vi"() -> ("Tank Data OUT"=w1737:dbl[])  [unwired: 11 in]
          }
          frame Enabled {
            n709 = xnode "Read/Write Control"("FPGA VI Reference In"=w1743) -> ("Currents (RMS)"=w1757:fxp<+,26,7>[], "Speed (RPM)"=w1758:fxp<+,32,18>[], "Temp"=w1759:fxp<+/-,20,12>, "Temp 2"=w1760:fxp<+/-,20,12>, "Elapsed Times"=w1761:u64[])  [unwired: 1 in, 2 out]
            n710 = To Double Precision Float(number=w1757) -> (double precision float=w1752:dbl[])
            n711 = To Double Precision Float(number=w1758) -> (double precision float=w1751:dbl[])
            n712 = To Double Precision Float(number=w1759) -> (double precision float=w1750:dbl)
            n713 = To Double Precision Float(number=w1760) -> (double precision float=w1749:dbl)
            n714 = To Double Precision Float(number=w1761) -> (double precision float=w1741:dbl[])
            n715 = Replace Array Subset(array=w1738, new element=w1752, index=10) -> (w1756:dbl[])
            n716 = Replace Array Subset(array=w1756, new element=w1751, index=16) -> (w1755:dbl[])
            n717 = Replace Array Subset(array=w1755, new element=w1750, index=28) -> (w1754:dbl[])
            n718 = Replace Array Subset(array=w1754, new element=w1749, index=29) -> (w1753:dbl[])
            n719 = Divide(x=w1741, y=10000) -> (x/y=w1739:dbl[])
            n720 = Replace Array Subset(array=w1753, new element=w1739, index=48) -> (w1742:dbl[])
          }
        }
        n721 = Index Array(array=w1707, index=w1706) -> (element=w1705:T12)
        n722 = case shown="\"Kuhnke\", Default" w1706 {
          tunnel: [100 ("CMD Max") 1000 ("CMD Max")] -> w1715
          tunnel: [1 ("CMD Max") 10 ("CMD Max")] -> w1714
          frame "Kuhnke", Default {
          }
          frame "Conti" {
          }
        }
        n723 = Number To Boolean Array(number=w1710) -> (Boolean array=w1730:bool[])
        n724 = call "Signal Breakout.vi"("Pumps Enabled"=w1730, "Tank Data"=w1709, "Intitial Times"=w1731) -> ("Pump Data"=w1729:T20, "Tank Data"=w1728:T36)  [unwired: 10 in, 1 out]
        n725 = Bundle("Location"=w1726, "Current Profile"=w1725, "CA Number"=w1724) -> (w1733:T37)  [unwired: 1 in]
        n726 = Bundle("PS CMD"=w1723, "Press CMD"=w1722, "Temp CMD"=w1721) -> (w1732:T38)  [unwired: 1 in]
        n727 = Bundle By Name(cluster=T24 {"Controller List"="", "Controller Type:"=enum."Kuhnke", "CMD Max"=0, "CMD Inc"=0} ("Controller Config"), "Controller Type:"=w1706, "CMD Max"=w1715, "CMD Inc"=w1714) -> (w1716:T24)
        n728 = call "Evaluate Alarms.vi"("In Test"=w1712, "Controller"=w1705, "Alarm Config"=w1708, "Data"=w1709, "Pumps Present"=w1710, "Trip Counter"=w1704, "Previous Times"=w1703, "Manual CMDs"=w1711, "Prev ON Times"=w1697) -> ("Trip Counter OUT"=w1702:i32[], "Previous Times OUT"=w1701:u32[], "Alarm Tripped"=w1700:bool, "Alarm Message"=w1699:string, "Prev ON Times OUT"=w1696:u32[])  [unwired: 14 in]
        n729 = Bundle By Name(cluster=T23 {"Start Test"=FALSE, "Toggle Spare 1"=FALSE, "Toggle Spare 2"=FALSE, "Toggle Spare 3"=FALSE, "Toggle Spare 4"=FALSE, "Toggle Spare 5"=FALSE} ("HMI Tog Buttons"), "Start Test"=w1712) -> (w1718:T23)
        n730 = call "RPi HMI Com.vi"("Pump Data"=w1729, "Tank Data"=w1728, "Power Relays"=w1727, "Pump CMDs"=w1711, "HMI Header"=w1733, "Tank CMDs"=w1732, "HMI Tog Buttons"=w1718, "RPi HMI Mode"=RPi_HMI_Mode."Write Data", "In Test"=w1712, "Controller Config"=w1716) -> ()  [unwired: 9 in, 1 out]
        n731 = Tick Count (ms)() -> (millisecond timer value=w1694:u32)
        n732 = Get Date/Time In Seconds() -> (seconds since 1Jan1904=w1736:timestamp)
        n733 = feedback-in #2(w1694) -> ()
        n734 = feedback #2() -> (w1693:u32)  [unwired: 1 in]
        n735 = To Double Precision Float(number=w1736) -> (double precision float=w1713:dbl)
        n736 = Subtract(x=w1694, y=w1693) -> (x-y=w1692:u32)
        n737 = Bundle By Name(cluster=w1720, "TenHz Timer"=w1713, "Tank Data"=w1709, "Trip Counters"=w1702, "Previous Times"=w1701, "Alarm"=w1700, "Alarm Message"=w1699, "Prev ON Times"=w1696) -> (w1735:T17)
        n738 = flat-sequence {
          tunnel: w1692 -> [_]
          frame #0 {
          }
        }
      }
      frame "Record Frequency Change" {
        # "was switching in the globals for controlling the logging of \"tenhz\""
        # "60 seconds times 7 min recording period and decremented to point at the correct index"
        n739 = local read "Record Frequency:"() -> (w1771:i32)
        n740 = Multiply(x=w1771, y=420) -> (x*y=w1768:i32)
        n741 = case shown="10, Default" w1771 {
          tunnel: [u32 1000 ("milliseconds to wait") u32 500 ("milliseconds to wait") u32 333 ("milliseconds to wait") u32 250 ("milliseconds to wait") u32 200 ("milliseconds to wait") u32 167 ("milliseconds to wait") u32 143 ("milliseconds to wait") u32 125 ("milliseconds to wait") u32 111 ("milliseconds to wait") u32 100 ("milliseconds to wait")] -> w1766
          frame 1 {
          }
          frame 2 {
          }
          frame 3 {
            # "0.1% slow"
          }
          frame 4 {
          }
          frame 5 {
          }
          frame 6 {
            # "0.2% fast"
          }
          frame 7 {
            # "0.1% fast"
          }
          frame 8 {
          }
          frame 9 {
            # "0.1% slow"
          }
          frame 10, Default {
          }
        }
        n742 = Decrement(x=w1768) -> (x-1=w1767:i32)
        n743 = global write "Record Period (global).vi" "Record Period (ms)"(w1766) -> ()
        n744 = global write "Record Samples (global).vi" "Record Samples"(w1767) -> ()
      }
      frame "Controller Change" {
        n745 = flat-sequence {
          tunnel: [w1812] -> w1787
          tunnel: [w1811] -> w1786
          tunnel: [w1797] -> w1783
          tunnel: w1784 -> [w1798]
          tunnel: w1785 -> [w1806]
          tunnel: w1784 -> [w1810]
          tunnel: w1787 -> [w1839]
          tunnel: w1786 -> [w1828]
          frame #0 {
            w1793 = dbl[] [0.0, 0.0, 0.0, 0.0, 0.0, 0.0] ("ControllerCurrent")
            n746 = Unbundle By Name(w1810) -> ("Controller List"=w1790:T11, "App Config.Controller Type:"=w1796:T5)
            n747 = Index Array(array=w1790, index=w1796) -> (element=w1792:T12)
            n748 = Unbundle By Name(w1792) -> ("Frequency"=w1794:i32, "CommSeg"=w1795:i32, "Controller?"=w1811:bool, "High Command"=w1800:dbl, "Low Command"=w1801:dbl, "Command Step"=w1802:dbl, "Stop Command"=w1803:dbl, "Invert PWM"=w1791:bool, "Controller Name"=w1789:T5)
            n749 = Equal?(x=2, y=w1795) -> (x = y?=w1812:bool)
            n750 = case shown="False" w1812 {
              tunnel: [w1823 fxp<+,32,16> 1.0 ("CommFactor")] -> w1808
              tunnel: w1795 -> [w1824 _]
              frame False {
                n751 = case shown="10, Default" w1824 {
                  tunnel: [fxp<+,32,16> 4.0 ("CommFactor") fxp<+,32,16> 5.0 ("CommFactor")] -> w1823
                  frame 8 {
                  }
                  frame 10, Default {
                  }
                }
              }
              frame True {
              }
            }
            n752 = property on="ControllerCurrent" class="Arr (strict)"("Value"=w1793) -> ()  [unwired: 2 in, 2 out]
            n753 = local write "ControllerCurrent"(w1793) -> ()
            n754 = Divide(x=40000000.0 ("40 MHz"), y=w1794) -> (x/y=w1805:dbl)
            n755 = To Unsigned Long Integer(number=w1805) -> (unsigned 32bit integer=w1799:u32)
            n756 = disable-structure shown="Enabled" {
              disable-tunnel: w1812 -> [w1818 _]
              disable-tunnel: w1808 -> [w1817 _]
              disable-tunnel: "RPMhyst" -> [w1816 w1819]
              disable-tunnel: w1806 -> [w1815 w1822]
              disable-tunnel: w1799 -> [w1814 w1821]
              disable-tunnel: w1791 -> [w1813 _]
              disable-tunnel: w1789 -> [_ w1820]
              frame Disabled {
                n757 = xnode "Read/Write Control"("FPGA VI Reference In"=w1815, "Brushless"=w1818, "CommFactor"=w1817, "RPMhyst"=w1816, "PWM Period (Ticks)"=w1814, "InvertPWM?"=w1813) -> ()  [unwired: 1 in, 2 out]
              }
              frame Enabled {
                n758 = xnode "Read/Write Control"("FPGA VI Reference In"=w1822, "Speed Hysteresis"=w1819, "PWM Period (Ticks)"=w1821, "Controller Type:"=w1820) -> ()  [unwired: 2 in, 2 out]
              }
            }
            n759 = property on="Numeric" class="DigNum (strict)"("Maximum"=w1800, "Minimum"=w1801, "Increment"=w1802) -> ()  [unwired: 2 in, 2 out]
            n760 = Bundle By Name(cluster=w1798, "Stop Cmd"=w1803, "Controller"=w1792) -> (w1797:T17)
          }
          frame #1 {
            # "This should be controlled by the\nDip switch and chosen as the\ndata set not set by pump type"
            n761 = Select(t="Controller\nVoltage\n(V)" ("Caption.Text"), s=FALSE, f="Pump\nVoltage\n(V)" ("Caption.Text")) -> (s? t:f=w1832:string)
            n762 = Select(t="Pump\nCurrent\n(RMS)" ("Label.Text"), s=w1839, f="Pump\nCurrent\n(DC)" ("Label.Text")) -> (s? t:f=w1834:string)
            n763 = Select(t=T27."Enabled" ("Disabled"), s=w1828, f=T27."Disabled and Grayed Out" ("Disabled")) -> (s? t:f=w1835:T27)
            n764 = property on="Voltages" class="Arr (strict)"("Caption.Text"=w1832) -> ()  [unwired: 2 in, 2 out]
            n765 = property on="PumpCurrent" class="Arr (strict)"("Caption.Text"=w1834) -> ()  [unwired: 2 in, 2 out]
            n766 = property on="ControllerCurrent" class="Arr (strict)"("DisabledEnum"=w1835) -> ()  [unwired: 2 in, 2 out]
          }
        }
      }
    }
  }
  n767 = while {
    shift-right: [w1847] -> _
    shift-left: w1 -> [w1848]
    shift-right: [w1845] -> _
    shift-left: dbl[] [0.0, 0.0, 0.0, 0.0, 0.0, 0.0, 0.0, 0.0, 0.0, 0.0, 0.0, 0.0, 0.0, 0.0, 0.0, 0.0, 0.0, 0.0, 0.0, 0.0, 0.0, 0.0, 0.0, 0.0, 0.0, 0.0, 0.0, 0.0, 0.0, 0.0, 0.0, 0.0, 0.0, 0.0, 0.0, 0.0, 0.0, 0.0, 0.0, 0.0, 0.0, 0.0, 0.0, 0.0, 0.0, 0.0, 0.0] -> [w1843]
    shift-right: [w1846] -> _
    shift-left: 0 -> [w1844]
    tunnel: w4 -> [_]
    shift-right: [w1841] -> _
    shift-left: _ -> [w1840]
    stop <- FALSE stop-if-true
    n768 = local read "pb.TenHzSave"() -> (w1842:bool)
    n769 = case shown="True" w1842 {
      tunnel: w1848 -> [w1856 w1890]
      tunnel: [w1856 w1888] -> w1847
      tunnel: [0 w1887] -> w1846
      tunnel: [w1854 w1857] -> w1845
      tunnel: w1844 -> [_ w1886]
      tunnel: w1843 -> [w1854 w1885]
      tunnel: [w1851 w1876] -> w1841
      tunnel: w1840 -> [_ w1875]
      frame False {
        n770 = Get Date/Time In Seconds() -> (seconds since 1Jan1904=w1850:timestamp)
        n771 = Seconds To Date/Time(time stamp (now)=w1850) -> (date time rec=w1852:T34)  [unwired: 1 in]
        n772 = Wait (ms)(milliseconds to wait=u32 10000) -> ()  [unwired: 1 out]
        n773 = Unbundle By Name(w1852) -> ("day of month"=w1851:i32)
      }
      frame True {
        n774 = Get Date/Time In Seconds() -> (seconds since 1Jan1904=w1879:timestamp)
        n775 = global read "Record Period (global).vi" "Record Period (ms)"() -> (w1881:u32)
        n776 = To Double Precision Float(number=w1879) -> (double precision float=w1883:dbl)
        n777 = Seconds To Date/Time(time stamp (now)=w1879) -> (date time rec=w1880:T34)  [unwired: 1 in]
        n778 = Replace Array Subset(array=w1885, new element=w1883, index=0) -> (w1859:dbl[])
        n779 = Unbundle By Name(w1880) -> ("day of month"=w1876:i32)
        n780 = call "Tank Data Global.vi"() -> ("Tank Data OUT"=w1858:dbl[])  [unwired: 11 in]
        n781 = Wait (ms)(milliseconds to wait=w1881) -> ()  [unwired: 1 out]
        n782 = Array Subset(array=w1858, index=0, length=6) -> (w1862:dbl[])
        n783 = Not Equal?(x=w1876, y=w1875) -> (x != y?=w1874:bool)
        n784 = Replace Array Subset(array=w1859, new element=w1862, index=1) -> (w1872:dbl[])
        n785 = Array Subset(array=w1858, index=9, length=33) -> (w1863:dbl[])
        n786 = global read "Record Samples (global).vi" "Record Samples"() -> (w1882:i32)
        n787 = Replace Array Subset(array=w1872, new element=w1863, index=7) -> (w1873:dbl[])
        n788 = Array Subset(array=w1858, index=48, length=6) -> (w1868:dbl[])
        n789 = Replace Array Subset(array=w1873, new element=w1868, index=40) -> (w1857:dbl[])
        n790 = Equal?(x=w1886, y=w1882) -> (x = y?=w1878:bool)
        n791 = Replace Array Subset(array=w1890, new element=w1857, index (row)=w1886) -> (w1889:dbl[][])  [unwired: 1 in]
        n792 = Or(x=w1878, y=w1874) -> (x .or. y?=w1877:bool)
        n793 = case shown="True" w1877 {
          tunnel: w1889 -> [w1893 w1894]
          tunnel: [w1893 dbl[][] array4200x47[197400 elements]] -> w1888
          tunnel: [w1892 0] -> w1887
          tunnel: w1886 -> [w1891 w1897]
          tunnel: w1874 -> [_ w1899]
          frame False {
            n794 = Increment(x=w1891) -> (x+1=w1892:i32)
          }
          frame True {
            n795 = Boolean To (0,1)(Boolean=w1899) -> (0, 1=w1898:i16)
            n796 = Negate(x=w1898) -> (-x=w1896:i16)
            n797 = Add(x=w1897, y=w1896) -> (x+y=w1895:i32)
            n798 = stacked-sequence {
              tunnel: w1895 -> [w1902 _]
              tunnel: w1894 -> [_ w1903]
              frame #0 {
                "TenHzPts" <- w1902
              }
              frame #1 {
                n799 = global write "TenHzDataArray(Global).vi" "TenHzDataArray"(w1903) -> ()
              }
            }
          }
        }
      }
    }
  }
  n800 = global write "TenHzDataArray(Global).vi" "TenHzDataArray"(w1) -> ()
  n801 = while {
    stop <- FALSE stop-if-true
    n802 = property class="App"() -> ("RemotePanel.ConnToClients"=w1908:T39)  [unwired: 2 in, 2 out]
    n803 = Array Size(array=w1908) -> (size(s)=w1911:i32)
    n804 = Greater Than 0?(x=w1911) -> (x > 0?=w1904:bool)
    "Client?" <- w1904
    n805 = Wait (ms)(milliseconds to wait=u32 500) -> ()  [unwired: 1 out]
    n806 = feedback #3() -> (w1910:bool)  [unwired: 1 in]
    n807 = feedback-in #3(w1904) -> ()
    n808 = Greater?(x=w1910, y=w1904) -> (0:w1909:bool)
    n809 = call <vilib>:"RT Get CPU Loads.vi"() -> ("CPU loads"=w1906:T40[])  [unwired: 10 in, 1 out]
    n810 = case shown="True" w1909 {
      frame False {
      }
      frame True {
        n811 = local write "Login"(FALSE ("Login")) -> ()
      }
    }
    n812 = Index Array(array=w1906) -> (element=w1907:T40)  [unwired: 1 in]
    n813 = Unbundle By Name(w1907) -> ("Total (%)"=→"CPU Usage:":dbl)
    n814 = case shown="True" w1904 {
      frame False {
        n815 = property class="App"("WebSrvr.TCPAccessList"=string[] ["c+*"] ("Web Server:TCP/IP Access List")) -> ()  [unwired: 2 in, 2 out]
      }
      frame True {
        n816 = property class="App"("WebSrvr.TCPAccessList"=string[] ["-*"] ("Web Server:TCP/IP Access List")) -> ()  [unwired: 2 in, 2 out]
      }
    }
  }
  n817 = while {
    shift-right: [w1923] -> _
    shift-left: _ -> [w1924]
    tunnel: w4 -> [_]
    stop <- FALSE stop-if-true
    w1921 = 0 ("index (row)")
    n818 = global read "TenHzDataArray(Global).vi" "TenHzDataArray"() -> (w1920:dbl[][])
    n819 = local read "pb.TenHzSave"() -> (w1919:bool)
    n820 = Wait (ms)(milliseconds to wait=u32 10000) -> ()  [unwired: 1 out]
    n821 = Index Array(array=w1920, index (row)=w1921, index (col)=w1921) -> (element=w1923:dbl)
    n822 = Not Equal?(x=w1923, y=w1924) -> (x != y?=w1918:bool)
    n823 = And(x=w1918, y=w1919) -> (x .and. y?=w1917:bool)
    n824 = case shown="True" w1917 {
      tunnel: w1920 -> [_ w1928]
      frame False {
      }
      frame True {
        n825 = local read "TenHzPts"() -> (w1926:i32)
        n826 = Increment(x=w1926) -> (x+1=w1927:i32)
        n827 = Array Subset(array=w1928, index (row)=0 ("index"), length (row)=w1927) -> (w1929:dbl[][])  [unwired: 2 in]
        n828 = call-poly <vilib>:"Write To Spreadsheet File.vi"("delimiter (\\t)"="," ("delimiter (\\t)"), "append to file? (new file:F)"=TRUE, "2D data"=w1929, "file path (dialog if empty)"="TenHz Path") -> ()  [unwired: 4 in, 1 out]
      }
    }
  }
  n829 = disable-structure shown="Disabled" {
    frame Disabled {
      w1934 = dbl[] [0.0, 0.0, 0.0, 0.0, 0.0, 0.0]  # Manual PWMs
      # "Don't know why this was sitting here"
      n830 = local write "Manual\nCMD"(w1934) -> ()
    }
    frame Enabled {
    }
  }
